vi "ADC_CHP_TEST.vi"() -> ()   [LabVIEW 2016]
uses:
  D:/share/SBND/SBND_SW/SBND_WIB_DLL/WIB_DLL/bin/Debug/WIB_DLL.dll
  SBND/SBND_SW/SBND_WIB_DLL/WIB_DLL/bin/Debug/WIB_DLL.dll
  WIB_Global.vi
  <vilib>/express/express analysis/Spectral/Block/exnSpectralBlock spectral measurements peak poly.vi
  <vilib>/express/express analysis/Spectral/Block/exnSpectralBlock spectral measurements peak DDT.vi
  <vilib>/Waveform/DTblOps.llb/DTbl Boolean Array to Digital.vi
  <vilib>/Waveform/DTblOps.llb/DTbl Append Digital Samples.vi
  <vilib>/express/express analysis/Spectral/XNode/ExpressSpectralMeasurementsBlockNode.xnode
  <vilib>/Analysis/NI_AAL_SigProc.lvlib
panel:
  out "PWR_CNTRL_\nREG 1":u32=15
  out "HCP_CHN_SEL_REG3":u32=2147484929
  out "TP_FR_DLY_REG5":u32=7996092
  out "D SHIFT_REG8":u32=33686018
  out "TP_CNTL_REG6":u32=18
  out "CLK_PHS_REG7":u32=13
  out "FE SPI":u32[](array[numeric])=[3435973836, 3435973836, 3435973836, 3435973836, 35344]
  out "ADC SPI 4":u32[](array[numeric])=[1751672936, 1751672936, 1751672936, 1751672936, 40960]
  out "ADC SPI 3":u32[](array[numeric])=[1751672936, 1751672936, 1751672936, 1751672936, 40960]
  out "ADC SPI 2":u32[](array[numeric])=[1751672936, 1751672936, 1751672936, 1751672936, 40960]
  out "ADC SPI 1":u32[](array[numeric])=[1751672936, 1751672936, 1751672936, 1751672936, 40960]
  out "receive_byte_array":u8[](array[numeric])=[1, 179, 4, 188, 0, 0, 0, 0, 0, 0, 0, 0, 240, 0, 1, 0, 250, 206, 195, 197, 161, 60, 60, 163, 51, 170, 192, 60, 61, 131, 195, 192, 200, 60, 57, 227, 83, 192, 203, 61, 60, 35, 250, 206, 163, 197, 159, 60, 60, 131, 51, 172, 187, 60, 61, 115, 195, 192, 200, 60, 57, 227, 83, 188, 203, 61, 60, 19, 250, 206, 179, 198, 162, 60, 60, 3, 51, 172, 188, 60, 61, 147, 179, 192, 200, 60, 57, 243, 83, 192, 203, 61, 60, 3, 250, 206, 163, 197, 164, 60, 60, 163, 99, 173, 192, 60, 61, 163, 179, 192, 201, 60, 57, 227, 99, 191, 203, 61, 60, 19, 250, 206, 179, 195, 164, 60, 60, 147, 51, 168, 192, 60, 61, 99, 131, 192, 200, 60, 57, 227, 51, 192, 205, 61, 60, 3, 250, 206, 163, 194, 161, 60, 60, 99, 35, 169, 189, 60, 61, 99, 147, 189, 200, 60, 57, 227, 99, 187, 203, 61, 60, 3, 250, 206, 147, 192, 159, 60, 60, 51, 51, 167, 187, 60, 61, 99, 147, 192, 200, 60, 57, 227, 83, 187, 204, 61, 60, 19, 250, 206, 147, 192, 159, 60, 60, 51, 19, 170, 190, 60, 61, 99, 179, 192, 198, 60, 57, 211, 83, 186, 203, 61, 60, 3, 250, 206, 115, 193, 158, 60, 60, 67, 19, 170, 186, 60, 61, 115, 163, 187, 200, 60, 57, 227, 83, 185, 203, 61, 60, 3, 250, 206, 131, 192, 158, 60, 60, 51, 3, 170, 186, 60, 61, 99, 163, 188, 200, 60, 58, 19, 83, 186, 203, 61, 60, 3, 250, 206, 163, 193, 159, 60, 60, 115, 3, 169, 187, 60, 61, 99, 163, 187, 200, 60, 57, 243, 51, 187, 200, 61, 60, 3, 250, 206, 179, 192, 159, 60, 60, 115, 3, 167, 188, 60, 61, 67, 179, 187, 200, 60, 57, 227, 51, 187, 200, 61, 60, 3, 250, 206, 195, 193, 162, 60, 60, 115, 19, 167, 192, 60, 61, 99, 131, 187, 199, 60, 58, 3, 115, 185, 202, 61, 60, 3, 250, 206, 163, 192, 191, 60, 60, 115, 19, 167, 192, 60, 61, 83, 147, 187, 199, 60, 57, 243, 51, 187, 203, 61, 60, 3, 250, 206, 179, 193, 159, 60, 60, 115, 19, 170, 192, 60, 61, 115, 131, 187, 197, 60, 57, 227, 51, 185, 202, 61, 59, 195, 250, 206, 179, 194, 160, 60, 60, 99, 3, 171, 192, 60, 61, 99, 131, 185, 200, 60, 57, 243, 51, 188, 200, 61, 60, 3, 250, 206, 179, 196, 160, 60, 60, 99, 3, 171, 192, 60, 61, 115, 163, 184, 198, 60, 57, 211, 83, 185, 200, 61, 60, 3, 250, 206, 163, 196, 159, 60, 60, 99, 3, 167, 192, 60, 61, 99, 131, 187, 198, 60, 57, 211, 51, 187, 200, 61, 60, 3, 250, 206, 163, 196, 161, 60, 60, 99, 3, 170, 187, 60, 61, 99, 147, 185, 198, 60, 57, 195, 35, 188, 200, 61, 60, 3, 250, 206, 131, 196, 160, 60, 60, 115, 3, 168, 192, 60, 61, 99, 131, 186, 197, 60, 57, 227, 35, 188, 200, 61, 59, 227, 250, 206, 163, 195, 160, 60, 60, 115, 3, 170, 189, 60, 61, 67, 147, 186, 197, 60, 57, 243, 35, 191, 200, 61, 59, 195, 250, 206, 131, 194, 161, 60, 60, 131, 3, 168, 192, 60, 61, 99, 131, 184, 198, 60, 57, 243, 19, 188, 201, 61, 60, 3, 250, 206, 131, 193, 159, 60, 60, 163, 3, 167, 192, 60, 61, 67, 115, 185, 198, 60, 57, 227, 19, 188, 200, 61, 59, 195, 250, 206, 67, 188, 154, 60, 60, 51, 3, 163, 185, 60, 61, 51, 83, 179, 194, 60, 57, 163, 211, 185, 198, 60, 59, 131, 250, 206, 179, 97, 64, 54, 54, 163, 83, 72, 98, 54, 55, 163, 195, 76, 104, 54, 52, 3, 35, 92, 106, 55, 53, 243, 250, 206, 242, 53, 23, 35, 35, 226, 2, 29, 54, 36, 36, 226, 162, 16, 52, 36, 33, 82, 242, 40, 61, 35, 35, 66, 250, 206, 49, 0, 213, 15, 15, 48, 160, 212, 241, 14, 16, 16, 48, 206, 247, 15, 13, 128, 0, 222, 0, 16, 14, 225, 250, 206, 32, 220, 64, 9, 5, 96, 32, 64, 123, 4, 5, 240, 64, 66, 200, 5, 5, 240, 144, 64, 158, 8, 8, 96, 250, 206, 160, 218, 40, 8, 3, 240, 208, 13, 117, 2, 3, 240, 112, 54, 201, 4, 5, 144, 32, 35, 155, 8, 8, 0, 250, 206, 192, 218, 43, 8, 3, 240, 240, 10, 119, 2, 3, 240, 128, 54, 200, 4, 5, 144, 16, 35, 155, 8, 8, 0, 250, 206, 0, 218, 60, 9, 3, 240, 96, 22, 120, 4, 3, 240, 48, 85, 201, 5, 5, 240, 128, 56, 155, 8, 8, 32, 250, 206, 192, 230, 171, 12, 12, 224, 240, 167, 203, 11, 14, 32, 96, 231, 230, 12, 12, 0, 16, 191, 216, 14, 12, 208, 250, 206, 225, 156, 123, 25, 25, 209, 113, 124, 152, 25, 27, 65, 161, 193, 176, 25, 24, 33, 65, 157, 161, 27, 25, 129, 250, 206, 98, 115, 75, 39, 39, 18, 210, 81, 106, 38, 40, 162, 34, 145, 127, 39, 37, 34, 194, 113, 118, 40, 38, 178, 250, 206, 131, 23, 236, 49, 49, 98, 2, 244, 11, 49, 50, 83, 83, 40, 32, 49, 47, 3, 131, 16, 26, 50, 48, 179, 250, 206, 3, 121, 81, 56, 55, 179, 67, 90, 110, 55, 56, 131, 179, 128, 129, 55, 53, 51, 211, 113, 128, 56, 54, 243, 250, 206, 227, 172, 132, 58, 58, 227, 67, 144, 162, 58, 59, 163, 211, 165, 174, 58, 56, 99, 3, 162, 176, 60, 58, 83, 250, 206, 67, 191, 154, 60, 60, 83, 227, 163, 182, 59, 61, 3, 67, 182, 195, 60, 57, 147, 3, 183, 196, 61, 59, 147, 250, 206, 147, 195, 159, 60, 60, 131, 19, 170, 187, 60, 61, 99, 131, 184, 201, 60, 57, 243, 83, 188, 200, 61, 60, 19] format="%x"
  out "ADC_hist":u32[][](array[numeric])
  in  "stop":bool
  in  "Tab Control":T1(tab)
  in  "RESET 6":bool
  in  "samples 3":i32
  in  "CHANNEL":u8(slide)=5
  in  "number_of_samples":u32=5000
  in  "CHIP":u8(slide)=1 scale=1.0..4.0
  in  "STOP_DATA":bool
  in  "AUTO SCALE":bool=TRUE
  in  "x":u32=72
  out "ADC_RMS":dbl=174.66413482178115
  out "ADC_MEAN":dbl=933.1157768446311
  out "ADC_CNT":u32=5001
  out "ADC_PEAK":u32=936
  out "Waveform Graph 4":u32[](graph)
  out "ADC HIST":u32[](graph)=[22577709, 0, 0, 0, 0, 0, 0, 21, 20418, 52548, 15639, 26748, 664, 1, 0, 1, 0, 0, 0, 0, 0, 0, 0, 0, 0, 0, 0, 0, 0, 0, 0, 0, 2, 0, 0, 0, 1, 7, 281, 204, 1416, 4249, 8417, 5754, 234, 46, 11, 23, 1, 0, 0, 1, 16, 23, 186, 61, 3216, 3846, 273, 944, 1470, 230, 5, 52, 23468, 0, 0, 0, 0, 0, 0, 2, 26, 205, 1131, 2487, 13823, 43022, 52991, 115617, 146273, 179719, 290128, 262476, 337032, 260069, 167100, 269246, 193925, 64886, 36955, 23917, 16001, 9314, 5817, 3963, 4270, 8627, 9126, 11227, 16105, 15657, 10840, 8925, 8975, 10027, 6845, 7402, 7674, 7135, 5371, 4730, 3238, 2959, 2574, 3198, 3582, 4566, 5614, 6190, 5902, 5590, 4229, 3018, 2633, 2873, 3587, 558800, 539267, 12817, 2, 0, 1, 0, 1, 78, 70, 55, 3, 0, 0, 0, 0, 0, 0, 0, 0, 0, 0, 0, 0, 0, 0, 28247, 761, 0, 0, 0, 0, 0, 3, 0, 0, 0, 0, 0, 1, 1, 61, 181, 563, 3580, 2716, 1620, 768, 580, 227, 15, 5, 3, 0, 7, 11, 25, 31, 40, 79, 98, 174, 226, 331, 157971, 146461, 0, 0, 0, 0, 0, 0, 0, 0, 0, 0, 0, 0, 0, 0, 0, 20, 1, 6, 75, 297, 1597, 1813, 2654, 2380, 744, 706, 26, 2, 0, 1, 1, 0, 0, 0, 0, 0, 0, 0, 0, 0, 17, 7, 0, 0, 0, 0, 0, 0, 0, 0, 0, 0, 0, 0, 0, 0, 0, 0, 0, 0, 0, 0, 268190, 65267, 235, 280, 239, 116, 42, 12, 1, 0, 1, 0, 0, 0, 0, 0, 0, 0, 0, 0, 0, 0, 0, 0, 0, 3, 0, 27989, 1018, 0, 0, 0, 0, 0, 0, 0, 0, 0, 0, 0, 0, 0, 0, 0, 0, 0, 0, 0, 0, 0, 0, 0, 0, 0, 0, 0, 0, 0, 0, 0, 0, 0, 0, 0, 348357, 468088, 0, 0, 0, 0, 0, 0, 0, 0, 0, 0, 0, 0, 0, 0, 0, 0, 0, 0, 0, 0, 0, 0, 0, 0, 0, 0, 0, 0, 0, 0, 0, 0, 0, 0, 0, 0, 0, 0, 0, 0, 0, 0, 0, 0, 0, 0, 0, 1, 0, 0, 10, 44, 151, 270, 186, 1592, 3714, 1087, 1445, 1789, 402, 33, 114418, 100521, 0, 0, 0, 0, 0, 0, 0, 0, 0, 0, 0, 0, 0, 0, 0, 0, 0, 0, 0, 0, 0, 0, 0, 0, 0, 0, 0, 0, 0, 0, 0, 0, 0, 0, 0, 0, 0, 0, 0, 0, 0, 0, 0, 0, 0, 0, 0, 0, 0, 0, 0, 0, 0, 0, 0, 0, 0, 0, 0, 0, 0, 0, 103225, 65211, 0, 0, 0, 0, 0, 0, 0, 0, 0, 0, 0, 0, 0, 0, 0, 0, 0, 0, 0, 1, 0, 0, 0, 0, 2, 474, 23148, 5367, 21546, 7315, 162, 0, 0, 0, 0, 0, 0, 0, 0, 0, 0, 0, 0, 0, 0, 0, 0, 0, 0, 0, 0, 0, 0, 0, 0, 0, 0, 0, 0, 0, 0, 0, 543916, 110849, 0, 0, 0, 0, 0, 0, 0, 0, 0, 0, 0, 0, 0, 0, 0, 64, 0, 8, 41, 168, 805, 1642, 2596, 1966, 752, 2266, 66, 39, 4270076, 0, 1, 0, 0, 0, 0, 0, 0, 0, 0, 0, 0, 0, 0, 0, 0, 0, 0, 0, 0, 0, 0, 0, 0, 0, 0, 0, 0, 0, 0, 0, 0, 0, 37524, 27901, 0, 0, 0, 0, 6, 10, 48, 66, 332, 550, 1805, 2923, 1144, 2250, 391, 902, 209, 44, 11, 0, 0, 0, 0, 3, 4281, 672, 89, 36472, 1510, 7, 15, 0, 9, 17, 33, 68, 41, 14, 5, 2, 0, 0, 0, 0, 0, 0, 0, 0, 0, 0, 0, 0, 0, 1, 12, 29, 38, 40, 16, 8, 6, 1, 186208, 374158, 15, 0, 0, 0, 0, 0, 5, 16, 34, 29, 14, 23, 14, 16, 33, 31, 18, 12, 3, 0, 0, 0, 0, 3, 0, 8, 21677, 7388, 152, 229, 257, 251, 134, 170, 204, 245, 307, 103, 52, 23, 7, 0, 0, 0, 3, 8, 35, 36, 38, 20, 10, 1, 0, 1, 11, 34, 72, 83, 40, 34, 5, 3, 539938, 221066, 133, 2, 14, 18, 29, 37, 423, 8, 8, 12, 12, 46, 46, 22, 34, 52, 30, 18, 14, 46, 103, 142, 86, 533, 8, 31, 5, 0, 3, 11, 26, 232, 42, 67, 84, 167, 169, 70, 42, 31, 60, 226, 1856, 2214, 1932, 1347, 1913, 1419, 101, 57, 23, 125, 289, 692, 1227, 1912, 3009, 2950, 2155, 1898, 1846, 1019, 145654, 187109, 2619, 1, 0, 0, 2, 14, 128, 655, 1324, 2969, 2323, 3140, 1932, 2127, 3093, 2220, 2096, 1242, 311, 28, 6, 1, 44, 296, 1396, 3357, 4125, 6543, 56916, 809, 267, 188, 282, 691, 795, 1008, 1064, 756, 423, 402, 999, 2289, 5714, 9364, 10422, 7930, 5699, 4275, 4216, 2880, 2729, 2320, 1875, 1848, 3156, 6640, 11295, 8971, 4828, 2794, 2521, 2254, 539153, 9526140, 23984, 3645, 2296, 775, 296, 85, 173, 34, 44, 41, 22, 36, 221, 423, 747, 1207, 1662, 3476, 3632, 1875, 1500, 574, 17287, 29029, 11205, 22887, 23819, 18510, 125772, 15570944, 5084400, 131401, 71234, 13143, 113780, 41764, 10472, 11394, 9741, 18907, 12744, 10109, 16912, 14081, 9050, 15252, 18972, 18097, 30210, 34499, 22914, 15704, 16962, 14793, 11397, 17017, 22006, 17454, 8162, 9019, 17249, 16759, 607898, 530261, 36183, 18775, 19842, 12497, 14104, 10165, 14844, 7410, 9392, 20172, 24755, 28710, 25853, 22888, 21117, 21210, 12128, 13154, 15918, 17977, 10914, 13293, 24423, 46723, 56516, 168221, 201926, 1224748, 932608, 1703093, 2418436, 1290130, 1081875, 1220564, 2115041, 48563549, 66978175, 81096802, 128293940, 174345980, 56717555, 6687204, 3207911, 517765, 97306, 77854, 30160, 42469, 70408, 98814, 71477, 70253, 36559, 44538, 101818, 310050, 1809711, 2451921, 347958, 395428, 108140, 6891, 210217, 1611534, 1259156, 46666, 29264, 41833, 8071, 10703, 17330, 16157, 8644, 4255, 3099, 4459, 7721, 9566, 11907, 11073, 10813, 12608, 21489, 38723, 51966, 68269, 84538, 69440, 17462, 11299, 5029, 3258, 215986, 99753, 66565, 117594, 123569, 9000, 112656, 4859, 1648, 1607, 1064, 1125, 1192, 7668, 9736, 8534, 6905, 5548, 1375, 649, 667, 846, 1826, 3073, 4290, 5127, 5994, 11408, 3783, 2185, 3925, 1156, 831, 490, 544570, 271572, 72151, 10036, 10374, 13581, 11554, 10053, 10605, 4507, 5529, 11858, 3179, 973, 475, 1232, 3805, 5899, 5322, 7517, 5860, 5148, 4434, 7330, 6653, 8150, 5089, 7730, 24174, 22294, 211500, 148381, 98471, 182664, 91351, 656, 229017, 70281, 53148, 950, 33846, 945, 620, 460, 1469, 2995, 3740, 2697, 3829, 3305, 452, 736, 58, 44, 4, 6, 10, 27, 13, 35, 67, 72, 186, 234, 54221, 83063, 2258, 2331, 5555, 548, 1421, 80, 198, 22, 8, 4, 16, 357, 1586, 1901, 1928, 914, 1246, 1207, 1834, 2347, 1744, 651, 118, 37, 0, 0, 0, 4, 9031, 141640, 280332, 295916, 115759, 6648, 4525, 4918, 925, 453, 296, 902, 1039, 2591, 3442, 2825, 182, 66, 197, 281, 274, 115, 57, 15, 0, 0, 0, 2, 0, 2, 0, 6, 23, 43, 97065, 560497, 177, 34, 47, 25, 4, 1, 33, 0, 0, 2, 6, 37, 30, 23, 35, 4, 45, 53, 61, 60, 73, 54, 15, 8, 1, 0, 0, 0, 0, 1, 1, 23, 370649, 132, 153619, 135316, 143, 131, 45, 87, 436, 178, 183, 99, 24, 1, 0, 0, 3, 25, 55, 93, 58, 310, 121, 43, 160, 16, 0, 0, 2, 17, 60446, 169610, 333, 0, 0, 0, 0, 0, 0, 0, 1, 2, 2, 10, 24, 24, 38, 9, 32, 9, 2, 13, 30, 42, 34, 36, 17, 0, 0, 0, 0, 2, 29007, 16, 9, 34, 65, 47, 21, 6, 4, 3, 33, 51, 60, 71, 216, 407, 1423, 2777, 1256, 2544, 319, 1291, 27, 10, 9, 4, 0, 0, 0, 0, 2, 5, 44882, 27803, 185, 0, 0, 0, 0, 0, 0, 0, 0, 0, 0, 0, 0, 0, 0, 0, 0, 0, 0, 0, 0, 0, 0, 0, 0, 0, 0, 0, 0, 0, 0, 0, 0, 0, 0, 0, 0, 0, 0, 0, 0, 0, 0, 0, 0, 0, 0, 0, 0, 0, 0, 0, 0, 0, 0, 0, 0, 0, 0, 0, 0, 0, 50022, 355826, 0, 0, 0, 0, 0, 0, 0, 0, 0, 0, 0, 0, 0, 0, 0, 0, 0, 0, 0, 0, 0, 0, 0, 0, 0, 0, 0, 0, 0, 0, 0, 0, 0, 0, 0, 0, 0, 0, 0, 0, 0, 0, 0, 0, 0, 0, 0, 0, 0, 0, 0, 0, 0, 0, 0, 0, 0, 0, 0, 0, 0, 0, 148638, 196913, 0, 0, 0, 0, 0, 0, 0, 0, 0, 0, 0, 0, 0, 0, 0, 0, 0, 0, 0, 0, 0, 0, 0, 0, 0, 0, 0, 0, 0, 0, 0, 0, 0, 0, 0, 0, 0, 0, 0, 0, 0, 0, 0, 0, 0, 0, 0, 0, 0, 0, 0, 0, 0, 0, 0, 0, 0, 0, 0, 0, 0, 0, 304803, 63193, 0, 0, 0, 0, 0, 0, 0, 0, 0, 0, 0, 0, 0, 0, 0, 0, 0, 0, 0, 0, 0, 0, 0, 0, 0, 0, 0, 0, 0, 0, 0, 0, 0, 0, 0, 0, 0, 0, 0, 0, 0, 0, 0, 0, 0, 0, 0, 0, 0, 0, 0, 0, 0, 0, 0, 2872, 0, 0, 0, 0, 0, 0, 24503, 122552, 0, 0, 0, 0, 0, 0, 0, 0, 0, 0, 0, 0, 0, 0, 0, 0, 0, 0, 0, 0, 0, 0, 0, 0, 0, 0, 0, 0, 0, 0, 1, 29005, 0, 0, 0, 0, 0, 0, 0, 0, 0, 0, 0, 0, 0, 0, 0, 5, 0, 0, 2, 94, 134, 367, 118, 4775, 3317, 208, 556, 662, 66, 4, 12854, 29829, 1, 0, 0, 0, 0, 0, 86, 3, 19, 87, 189, 240, 250, 32, 15, 2, 1, 0, 1, 0, 0, 0, 0, 0, 0, 0, 0, 0, 0, 0, 0, 0, 0, 0, 0, 0, 0, 0, 0, 0, 0, 0, 0, 0, 0, 0, 0, 0, 0, 0, 0, 0, 0, 0, 0, 0, 0, 0, 0, 0, 0, 0, 9597, 26948, 0, 0, 0, 0, 0, 0, 0, 0, 0, 0, 0, 0, 0, 0, 0, 0, 0, 0, 0, 0, 0, 0, 0, 0, 0, 0, 0, 0, 0, 0, 0, 29004, 2, 0, 0, 0, 0, 0, 0, 0, 1, 0, 0, 0, 0, 0, 0, 0, 0, 0, 0, 0, 0, 0, 0, 0, 0, 0, 0, 0, 0, 0, 9296, 232533, 0, 0, 0, 0, 0, 0, 0, 0, 0, 0, 0, 0, 0, 0, 0, 0, 0, 0, 0, 0, 0, 0, 0, 0, 0, 0, 0, 0, 0, 0, 0, 0, 0, 0, 0, 0, 0, 0, 0, 0, 0, 0, 0, 0, 0, 0, 0, 0, 0, 0, 0, 0, 0, 0, 2, 15, 175, 203, 494, 2344, 3342, 938, 12604, 116970, 25, 5, 0, 0, 0, 0, 0, 0, 0, 0, 0, 0, 0, 0, 0, 0, 0, 0, 0, 0, 0, 0, 0, 0, 0, 0, 0, 0, 0, 0, 0, 0, 0, 0, 0, 0, 0, 0, 0, 0, 0, 0, 0, 0, 0, 0, 0, 0, 0, 0, 0, 0, 0, 0, 0, 0, 0, 0, 0, 0, 0, 0, 92278, 206268, 0, 0, 0, 0, 0, 0, 0, 0, 0, 0, 0, 0, 0, 0, 0, 0, 0, 0, 0, 0, 0, 0, 0, 0, 0, 0, 0, 0, 0, 0, 0, 0, 0, 0, 0, 0, 0, 0, 0, 0, 0, 0, 0, 0, 0, 0, 0, 0, 0, 0, 0, 0, 0, 0, 0, 0, 0, 0, 0, 0, 0, 0, 44518, 51696, 0, 0, 0, 0, 0, 0, 0, 0, 0, 0, 0, 0, 0, 0, 0, 0, 0, 0, 0, 0, 0, 0, 0, 0, 0, 0, 0, 0, 0, 0, 0, 0, 0, 0, 0, 0, 0, 0, 0, 0, 0, 0, 0, 0, 0, 0, 0, 0, 0, 0, 0, 0, 0, 0, 0, 50, 1, 0, 0, 0, 0, 0, 15879, 62858, 0, 0, 0, 0, 0, 0, 0, 0, 0, 0, 0, 0, 0, 0, 0, 0, 0, 0, 0, 0, 0, 0, 0, 0, 0, 0, 0, 0, 0, 0, 0, 0, 23, 307, 28543, 133, 0, 0, 0, 0, 0, 0, 0, 0, 0, 0, 0, 0, 0, 0, 0, 0, 0, 0, 0, 0, 0, 0, 0, 0, 0, 0, 48629, 97378, 0, 2, 12, 1, 13, 124, 363, 1882, 2761, 2632, 1683, 452, 145, 27, 153, 0, 0, 0, 0, 0, 0, 0, 0, 0, 0, 0, 0, 0, 0, 0, 0, 0, 0, 0, 0, 0, 0, 0, 0, 0, 0, 0, 0, 0, 0, 0, 0, 0, 0, 0, 0, 0, 0, 0, 0, 0, 0, 0, 0, 0, 0, 0, 182370, 13611, 0, 0, 0, 0, 0, 0, 0, 0, 0, 0, 0, 0, 0, 0, 0, 0, 0, 0, 0, 0, 0, 0, 0, 0, 0, 0, 0, 0, 0, 0, 0, 0, 0, 0, 0, 0, 0, 0, 0, 0, 0, 0, 0, 0, 0, 0, 0, 0, 0, 0, 0, 0, 0, 0, 0, 0, 0, 0, 0, 0, 0, 0, 15545, 11648, 0, 0, 0, 0, 0, 0, 0, 0, 0, 0, 0, 0, 0, 0, 0, 0, 0, 0, 0, 0, 0, 0, 0, 0, 0, 0, 0, 0, 0, 0, 0, 0, 0, 0, 0, 0, 0, 0, 0, 0, 0, 0, 0, 0, 0, 0, 0, 0, 0, 0, 0, 0, 0, 0, 0, 0, 0, 0, 0, 0, 0, 0, 46428, 23927, 0, 0, 0, 0, 0, 0, 0, 0, 0, 0, 0, 0, 0, 0, 0, 0, 0, 0, 0, 0, 0, 0, 0, 0, 0, 0, 0, 0, 0, 0, 0, 0, 0, 0, 0, 0, 0, 0, 0, 0, 14, 5, 0, 0, 0, 0, 0, 0, 0, 0, 0, 0, 0, 0, 0, 0, 0, 0, 0, 0, 0, 0, 282874, 312757, 6, 0, 0, 0, 0, 0, 0, 0, 0, 0, 0, 0, 0, 0, 0, 1, 0, 0, 0, 0, 0, 0, 0, 0, 0, 0, 0, 0, 0, 0, 0, 0, 0, 0, 0, 0, 0, 0, 0, 0, 0, 0, 0, 0, 0, 0, 0, 0, 0, 0, 0, 0, 0, 0, 0, 0, 0, 0, 0, 0, 0, 0, 10038, 189855, 0, 0, 0, 0, 0, 0, 0, 0, 0, 0, 0, 0, 0, 0, 0, 0, 0, 0, 0, 0, 0, 0, 0, 0, 0, 0, 0, 0, 0, 0, 0, 0, 0, 0, 0, 0, 0, 0, 0, 0, 0, 0, 0, 0, 0, 0, 0, 0, 0, 0, 0, 0, 0, 0, 0, 0, 0, 0, 0, 0, 0, 0, 5636, 51609, 0, 0, 0, 0, 0, 0, 0, 0, 0, 0, 0, 0, 0, 0, 0, 0, 0, 0, 0, 0, 0, 0, 0, 0, 0, 0, 0, 0, 0, 4, 11, 19, 12, 13, 27, 49, 41, 59, 4298, 19373, 0, 0, 0, 0, 0, 0, 0, 1, 0, 0, 1, 6, 4, 3991, 10, 3156, 0, 2, 10, 0, 0, 0, 9926, 64268, 0, 0, 0, 0, 0, 0, 0, 0, 0, 0, 0, 0, 0, 0, 0, 0, 0, 0, 0, 0, 0, 0, 0, 0, 0, 0, 0, 0, 0, 1293, 3795, 12, 0, 0, 0, 13395, 10568, 290, 4753, 0, 0, 0, 0, 0, 0, 0, 0, 0, 0, 0, 0, 0, 0, 0, 0, 0, 0, 0, 0, 0, 0, 0, 11479, 95493, 0, 0, 0, 0, 0, 0, 0, 0, 0, 0, 0, 0, 0, 0, 0, 6, 0, 0, 0, 0, 0, 2, 15, 192, 828, 2618, 1718, 1754, 1878, 726, 563, 45, 16, 129, 326, 1885, 1524, 2929, 1018, 1280, 509, 455, 217, 4, 0, 0, 0, 0, 0, 0, 0, 0, 0, 0, 0, 6, 0, 0, 0, 0, 0, 2, 92982, 29939, 0, 0, 0, 0, 0, 0, 0, 0, 0, 0, 0, 0, 0, 0, 0, 0, 0, 0, 0, 0, 0, 0, 0, 0, 0, 0, 0, 0, 0, 0, 0, 0, 0, 0, 0, 0, 0, 0, 0, 0, 0, 0, 0, 0, 0, 0, 0, 0, 0, 0, 0, 0, 0, 0, 0, 0, 0, 0, 0, 0, 0, 0, 46979, 14255, 0, 0, 0, 0, 0, 0, 0, 0, 0, 0, 0, 0, 0, 0, 0, 0, 0, 0, 0, 0, 0, 0, 0, 0, 0, 0, 0, 2, 4, 32, 100, 8260, 19163, 205899, 332365, 335911, 57084, 188161, 39724, 1994, 118, 4764, 1068, 392, 400, 1032, 239, 365, 405, 509, 181, 585, 270, 245, 171, 418, 163, 182, 305, 497, 440, 267, 47466, 94800, 47, 0, 0, 0, 0, 0, 0, 0, 0, 0, 0, 0, 0, 0, 0, 0, 0, 0, 0, 0, 0, 0, 0, 0, 0, 0, 0, 0, 0, 0, 0, 0, 0, 0, 0, 0, 0, 0, 0, 0, 0, 0, 0, 0, 0, 0, 0, 0, 0, 0, 0, 0, 0, 0, 0, 0, 0, 0, 0, 0, 0, 0, 184863, 255979, 0, 0, 0, 0, 0, 0, 0, 0, 0, 0, 0, 0, 0, 0, 0, 0, 0, 0, 0, 0, 0, 0, 0, 0, 0, 0, 0, 0, 0, 0, 0, 0, 0, 0, 0, 0, 0, 0, 0, 0, 0, 0, 0, 0, 0, 0, 0, 0, 0, 0, 0, 0, 0, 0, 0, 3156, 0, 0, 0, 0, 0, 0, 16079, 233706, 0, 0, 0, 0, 0, 0, 0, 0, 0, 0, 0, 0, 0, 0, 0, 0, 0, 0, 0, 0, 0, 0, 0, 0, 0, 0, 0, 0, 0, 0, 0, 0, 6, 4, 5, 5, 4, 3, 11, 28931, 0, 0, 0, 0, 0, 0, 0, 0, 0, 0, 0, 0, 0, 0, 0, 665, 0, 0, 0, 0, 0, 0, 328595, 89292, 36, 0, 0, 0, 0, 0, 0, 0, 0, 0, 0, 0, 0, 0, 0, 0, 0, 0, 0, 0, 0, 0, 0, 0, 0, 0, 0, 0, 0, 0, 0, 1, 34, 2, 27751, 1255, 0, 0, 0, 0, 0, 0, 0, 0, 0, 0, 0, 0, 0, 0, 0, 0, 0, 0, 0, 5, 27, 7, 23, 17, 3, 2, 20923, 113008, 101, 10, 3, 0, 0, 0, 0, 0, 0, 0, 0, 0, 0, 0, 0, 0, 0, 0, 0, 0, 0, 0, 0, 0, 0, 0, 0, 0, 0, 0, 0, 0, 0, 0, 0, 0, 0, 0, 0, 0, 0, 1, 31, 102, 226, 348, 1710, 1959, 877, 3349, 609, 968, 29, 27, 23, 17, 0, 0, 0, 0, 0, 6, 149571, 516166, 46546, 4192, 2157, 2291, 2062, 1763, 860, 369, 173, 134, 67, 16, 5, 0, 0, 0, 0, 0, 0, 0, 0, 0, 0, 0, 0, 0, 0, 0, 0, 0, 0, 0, 0, 0, 0, 0, 0, 0, 0, 0, 0, 0, 0, 0, 0, 0, 0, 0, 0, 0, 0, 0, 0, 0, 0, 0, 0, 0, 0, 0, 0, 0, 330, 94, 0, 0, 0, 0, 0, 0, 0, 0, 0, 0, 0, 0, 0, 0, 0, 0, 0, 0, 0, 0, 0, 0, 0, 0, 0, 0, 0, 0, 0, 0, 0, 0, 0, 0, 0, 0, 0, 0, 0, 0, 0, 0, 0, 0, 0, 0, 0, 0, 0, 0, 0, 0, 0, 0, 0, 0, 0, 0, 0, 0, 0, 0, 342, 578, 0, 0, 0, 0, 0, 0, 0, 0, 0, 0, 0, 0, 0, 0, 0, 0, 0, 0, 0, 0, 0, 0, 0, 0, 0, 0, 0, 0, 0, 0, 0, 0, 0, 0, 0, 0, 0, 0, 0, 0, 0, 0, 0, 0, 0, 0, 0, 0, 0, 0, 0, 0, 0, 0, 0, 0, 0, 0, 0, 0, 0, 0, 1159, 1, 0, 0, 0, 0, 0, 0, 0, 0, 0, 0, 0, 0, 0, 0, 0, 0, 0, 0, 0, 0, 0, 0, 0, 0, 0, 0, 0, 0, 0, 0, 0, 0, 0, 0, 0, 0, 0, 0, 0, 0, 19, 9, 0, 0, 0, 0, 0, 0, 0, 0, 0, 0, 0, 0, 0, 0, 0, 0, 0, 0, 0, 0, 1486, 1, 0, 0, 0, 0, 0, 0, 0, 0, 0, 0, 0, 0, 0, 0, 0, 0, 1, 0, 0, 0, 0, 0, 0, 0, 0, 0, 0, 0, 0, 0, 0, 0, 0, 0, 0, 0, 0, 0, 0, 0, 0, 0, 0, 0, 0, 0, 0, 0, 0, 0, 0, 0, 0, 0, 0, 0, 0, 0, 0, 0, 0, 0, 1939, 3175, 0, 0, 0, 0, 0, 0, 0, 0, 0, 0, 0, 0, 0, 0, 0, 0, 0, 0, 0, 0, 0, 0, 0, 0, 0, 0, 0, 0, 0, 0, 0, 0, 0, 0, 0, 0, 0, 0, 0, 0, 0, 0, 0, 0, 0, 0, 0, 0, 0, 0, 0, 0, 0, 0, 0, 0, 0, 0, 0, 0, 0, 0, 1379, 1262, 0, 0, 0, 0, 0, 0, 0, 0, 0, 0, 0, 0, 0, 0, 0, 0, 0, 0, 0, 0, 0, 0, 0, 0, 0, 0, 0, 0, 0, 0, 0, 0, 0, 0, 0, 0, 0, 0, 0, 0, 0, 0, 0, 0, 0, 0, 0, 0, 0, 0, 0, 0, 0, 0, 0, 0, 0, 0, 0, 0, 0, 0, 1052, 854, 0, 0, 0, 0, 0, 0, 0, 0, 0, 0, 0, 0, 0, 0, 0, 0, 0, 0, 0, 0, 0, 0, 0, 0, 0, 0, 0, 0, 0, 0, 0, 0, 0, 0, 0, 0, 0, 0, 0, 0, 0, 0, 0, 0, 0, 0, 0, 0, 0, 0, 0, 0, 0, 0, 0, 0, 0, 0, 0, 0, 0, 0, 12072, 3568, 0, 0, 0, 0, 0, 0, 0, 0, 0, 0, 0, 0, 0, 0, 0, 0, 0, 0, 0, 0, 0, 0, 0, 0, 0, 0, 0, 0, 0, 0, 0, 0, 0, 0, 0, 0, 0, 0, 0, 0, 0, 0, 0, 0, 0, 0, 0, 0, 0, 0, 0, 0, 0, 0, 0, 0, 0, 0, 0, 0, 0, 0, 5930, 5084, 0, 0, 0, 0, 0, 0, 0, 0, 0, 0, 0, 0, 0, 0, 0, 0, 0, 0, 0, 0, 0, 0, 0, 0, 0, 0, 0, 0, 0, 0, 0, 0, 0, 0, 0, 0, 0, 0, 0, 0, 0, 0, 0, 0, 0, 0, 0, 0, 0, 0, 0, 0, 0, 0, 0, 0, 0, 0, 0, 0, 0, 0, 1087, 11747, 0, 0, 0, 0, 0, 0, 0, 0, 0, 0, 0, 0, 0, 0, 0, 1, 0, 0, 0, 7, 0, 0, 0, 8, 0, 0, 0, 11, 0, 0, 0, 19, 0, 0, 0, 4, 0, 0, 0, 1, 0, 0, 0, 0, 0, 0, 0, 0, 0, 0, 0, 0, 0, 0, 0, 0, 0, 0, 0, 0, 0, 0, 899, 3837, 0, 0, 0, 0, 0, 0, 0, 0, 0, 0, 0, 0, 0, 0, 0, 0, 0, 0, 0, 0, 0, 0, 0, 0, 0, 0, 0, 0, 0, 0, 0, 0, 0, 0, 0, 0, 0, 0, 0, 0, 0, 0, 0, 0, 0, 0, 0, 0, 0, 0, 0, 0, 0, 0, 0, 0, 0, 0, 0, 0, 0, 0, 1305, 1659, 0, 0, 0, 0, 0, 0, 0, 0, 0, 0, 0, 0, 0, 0, 0, 0, 0, 0, 0, 0, 0, 0, 0, 0, 0, 0, 0, 0, 0, 0, 0, 0, 0, 0, 0, 0, 0, 0, 0, 0, 0, 0, 0, 0, 0, 0, 0, 0, 0, 0, 0, 0, 0, 0, 0, 0, 0, 0, 0, 0, 0, 0, 860, 1, 0, 0, 0, 0, 0, 0, 0, 0, 0, 0, 0, 0, 0, 0, 0, 0, 0, 0, 0, 0, 0, 0, 0, 0, 0, 0, 0, 0, 0, 0, 0, 0, 0, 0, 0, 0, 0, 0, 0, 0, 0, 0, 0, 0, 0, 0, 0, 0, 0, 0, 0, 0, 0, 0, 0, 0, 0, 0, 0, 0, 0, 0, 1, 0, 0, 0, 0, 0, 0, 0, 0, 0, 0, 0, 0, 0, 0, 0, 0, 0, 0, 0, 0, 0, 0, 0, 0, 0, 0, 0, 0, 0, 0, 0, 0, 0, 0, 0, 0, 0, 0, 0, 0, 0, 0, 0, 0, 0, 0, 0, 0, 0, 0, 0, 0, 0, 0, 0, 0, 0, 0, 0, 0, 0, 0, 0, 0, 674, 1, 0, 0, 0, 0, 0, 0, 0, 0, 0, 0, 0, 0, 0, 0, 0, 0, 0, 0, 0, 0, 0, 0, 0, 0, 0, 0, 0, 0, 0, 0, 0, 0, 0, 0, 0, 0, 0, 0, 0, 0, 0, 0, 0, 0, 0, 0, 0, 0, 0, 0, 0, 0, 0, 0, 0, 0, 0, 0, 0, 0, 0, 77598]
  out "samples 4":u32=671013472
  in  "FILE PATH":path=path "C:/Users/jfried/Desktop/New folder (11)"
  in  "FILE NAME 2":string="1459002fff"
  in  "SAVE TO \nFILE":bool
  out "Store_Data":bool
  out "x = y? 5":bool=TRUE
  out "HEX":u32=928 format="%x"
  in  "Tab Control 3":T2(tab)
  in  "length":i32=29 min=10 max=65 step=1
  in  "Tab Control 5":enum32{"ADC SYNC", "UDP CONTROL"}(tab)=enum."UDP CONTROL"
  out "100MHZ":bool
  out "200MHZ  ON":bool=TRUE
  in  "ADC  CLK \nPHASE 2":bool[](array[boolean])=[FALSE, FALSE, FALSE, TRUE, FALSE, FALSE, FALSE, FALSE]
  in  "DATA SHIFT 2":u8[](array[numeric])=[0, 0, 0, 0, 0, 0, 0, 1] format="%x"
  in  "ADC  CLK \nPHASE":bool[](array[boolean])=[TRUE, FALSE, TRUE, TRUE, FALSE, FALSE, FALSE, FALSE]
  in  "TEST PAT EN":bool
  in  "TEST PAT":u16=18 format="%x"
  in  "DATA SHIFT":u8[](array[numeric])=[2, 2, 2, 2, 0, 0, 0, 1] format="%x"
  in  "100MHz/\n200MHz":bool
  out "SYNC 2":u8=240 format="%08b"
  in  "DATA 9":u32=15 format="%x"
  in  "ADDRESS 6":u16=1
  in  "UDP WRITE 2":bool
  in  "ADDRESS 5":u16=1
  out "DATA 8":u32 format="%x"
  in  "UDP READ 2":bool
  in  "WIB MODE":bool=TRUE
  in  "ASIC/CHN READOUT":bool=TRUE
  out "Waveform Graph 6":u32[](graph)=[927, 927, 927, 926, 927, 926, 927, 926, 926, 927, 930, 1124, 1789, 2599, 3058, 3008, 2591, 2059, 1592, 1266, 1074, 978, 940, 930, 929, 930, 931, 930, 930]
  in  "FPGA DAC":bool
  in  "ASIC DAC":bool
  in  "AMPL":u16=24576 format="%x"
  in  "DLY":u16=122
  in  "FREQ":u16=700
  in  "MODE":u16(slide)=4 scale format="%.6p"
  out "Waveform Graph 5":u32[](graph)=[927, 927, 927, 926, 927, 926, 927, 926, 926, 927, 930, 1124, 1789, 2599, 3058, 3008, 2591, 2059, 1592, 1266, 1074, 978, 940, 930, 929, 930, 931, 930, 930]
  in  "MULT":dbl=1.0 min=1.0
  out "CLOCK 2":dbl=5e-09
  in  "CLOCK":dbl=5e-09
  in  "IDL_OFF2":dbl=4.500000000000002e-07 caption="OFFSET" min=0.0 max=0.000655 step=1e-08 format="%#_6p"
  in  "IDL_WID2":dbl=5e-08 caption="WIDTH" min=0.0 max=0.000655 step=1e-08 format="%#_6p"
  in  "I_IDL":bool caption="INVERT"
  in  "IDL_WID1":dbl=1.5999999999999995e-07 caption="WIDTH" min=0.0 max=0.000655 step=1e-08 format="%#_6p"
  in  "IDL_OFF1":dbl=5e-08 caption="OFFSET" min=0.0 max=0.000655 step=1e-08 format="%#_6p"
  out "INV_REG":u32=50529027
  in  "OK Button 4":bool
  in  "I_IDXL":bool caption="invert"
  in  "I_IDXM":bool caption="invert"
  in  "I_READ":bool=TRUE caption="invert"
  in  "I_RST":bool=TRUE caption="invert"
  in  "IDXL_WID":dbl=4.999999999999999e-08 caption="WIDTH" min=0.0 max=0.000655 step=5e-09 format="%#_6p"
  in  "IDXL_OFF":dbl=4.4999999999999993e-07 caption="OFFSET" min=0.0 max=0.000655 step=5e-09 format="%#_6p"
  in  "IDXM_WID":dbl=3e-07 caption="WIDTH" min=0.0 max=0.000655 step=5e-09 format="%#_6p"
  in  "IDXM_OFF":dbl=2e-07 caption="OFFSET" min=0.0 max=0.000655 step=5e-09 format="%#_6p"
  in  "READ_WID":dbl=3.000000000000002e-08 caption="WIDTH" min=0.0 max=0.000655 step=5e-09 format="%#_6p"
  in  "READ_OFF":dbl=4.600000000000003e-07 caption="OFFSET" min=0.0 max=0.000655 step=5e-09 format="%#_6p"
  in  "RST_WID":dbl=5e-08 caption="WIDTH" min=0.0 max=0.000655 step=5e-09 format="%#_6p"
  in  "RST_OFF":dbl caption="OFFSET" min=0.0 max=0.000655 step=5e-09 format="%#_6p"
  in  "PERIOD":dbl=5e-07 min=1e-08 max=0.000655 step=1e-08 format="%#_6p"
  out "Mixed Signal Graph":digitaldata(graph)
  in  "CLOCK DISABLE":bool
  out "PLL1 in = out":bool=TRUE
  in  "C0":u16
  in  "C1":u16
  out "PLL1_in":u32 format="%x"
  out "PLL1_out":u32 format="%x"
  in  "C3":u16=2
  in  "C2":u16=1
  out "PLL1_in 2":u32=131073 format="%x"
  out "PLL1 in = out 2":bool=TRUE
  out "PLL1_out 2":u32=131073 format="%x"
  out "PLL1_in 3":u32 format="%x"
  in  "C0 2":bool
  in  "C4":bool
  in  "C3 2":bool
  in  "C2 2":bool
  in  "C1 2":bool
  in  "C4 2":u16 caption="C4"
  out "PLL1 in = out 3":bool=TRUE
  out "PLL1_out 3":u32 format="%x"
  out "set_ind":bool
  in  "Set Phase ADC 1":bool
  in  "C0 3":u16 caption="C0"
  in  "C1 3":u16 caption="C1"
  out "PLL1_in 4":u32 format="%x"
  out "PLL1_out 4":u32 format="%x"
  out "PLL1 in = out 4":bool=TRUE
  in  "C3 3":u16=2 caption="C3"
  in  "C2 3":u16=1 caption="C2"
  out "PLL1_in 5":u32=131073 format="%x"
  out "PLL1 in = out 5":bool=TRUE
  out "PLL1_out 5":u32=131073 format="%x"
  out "PLL1_in 6":u32 format="%x"
  in  "C0 4":bool
  in  "C4 3":bool
  in  "C3 4":bool
  in  "C2 4":bool
  in  "C1 4":bool
  in  "C4 4":u16 caption="C4"
  out "PLL1 in = out 6":bool=TRUE
  out "PLL1_out 6":u32 format="%x"
  out "set_ind 2":bool
  in  "Set Phase ADC 2":bool
  in  "C0 5":u16 caption="C0"
  in  "C1 5":u16 caption="C1"
  out "PLL1_in 7":u32 format="%x"
  out "PLL1_out 7":u32 format="%x"
  out "PLL1 in = out 7":bool=TRUE
  in  "C3 5":u16=2 caption="C3"
  in  "C2 5":u16=1 caption="C2"
  out "PLL1_in 8":u32=131073 format="%x"
  out "PLL1 in = out 8":bool=TRUE
  out "PLL1_out 8":u32=131073 format="%x"
  out "PLL1_in 9":u32 format="%x"
  in  "C0 6":bool
  in  "C4 5":bool
  in  "C3 6":bool
  in  "C2 6":bool
  in  "C1 6":bool
  in  "C4 6":u16 caption="C4"
  out "PLL1 in = out 9":bool=TRUE
  out "PLL1_out 9":u32 format="%x"
  out "set_ind 3":bool
  in  "Set Phase ADC 3":bool
  out "Waveform Graph":dynamicdata(graph)=[{"t0"=timestamp(0 s since 1904-01-01), "dt"=399.9200159968007, "Y"=array[2501 elements], "attributes"=variant("NI_ChannelName"=variant(string "FFT - (Peak)"))}]
  in  "ENABLE FFT":bool=TRUE
  in  "RESET FFT":bool
  out "BUS VOL":dbl[](array[numeric])=[1.78875, 1.7862500000000001, 1.7925, 1.7825, 1.7875, 1.7925] format="%#_4p"
  out "SHUNT VOL":dbl[](array[numeric])=[0.0031125000000000002, 0.0023125000000000003, 0.00237, 0.0053750000000000004, 0.005580000000000001, 0.0031025000000000002] format="%#_4p"
  in  "Boolean":bool
  out "BUS VOL 2":dbl[](array[numeric])=[1.7962500000000001, 1.78875, 1.7875, 1.7862500000000001, 1.78875, 1.7875] format="%#_4p"
  out "SHUNT VOL 2":dbl[](array[numeric])=[0.0032575000000000004, 0.0021750000000000003, 0.0020475000000000003, 0.0055325, 0.005602500000000001, 0.0032050000000000004] format="%#_4p"
  in  "PWR SCK 1":bool=TRUE
  in  "channel":T3={"sts"=TRUE, "snc"=TRUE, "SG"=0, "ST"=3, "SDC"=FALSE, "SDF"=FALSE} {"ST" items=["0.5us"=1, "1us"=0, "2us"=3, "3us"=2]; "SG" items=["4.7 mV/fC", "7.8 mV/fC", "14 mV/fC", "25 mV/fC"]}
  in  "s 11":bool=TRUE
  in  "write_string":bool
  in  "OK Button 2":bool
  in  "Slide":u8(slide) scale=0.0..3.0
  in  "CHANNEL 4":T4={"D_offset"=6, "PDSR"=FALSE, "PCSR"=TRUE, "slp"=FALSE, "tst"=FALSE} {"D_offset" items=["0", "1", "2", "3", "4", "5", "6", "7", "8", "9", "10", "11", "12", "13", "14", "15"]}
  in  "QUICK SET":bool
  in  "s 10":bool=TRUE
  in  "s 9":bool=TRUE
  in  "s 8":bool=TRUE
  in  "s 7":bool=TRUE
  in  "s 6":bool=TRUE
  in  "s 5":bool=TRUE
  in  "s 4":bool=TRUE
  in  "s 3":bool=TRUE
  in  "s 2":bool=TRUE
  in  "s":bool=TRUE
  in  "CHANNEL 3":T5(array[cluster])=[[{"D_offset"=6, "PDSR"=FALSE, "PCSR"=TRUE, "slp"=FALSE, "tst"=FALSE}, {"D_offset"=6, "PDSR"=FALSE, "PCSR"=TRUE, "slp"=FALSE, "tst"=FALSE}, {"D_offset"=6, "PDSR"=FALSE, "PCSR"=TRUE, "slp"=FALSE, "tst"=FALSE}, {"D_offset"=6, "PDSR"=FALSE, "PCSR"=TRUE, "slp"=FALSE, "tst"=FALSE}, {"D_offset"=0, "PDSR"=TRUE, "PCSR"=TRUE, "slp"=FALSE, "tst"=FALSE}, {"D_offset"=0, "PDSR"=TRUE, "PCSR"=TRUE, "slp"=FALSE, "tst"=FALSE}, {"D_offset"=0, "PDSR"=TRUE, "PCSR"=TRUE, "slp"=FALSE, "tst"=FALSE}, {"D_offset"=0, "PDSR"=TRUE, "PCSR"=TRUE, "slp"=FALSE, "tst"=FALSE}], [{"D_offset"=6, "PDSR"=FALSE, "PCSR"=TRUE, "slp"=FALSE, "tst"=FALSE}, {"D_offset"=6, "PDSR"=FALSE, "PCSR"=TRUE, "slp"=FALSE, "tst"=FALSE}, {"D_offset"=6, "PDSR"=FALSE, "PCSR"=TRUE, "slp"=FALSE, "tst"=FALSE}, {"D_offset"=6, "PDSR"=FALSE, "PCSR"=TRUE, "slp"=FALSE, "tst"=FALSE}, {"D_offset"=0, "PDSR"=TRUE, "PCSR"=TRUE, "slp"=FALSE, "tst"=FALSE}, {"D_offset"=0, "PDSR"=TRUE, "PCSR"=TRUE, "slp"=FALSE, "tst"=FALSE}, {"D_offset"=0, "PDSR"=TRUE, "PCSR"=TRUE, "slp"=FALSE, "tst"=FALSE}, {"D_offset"=0, "PDSR"=TRUE, "PCSR"=TRUE, "slp"=FALSE, "tst"=FALSE}], [{"D_offset"=6, "PDSR"=FALSE, "PCSR"=TRUE, "slp"=FALSE, "tst"=FALSE}, {"D_offset"=6, "PDSR"=FALSE, "PCSR"=TRUE, "slp"=FALSE, "tst"=FALSE}, {"D_offset"=6, "PDSR"=FALSE, "PCSR"=TRUE, "slp"=FALSE, "tst"=FALSE}, {"D_offset"=6, "PDSR"=FALSE, "PCSR"=TRUE, "slp"=FALSE, "tst"=FALSE}, {"D_offset"=0, "PDSR"=TRUE, "PCSR"=TRUE, "slp"=FALSE, "tst"=FALSE}, {"D_offset"=0, "PDSR"=TRUE, "PCSR"=TRUE, "slp"=FALSE, "tst"=FALSE}, {"D_offset"=0, "PDSR"=TRUE, "PCSR"=TRUE, "slp"=FALSE, "tst"=FALSE}, {"D_offset"=0, "PDSR"=TRUE, "PCSR"=TRUE, "slp"=FALSE, "tst"=FALSE}], [{"D_offset"=6, "PDSR"=FALSE, "PCSR"=TRUE, "slp"=FALSE, "tst"=FALSE}, {"D_offset"=6, "PDSR"=FALSE, "PCSR"=TRUE, "slp"=FALSE, "tst"=FALSE}, {"D_offset"=6, "PDSR"=FALSE, "PCSR"=TRUE, "slp"=FALSE, "tst"=FALSE}, {"D_offset"=6, "PDSR"=FALSE, "PCSR"=TRUE, "slp"=FALSE, "tst"=FALSE}, {"D_offset"=0, "PDSR"=TRUE, "PCSR"=TRUE, "slp"=FALSE, "tst"=FALSE}, {"D_offset"=0, "PDSR"=TRUE, "PCSR"=TRUE, "slp"=FALSE, "tst"=FALSE}, {"D_offset"=0, "PDSR"=TRUE, "PCSR"=TRUE, "slp"=FALSE, "tst"=FALSE}, {"D_offset"=0, "PDSR"=TRUE, "PCSR"=TRUE, "slp"=FALSE, "tst"=FALSE}], [{"D_offset"=6, "PDSR"=FALSE, "PCSR"=TRUE, "slp"=FALSE, "tst"=FALSE}, {"D_offset"=6, "PDSR"=FALSE, "PCSR"=TRUE, "slp"=FALSE, "tst"=FALSE}, {"D_offset"=6, "PDSR"=FALSE, "PCSR"=TRUE, "slp"=FALSE, "tst"=FALSE}, {"D_offset"=6, "PDSR"=FALSE, "PCSR"=TRUE, "slp"=FALSE, "tst"=FALSE}, {"D_offset"=0, "PDSR"=TRUE, "PCSR"=TRUE, "slp"=FALSE, "tst"=FALSE}, {"D_offset"=0, "PDSR"=TRUE, "PCSR"=TRUE, "slp"=FALSE, "tst"=FALSE}, {"D_offset"=0, "PDSR"=TRUE, "PCSR"=TRUE, "slp"=FALSE, "tst"=FALSE}, {"D_offset"=0, "PDSR"=TRUE, "PCSR"=TRUE, "slp"=FALSE, "tst"=FALSE}], [{"D_offset"=6, "PDSR"=FALSE, "PCSR"=TRUE, "slp"=FALSE, "tst"=FALSE}, {"D_offset"=6, "PDSR"=FALSE, "PCSR"=TRUE, "slp"=FALSE, "tst"=FALSE}, {"D_offset"=6, "PDSR"=FALSE, "PCSR"=TRUE, "slp"=FALSE, "tst"=FALSE}, {"D_offset"=6, "PDSR"=FALSE, "PCSR"=TRUE, "slp"=FALSE, "tst"=FALSE}, {"D_offset"=0, "PDSR"=TRUE, "PCSR"=TRUE, "slp"=FALSE, "tst"=FALSE}, {"D_offset"=0, "PDSR"=TRUE, "PCSR"=TRUE, "slp"=FALSE, "tst"=FALSE}, {"D_offset"=0, "PDSR"=TRUE, "PCSR"=TRUE, "slp"=FALSE, "tst"=FALSE}, {"D_offset"=0, "PDSR"=TRUE, "PCSR"=TRUE, "slp"=FALSE, "tst"=FALSE}], [{"D_offset"=6, "PDSR"=FALSE, "PCSR"=TRUE, "slp"=FALSE, "tst"=FALSE}, {"D_offset"=6, "PDSR"=FALSE, "PCSR"=TRUE, "slp"=FALSE, "tst"=FALSE}, {"D_offset"=6, "PDSR"=FALSE, "PCSR"=TRUE, "slp"=FALSE, "tst"=FALSE}, {"D_offset"=6, "PDSR"=FALSE, "PCSR"=TRUE, "slp"=FALSE, "tst"=FALSE}, {"D_offset"=0, "PDSR"=TRUE, "PCSR"=TRUE, "slp"=FALSE, "tst"=FALSE}, {"D_offset"=0, "PDSR"=TRUE, "PCSR"=TRUE, "slp"=FALSE, "tst"=FALSE}, {"D_offset"=0, "PDSR"=TRUE, "PCSR"=TRUE, "slp"=FALSE, "tst"=FALSE}, {"D_offset"=0, "PDSR"=TRUE, "PCSR"=TRUE, "slp"=FALSE, "tst"=FALSE}], [{"D_offset"=6, "PDSR"=FALSE, "PCSR"=TRUE, "slp"=FALSE, "tst"=FALSE}, {"D_offset"=6, "PDSR"=FALSE, "PCSR"=TRUE, "slp"=FALSE, "tst"=FALSE}, {"D_offset"=6, "PDSR"=FALSE, "PCSR"=TRUE, "slp"=FALSE, "tst"=FALSE}, {"D_offset"=6, "PDSR"=FALSE, "PCSR"=TRUE, "slp"=FALSE, "tst"=FALSE}, {"D_offset"=0, "PDSR"=TRUE, "PCSR"=TRUE, "slp"=FALSE, "tst"=FALSE}, {"D_offset"=0, "PDSR"=TRUE, "PCSR"=TRUE, "slp"=FALSE, "tst"=FALSE}, {"D_offset"=0, "PDSR"=TRUE, "PCSR"=TRUE, "slp"=FALSE, "tst"=FALSE}, {"D_offset"=0, "PDSR"=TRUE, "PCSR"=TRUE, "slp"=FALSE, "tst"=FALSE}], [{"D_offset"=6, "PDSR"=FALSE, "PCSR"=TRUE, "slp"=FALSE, "tst"=FALSE}, {"D_offset"=6, "PDSR"=FALSE, "PCSR"=TRUE, "slp"=FALSE, "tst"=FALSE}, {"D_offset"=6, "PDSR"=FALSE, "PCSR"=TRUE, "slp"=FALSE, "tst"=FALSE}, {"D_offset"=6, "PDSR"=FALSE, "PCSR"=TRUE, "slp"=FALSE, "tst"=FALSE}, {"D_offset"=0, "PDSR"=TRUE, "PCSR"=TRUE, "slp"=FALSE, "tst"=FALSE}, {"D_offset"=0, "PDSR"=TRUE, "PCSR"=TRUE, "slp"=FALSE, "tst"=FALSE}, {"D_offset"=0, "PDSR"=TRUE, "PCSR"=TRUE, "slp"=FALSE, "tst"=FALSE}, {"D_offset"=0, "PDSR"=TRUE, "PCSR"=TRUE, "slp"=FALSE, "tst"=FALSE}], [{"D_offset"=6, "PDSR"=FALSE, "PCSR"=TRUE, "slp"=FALSE, "tst"=FALSE}, {"D_offset"=6, "PDSR"=FALSE, "PCSR"=TRUE, "slp"=FALSE, "tst"=FALSE}, {"D_offset"=6, "PDSR"=FALSE, "PCSR"=TRUE, "slp"=FALSE, "tst"=FALSE}, {"D_offset"=6, "PDSR"=FALSE, "PCSR"=TRUE, "slp"=FALSE, "tst"=FALSE}, {"D_offset"=0, "PDSR"=TRUE, "PCSR"=TRUE, "slp"=FALSE, "tst"=FALSE}, {"D_offset"=0, "PDSR"=TRUE, "PCSR"=TRUE, "slp"=FALSE, "tst"=FALSE}, {"D_offset"=0, "PDSR"=TRUE, "PCSR"=TRUE, "slp"=FALSE, "tst"=FALSE}, {"D_offset"=0, "PDSR"=TRUE, "PCSR"=TRUE, "slp"=FALSE, "tst"=FALSE}], [{"D_offset"=6, "PDSR"=FALSE, "PCSR"=TRUE, "slp"=FALSE, "tst"=FALSE}, {"D_offset"=6, "PDSR"=FALSE, "PCSR"=TRUE, "slp"=FALSE, "tst"=FALSE}, {"D_offset"=6, "PDSR"=FALSE, "PCSR"=TRUE, "slp"=FALSE, "tst"=FALSE}, {"D_offset"=6, "PDSR"=FALSE, "PCSR"=TRUE, "slp"=FALSE, "tst"=FALSE}, {"D_offset"=0, "PDSR"=TRUE, "PCSR"=TRUE, "slp"=FALSE, "tst"=FALSE}, {"D_offset"=0, "PDSR"=TRUE, "PCSR"=TRUE, "slp"=FALSE, "tst"=FALSE}, {"D_offset"=0, "PDSR"=TRUE, "PCSR"=TRUE, "slp"=FALSE, "tst"=FALSE}, {"D_offset"=0, "PDSR"=TRUE, "PCSR"=TRUE, "slp"=FALSE, "tst"=FALSE}], [{"D_offset"=6, "PDSR"=FALSE, "PCSR"=TRUE, "slp"=FALSE, "tst"=FALSE}, {"D_offset"=6, "PDSR"=FALSE, "PCSR"=TRUE, "slp"=FALSE, "tst"=FALSE}, {"D_offset"=6, "PDSR"=FALSE, "PCSR"=TRUE, "slp"=FALSE, "tst"=FALSE}, {"D_offset"=6, "PDSR"=FALSE, "PCSR"=TRUE, "slp"=FALSE, "tst"=FALSE}, {"D_offset"=0, "PDSR"=TRUE, "PCSR"=TRUE, "slp"=FALSE, "tst"=FALSE}, {"D_offset"=0, "PDSR"=TRUE, "PCSR"=TRUE, "slp"=FALSE, "tst"=FALSE}, {"D_offset"=0, "PDSR"=TRUE, "PCSR"=TRUE, "slp"=FALSE, "tst"=FALSE}, {"D_offset"=0, "PDSR"=TRUE, "PCSR"=TRUE, "slp"=FALSE, "tst"=FALSE}], [{"D_offset"=6, "PDSR"=FALSE, "PCSR"=TRUE, "slp"=FALSE, "tst"=FALSE}, {"D_offset"=6, "PDSR"=FALSE, "PCSR"=TRUE, "slp"=FALSE, "tst"=FALSE}, {"D_offset"=6, "PDSR"=FALSE, "PCSR"=TRUE, "slp"=FALSE, "tst"=FALSE}, {"D_offset"=6, "PDSR"=FALSE, "PCSR"=TRUE, "slp"=FALSE, "tst"=FALSE}, {"D_offset"=0, "PDSR"=TRUE, "PCSR"=TRUE, "slp"=FALSE, "tst"=FALSE}, {"D_offset"=0, "PDSR"=TRUE, "PCSR"=TRUE, "slp"=FALSE, "tst"=FALSE}, {"D_offset"=0, "PDSR"=TRUE, "PCSR"=TRUE, "slp"=FALSE, "tst"=FALSE}, {"D_offset"=0, "PDSR"=TRUE, "PCSR"=TRUE, "slp"=FALSE, "tst"=FALSE}], [{"D_offset"=6, "PDSR"=FALSE, "PCSR"=TRUE, "slp"=FALSE, "tst"=FALSE}, {"D_offset"=6, "PDSR"=FALSE, "PCSR"=TRUE, "slp"=FALSE, "tst"=FALSE}, {"D_offset"=6, "PDSR"=FALSE, "PCSR"=TRUE, "slp"=FALSE, "tst"=FALSE}, {"D_offset"=6, "PDSR"=FALSE, "PCSR"=TRUE, "slp"=FALSE, "tst"=FALSE}, {"D_offset"=0, "PDSR"=TRUE, "PCSR"=TRUE, "slp"=FALSE, "tst"=FALSE}, {"D_offset"=0, "PDSR"=TRUE, "PCSR"=TRUE, "slp"=FALSE, "tst"=FALSE}, {"D_offset"=0, "PDSR"=TRUE, "PCSR"=TRUE, "slp"=FALSE, "tst"=FALSE}, {"D_offset"=0, "PDSR"=TRUE, "PCSR"=TRUE, "slp"=FALSE, "tst"=FALSE}], [{"D_offset"=6, "PDSR"=FALSE, "PCSR"=TRUE, "slp"=FALSE, "tst"=FALSE}, {"D_offset"=6, "PDSR"=FALSE, "PCSR"=TRUE, "slp"=FALSE, "tst"=FALSE}, {"D_offset"=6, "PDSR"=FALSE, "PCSR"=TRUE, "slp"=FALSE, "tst"=FALSE}, {"D_offset"=6, "PDSR"=FALSE, "PCSR"=TRUE, "slp"=FALSE, "tst"=FALSE}, {"D_offset"=0, "PDSR"=TRUE, "PCSR"=TRUE, "slp"=FALSE, "tst"=FALSE}, {"D_offset"=0, "PDSR"=TRUE, "PCSR"=TRUE, "slp"=FALSE, "tst"=FALSE}, {"D_offset"=0, "PDSR"=TRUE, "PCSR"=TRUE, "slp"=FALSE, "tst"=FALSE}, {"D_offset"=0, "PDSR"=TRUE, "PCSR"=TRUE, "slp"=FALSE, "tst"=FALSE}], [{"D_offset"=6, "PDSR"=FALSE, "PCSR"=TRUE, "slp"=FALSE, "tst"=FALSE}, {"D_offset"=6, "PDSR"=FALSE, "PCSR"=TRUE, "slp"=FALSE, "tst"=FALSE}, {"D_offset"=6, "PDSR"=FALSE, "PCSR"=TRUE, "slp"=FALSE, "tst"=FALSE}, {"D_offset"=6, "PDSR"=FALSE, "PCSR"=TRUE, "slp"=FALSE, "tst"=FALSE}, {"D_offset"=0, "PDSR"=TRUE, "PCSR"=TRUE, "slp"=FALSE, "tst"=FALSE}, {"D_offset"=0, "PDSR"=TRUE, "PCSR"=TRUE, "slp"=FALSE, "tst"=FALSE}, {"D_offset"=0, "PDSR"=TRUE, "PCSR"=TRUE, "slp"=FALSE, "tst"=FALSE}, {"D_offset"=0, "PDSR"=TRUE, "PCSR"=TRUE, "slp"=FALSE, "tst"=FALSE}]] {"D_offset" items=["0", "1", "2", "3", "4", "5", "6", "7", "8", "9", "10", "11", "12", "13", "14", "15"]}
  out "ADC ARRAY":bool[](array[boolean])=[FALSE, FALSE, FALSE, TRUE, FALSE, TRUE, TRUE, FALSE, FALSE, FALSE, FALSE, TRUE, FALSE, TRUE, TRUE, FALSE, FALSE, FALSE, FALSE, TRUE, FALSE, TRUE, TRUE, FALSE, FALSE, FALSE, FALSE, TRUE, FALSE, TRUE, TRUE, FALSE, FALSE, FALSE, FALSE, TRUE, FALSE, TRUE, TRUE, FALSE, FALSE, FALSE, FALSE, TRUE, FALSE, TRUE, TRUE, FALSE, FALSE, FALSE, FALSE, TRUE, FALSE, TRUE, TRUE, FALSE, FALSE, FALSE, FALSE, TRUE, FALSE, TRUE, TRUE, FALSE, FALSE, FALSE, FALSE, TRUE, FALSE, TRUE, TRUE, FALSE, FALSE, FALSE, FALSE, TRUE, FALSE, TRUE, TRUE, FALSE, FALSE, FALSE, FALSE, TRUE, FALSE, TRUE, TRUE, FALSE, FALSE, FALSE, FALSE, TRUE, FALSE, TRUE, TRUE, FALSE, FALSE, FALSE, FALSE, TRUE, FALSE, TRUE, TRUE, FALSE, FALSE, FALSE, FALSE, TRUE, FALSE, TRUE, TRUE, FALSE, FALSE, FALSE, FALSE, TRUE, FALSE, TRUE, TRUE, FALSE, FALSE, FALSE, FALSE, TRUE, FALSE, TRUE, TRUE, FALSE, FALSE, FALSE, FALSE, FALSE, FALSE, FALSE, FALSE, FALSE, FALSE, FALSE, FALSE, FALSE, FALSE, TRUE, FALSE, TRUE, FALSE, FALSE, FALSE, TRUE, FALSE, TRUE, TRUE, FALSE, FALSE, FALSE, FALSE, TRUE, FALSE, TRUE, TRUE, FALSE, FALSE, FALSE, FALSE, TRUE, FALSE, TRUE, TRUE, FALSE, FALSE, FALSE, FALSE, TRUE, FALSE, TRUE, TRUE, FALSE, FALSE, FALSE, FALSE, TRUE, FALSE, TRUE, TRUE, FALSE, FALSE, FALSE, FALSE, TRUE, FALSE, TRUE, TRUE, FALSE, FALSE, FALSE, FALSE, TRUE, FALSE, TRUE, TRUE, FALSE, FALSE, FALSE, FALSE, TRUE, FALSE, TRUE, TRUE, FALSE, FALSE, FALSE, FALSE, TRUE, FALSE, TRUE, TRUE, FALSE, FALSE, FALSE, FALSE, TRUE, FALSE, TRUE, TRUE, FALSE, FALSE, FALSE, FALSE, TRUE, FALSE, TRUE, TRUE, FALSE, FALSE, FALSE, FALSE, TRUE, FALSE, TRUE, TRUE, FALSE, FALSE, FALSE, FALSE, TRUE, FALSE, TRUE, TRUE, FALSE, FALSE, FALSE, FALSE, TRUE, FALSE, TRUE, TRUE, FALSE, FALSE, FALSE, FALSE, TRUE, FALSE, TRUE, TRUE, FALSE, FALSE, FALSE, FALSE, TRUE, FALSE, TRUE, TRUE, FALSE, FALSE, FALSE, FALSE, FALSE, FALSE, FALSE, FALSE, FALSE, FALSE, FALSE, FALSE, FALSE, FALSE, TRUE, FALSE, TRUE, FALSE, FALSE, FALSE, TRUE, FALSE, TRUE, TRUE, FALSE, FALSE, FALSE, FALSE, TRUE, FALSE, TRUE, TRUE, FALSE, FALSE, FALSE, FALSE, TRUE, FALSE, TRUE, TRUE, FALSE, FALSE, FALSE, FALSE, TRUE, FALSE, TRUE, TRUE, FALSE, FALSE, FALSE, FALSE, TRUE, FALSE, TRUE, TRUE, FALSE, FALSE, FALSE, FALSE, TRUE, FALSE, TRUE, TRUE, FALSE, FALSE, FALSE, FALSE, TRUE, FALSE, TRUE, TRUE, FALSE, FALSE, FALSE, FALSE, TRUE, FALSE, TRUE, TRUE, FALSE, FALSE, FALSE, FALSE, TRUE, FALSE, TRUE, TRUE, FALSE, FALSE, FALSE, FALSE, TRUE, FALSE, TRUE, TRUE, FALSE, FALSE, FALSE, FALSE, TRUE, FALSE, TRUE, TRUE, FALSE, FALSE, FALSE, FALSE, TRUE, FALSE, TRUE, TRUE, FALSE, FALSE, FALSE, FALSE, TRUE, FALSE, TRUE, TRUE, FALSE, FALSE, FALSE, FALSE, TRUE, FALSE, TRUE, TRUE, FALSE, FALSE, FALSE, FALSE, TRUE, FALSE, TRUE, TRUE, FALSE, FALSE, FALSE, FALSE, TRUE, FALSE, TRUE, TRUE, FALSE, FALSE, FALSE, FALSE, FALSE, FALSE, FALSE, FALSE, FALSE, FALSE, FALSE, FALSE, FALSE, FALSE, TRUE, FALSE, TRUE, FALSE, FALSE, FALSE, TRUE, FALSE, TRUE, TRUE, FALSE, FALSE, FALSE, FALSE, TRUE, FALSE, TRUE, TRUE, FALSE, FALSE, FALSE, FALSE, TRUE, FALSE, TRUE, TRUE, FALSE, FALSE, FALSE, FALSE, TRUE, FALSE, TRUE, TRUE, FALSE, FALSE, FALSE, FALSE, TRUE, FALSE, TRUE, TRUE, FALSE, FALSE, FALSE, FALSE, TRUE, FALSE, TRUE, TRUE, FALSE, FALSE, FALSE, FALSE, TRUE, FALSE, TRUE, TRUE, FALSE, FALSE, FALSE, FALSE, TRUE, FALSE, TRUE, TRUE, FALSE, FALSE, FALSE, FALSE, TRUE, FALSE, TRUE, TRUE, FALSE, FALSE, FALSE, FALSE, TRUE, FALSE, TRUE, TRUE, FALSE, FALSE, FALSE, FALSE, TRUE, FALSE, TRUE, TRUE, FALSE, FALSE, FALSE, FALSE, TRUE, FALSE, TRUE, TRUE, FALSE, FALSE, FALSE, FALSE, TRUE, FALSE, TRUE, TRUE, FALSE, FALSE, FALSE, FALSE, TRUE, FALSE, TRUE, TRUE, FALSE, FALSE, FALSE, FALSE, TRUE, FALSE, TRUE, TRUE, FALSE, FALSE, FALSE, FALSE, TRUE, FALSE, TRUE, TRUE, FALSE, FALSE, FALSE, FALSE, FALSE, FALSE, FALSE, FALSE, FALSE, FALSE, FALSE, FALSE, FALSE, FALSE, TRUE, FALSE, TRUE]
  out "FE ARRAY":bool[](array[boolean])=[FALSE, FALSE, TRUE, TRUE, FALSE, FALSE, TRUE, TRUE, FALSE, FALSE, TRUE, TRUE, FALSE, FALSE, TRUE, TRUE, FALSE, FALSE, TRUE, TRUE, FALSE, FALSE, TRUE, TRUE, FALSE, FALSE, TRUE, TRUE, FALSE, FALSE, TRUE, TRUE, FALSE, FALSE, TRUE, TRUE, FALSE, FALSE, TRUE, TRUE, FALSE, FALSE, TRUE, TRUE, FALSE, FALSE, TRUE, TRUE, FALSE, FALSE, TRUE, TRUE, FALSE, FALSE, TRUE, TRUE, FALSE, FALSE, TRUE, TRUE, FALSE, FALSE, TRUE, TRUE, FALSE, FALSE, TRUE, TRUE, FALSE, FALSE, TRUE, TRUE, FALSE, FALSE, TRUE, TRUE, FALSE, FALSE, TRUE, TRUE, FALSE, FALSE, TRUE, TRUE, FALSE, FALSE, TRUE, TRUE, FALSE, FALSE, TRUE, TRUE, FALSE, FALSE, TRUE, TRUE, FALSE, FALSE, TRUE, TRUE, FALSE, FALSE, TRUE, TRUE, FALSE, FALSE, TRUE, TRUE, FALSE, FALSE, TRUE, TRUE, FALSE, FALSE, TRUE, TRUE, FALSE, FALSE, TRUE, TRUE, FALSE, FALSE, TRUE, TRUE, FALSE, FALSE, TRUE, TRUE, FALSE, FALSE, FALSE, FALSE, TRUE, FALSE, FALSE, FALSE, FALSE, TRUE, FALSE, TRUE, FALSE, FALSE, FALSE, TRUE]
  out "size(s)":i32=576
  in  "DAC  0x00-0x3f":u16=17 format="%x"
  in  "DAC":u16(ring)=2 items=["DISABLE TEST PULSE", "INTERNAL DAC", "EXTERNAL DAC", "DAC OUTPUT"]
  in  "STB":u16(ring) items=["Monitor Analog"=0, "Monitor Temp"=1, "Monitor Bandgap"=3]
  in  "Array 4":T6(array[cluster])=[{"EN_GR"=0, "CLKG"=1, "FRQC"=1, "F2"=0, "F1"=0, "F0"=0, "F3"=0, "F4 pipeline select"=0, "F5  TEST DATA"=0, "sLSB"=0}, {"EN_GR"=0, "CLKG"=0, "FRQC"=1, "F2"=0, "F1"=0, "F0"=0, "F3"=0, "F4 pipeline select"=0, "F5  TEST DATA"=0, "sLSB"=0}, {"EN_GR"=0, "CLKG"=0, "FRQC"=1, "F2"=0, "F1"=0, "F0"=0, "F3"=0, "F4 pipeline select"=0, "F5  TEST DATA"=0, "sLSB"=0}, {"EN_GR"=0, "CLKG"=0, "FRQC"=1, "F2"=0, "F1"=0, "F0"=0, "F3"=0, "F4 pipeline select"=0, "F5  TEST DATA"=1, "sLSB"=0}, {"EN_GR"=0, "CLKG"=2, "FRQC"=1, "F2"=0, "F1"=0, "F0"=0, "F3"=0, "F4 pipeline select"=0, "F5  TEST DATA"=0, "sLSB"=0}, {"EN_GR"=0, "CLKG"=2, "FRQC"=1, "F2"=0, "F1"=0, "F0"=0, "F3"=0, "F4 pipeline select"=0, "F5  TEST DATA"=0, "sLSB"=0}, {"EN_GR"=0, "CLKG"=2, "FRQC"=1, "F2"=0, "F1"=0, "F0"=0, "F3"=0, "F4 pipeline select"=0, "F5  TEST DATA"=0, "sLSB"=0}, {"EN_GR"=0, "CLKG"=2, "FRQC"=1, "F2"=0, "F1"=0, "F0"=0, "F3"=0, "F4 pipeline select"=0, "F5  TEST DATA"=0, "sLSB"=0}] {"sLSB" items=["FIFO write clock is the ADC write clock", "FIFO write clock is on pin IdxMp/n.  "]; "F5  TEST DATA" items=["ADC data is selected and pipelined.", "test data is selected and pipelined"]; "F4 pipeline select" items=["bit F5 controls the pipeline.", "CMOS pins CS and SCK controls the pipeline"]; "F3" items=["IDL falling edge is delayed of 5-10ns after IDXM rising edge.", "delay of 1 clock cycle on LVDS pin CLK"]; "F0" items=["the ADC write clock is generated internally.", "the ADC write clock is on LVDS pin IDXM"]; "F1" items=["a rising edge on LVDS pin ADC_CONV starts the sampling and readout.", "the readout is compatible to V* version"]; "F2" items=["FIFO clock generator on", "FIFO clock generator  off"]; "FRQC" items=["1 MHz", "2 MHz "]; "CLKG" items=["ADC clocks from internal FIFO controller,", "External clocks", "ADC clocks from internal monostable", "ADC clocks from internal FIFO controller,"]; "EN_GR" items=["Disables offset current absorption", "Enables the offset current absorption"]}
  in  "GLOBAL \nALL SAME":bool=TRUE
  in  "Array 3":T7(array[cluster])=[[{"sts"=TRUE, "snc"=TRUE, "SG"=0, "ST"=3, "SDC"=FALSE, "SDF"=FALSE}, {"sts"=TRUE, "snc"=TRUE, "SG"=1, "ST"=0, "SDC"=FALSE, "SDF"=FALSE}, {"sts"=TRUE, "snc"=TRUE, "SG"=1, "ST"=0, "SDC"=FALSE, "SDF"=FALSE}, {"sts"=TRUE, "snc"=TRUE, "SG"=1, "ST"=0, "SDC"=FALSE, "SDF"=FALSE}, {"sts"=TRUE, "snc"=TRUE, "SG"=1, "ST"=0, "SDC"=FALSE, "SDF"=FALSE}, {"sts"=TRUE, "snc"=TRUE, "SG"=1, "ST"=0, "SDC"=FALSE, "SDF"=FALSE}, {"sts"=TRUE, "snc"=TRUE, "SG"=1, "ST"=0, "SDC"=FALSE, "SDF"=FALSE}, {"sts"=TRUE, "snc"=TRUE, "SG"=1, "ST"=2, "SDC"=FALSE, "SDF"=FALSE}], [{"sts"=TRUE, "snc"=TRUE, "SG"=0, "ST"=3, "SDC"=FALSE, "SDF"=FALSE}, {"sts"=TRUE, "snc"=TRUE, "SG"=1, "ST"=0, "SDC"=FALSE, "SDF"=FALSE}, {"sts"=TRUE, "snc"=TRUE, "SG"=1, "ST"=0, "SDC"=FALSE, "SDF"=FALSE}, {"sts"=TRUE, "snc"=TRUE, "SG"=1, "ST"=0, "SDC"=FALSE, "SDF"=FALSE}, {"sts"=TRUE, "snc"=TRUE, "SG"=1, "ST"=0, "SDC"=FALSE, "SDF"=FALSE}, {"sts"=TRUE, "snc"=TRUE, "SG"=1, "ST"=0, "SDC"=FALSE, "SDF"=FALSE}, {"sts"=TRUE, "snc"=TRUE, "SG"=1, "ST"=0, "SDC"=FALSE, "SDF"=FALSE}, {"sts"=TRUE, "snc"=TRUE, "SG"=1, "ST"=2, "SDC"=FALSE, "SDF"=FALSE}], [{"sts"=TRUE, "snc"=TRUE, "SG"=0, "ST"=3, "SDC"=FALSE, "SDF"=FALSE}, {"sts"=TRUE, "snc"=TRUE, "SG"=1, "ST"=0, "SDC"=FALSE, "SDF"=FALSE}, {"sts"=TRUE, "snc"=TRUE, "SG"=1, "ST"=0, "SDC"=FALSE, "SDF"=FALSE}, {"sts"=TRUE, "snc"=TRUE, "SG"=1, "ST"=0, "SDC"=FALSE, "SDF"=FALSE}, {"sts"=TRUE, "snc"=TRUE, "SG"=1, "ST"=0, "SDC"=FALSE, "SDF"=FALSE}, {"sts"=TRUE, "snc"=TRUE, "SG"=1, "ST"=0, "SDC"=FALSE, "SDF"=FALSE}, {"sts"=TRUE, "snc"=TRUE, "SG"=1, "ST"=0, "SDC"=FALSE, "SDF"=FALSE}, {"sts"=TRUE, "snc"=TRUE, "SG"=1, "ST"=2, "SDC"=FALSE, "SDF"=FALSE}], [{"sts"=TRUE, "snc"=TRUE, "SG"=0, "ST"=3, "SDC"=FALSE, "SDF"=FALSE}, {"sts"=TRUE, "snc"=TRUE, "SG"=1, "ST"=0, "SDC"=FALSE, "SDF"=FALSE}, {"sts"=TRUE, "snc"=TRUE, "SG"=1, "ST"=0, "SDC"=FALSE, "SDF"=FALSE}, {"sts"=TRUE, "snc"=TRUE, "SG"=1, "ST"=0, "SDC"=FALSE, "SDF"=FALSE}, {"sts"=TRUE, "snc"=TRUE, "SG"=1, "ST"=0, "SDC"=FALSE, "SDF"=FALSE}, {"sts"=TRUE, "snc"=TRUE, "SG"=1, "ST"=0, "SDC"=FALSE, "SDF"=FALSE}, {"sts"=TRUE, "snc"=TRUE, "SG"=1, "ST"=0, "SDC"=FALSE, "SDF"=FALSE}, {"sts"=TRUE, "snc"=TRUE, "SG"=1, "ST"=2, "SDC"=FALSE, "SDF"=FALSE}], [{"sts"=TRUE, "snc"=TRUE, "SG"=0, "ST"=3, "SDC"=FALSE, "SDF"=FALSE}, {"sts"=TRUE, "snc"=TRUE, "SG"=1, "ST"=0, "SDC"=FALSE, "SDF"=FALSE}, {"sts"=TRUE, "snc"=TRUE, "SG"=1, "ST"=0, "SDC"=FALSE, "SDF"=FALSE}, {"sts"=TRUE, "snc"=TRUE, "SG"=1, "ST"=0, "SDC"=FALSE, "SDF"=FALSE}, {"sts"=TRUE, "snc"=TRUE, "SG"=1, "ST"=0, "SDC"=FALSE, "SDF"=FALSE}, {"sts"=TRUE, "snc"=TRUE, "SG"=1, "ST"=0, "SDC"=FALSE, "SDF"=FALSE}, {"sts"=TRUE, "snc"=TRUE, "SG"=1, "ST"=0, "SDC"=FALSE, "SDF"=FALSE}, {"sts"=TRUE, "snc"=TRUE, "SG"=1, "ST"=2, "SDC"=FALSE, "SDF"=FALSE}], [{"sts"=TRUE, "snc"=TRUE, "SG"=0, "ST"=3, "SDC"=FALSE, "SDF"=FALSE}, {"sts"=TRUE, "snc"=TRUE, "SG"=1, "ST"=0, "SDC"=FALSE, "SDF"=FALSE}, {"sts"=TRUE, "snc"=TRUE, "SG"=1, "ST"=0, "SDC"=FALSE, "SDF"=FALSE}, {"sts"=TRUE, "snc"=TRUE, "SG"=1, "ST"=0, "SDC"=FALSE, "SDF"=FALSE}, {"sts"=TRUE, "snc"=TRUE, "SG"=1, "ST"=0, "SDC"=FALSE, "SDF"=FALSE}, {"sts"=TRUE, "snc"=TRUE, "SG"=1, "ST"=0, "SDC"=FALSE, "SDF"=FALSE}, {"sts"=TRUE, "snc"=TRUE, "SG"=1, "ST"=0, "SDC"=FALSE, "SDF"=FALSE}, {"sts"=TRUE, "snc"=TRUE, "SG"=1, "ST"=2, "SDC"=FALSE, "SDF"=FALSE}], [{"sts"=TRUE, "snc"=TRUE, "SG"=0, "ST"=3, "SDC"=FALSE, "SDF"=FALSE}, {"sts"=TRUE, "snc"=TRUE, "SG"=1, "ST"=0, "SDC"=FALSE, "SDF"=FALSE}, {"sts"=TRUE, "snc"=TRUE, "SG"=1, "ST"=0, "SDC"=FALSE, "SDF"=FALSE}, {"sts"=TRUE, "snc"=TRUE, "SG"=1, "ST"=0, "SDC"=FALSE, "SDF"=FALSE}, {"sts"=TRUE, "snc"=TRUE, "SG"=1, "ST"=0, "SDC"=FALSE, "SDF"=FALSE}, {"sts"=TRUE, "snc"=TRUE, "SG"=1, "ST"=0, "SDC"=FALSE, "SDF"=FALSE}, {"sts"=TRUE, "snc"=TRUE, "SG"=1, "ST"=0, "SDC"=FALSE, "SDF"=FALSE}, {"sts"=TRUE, "snc"=TRUE, "SG"=1, "ST"=2, "SDC"=FALSE, "SDF"=FALSE}], [{"sts"=TRUE, "snc"=TRUE, "SG"=0, "ST"=3, "SDC"=FALSE, "SDF"=FALSE}, {"sts"=TRUE, "snc"=TRUE, "SG"=1, "ST"=0, "SDC"=FALSE, "SDF"=FALSE}, {"sts"=TRUE, "snc"=TRUE, "SG"=1, "ST"=0, "SDC"=FALSE, "SDF"=FALSE}, {"sts"=TRUE, "snc"=TRUE, "SG"=1, "ST"=0, "SDC"=FALSE, "SDF"=FALSE}, {"sts"=TRUE, "snc"=TRUE, "SG"=1, "ST"=0, "SDC"=FALSE, "SDF"=FALSE}, {"sts"=TRUE, "snc"=TRUE, "SG"=1, "ST"=0, "SDC"=FALSE, "SDF"=FALSE}, {"sts"=TRUE, "snc"=TRUE, "SG"=1, "ST"=0, "SDC"=FALSE, "SDF"=FALSE}, {"sts"=TRUE, "snc"=TRUE, "SG"=1, "ST"=2, "SDC"=FALSE, "SDF"=FALSE}], [{"sts"=TRUE, "snc"=TRUE, "SG"=0, "ST"=3, "SDC"=FALSE, "SDF"=FALSE}, {"sts"=TRUE, "snc"=TRUE, "SG"=1, "ST"=0, "SDC"=FALSE, "SDF"=FALSE}, {"sts"=TRUE, "snc"=TRUE, "SG"=1, "ST"=0, "SDC"=FALSE, "SDF"=FALSE}, {"sts"=TRUE, "snc"=TRUE, "SG"=1, "ST"=0, "SDC"=FALSE, "SDF"=FALSE}, {"sts"=TRUE, "snc"=TRUE, "SG"=1, "ST"=0, "SDC"=FALSE, "SDF"=FALSE}, {"sts"=TRUE, "snc"=TRUE, "SG"=1, "ST"=0, "SDC"=FALSE, "SDF"=FALSE}, {"sts"=TRUE, "snc"=TRUE, "SG"=1, "ST"=0, "SDC"=FALSE, "SDF"=FALSE}, {"sts"=TRUE, "snc"=TRUE, "SG"=1, "ST"=2, "SDC"=FALSE, "SDF"=FALSE}], [{"sts"=TRUE, "snc"=TRUE, "SG"=0, "ST"=3, "SDC"=FALSE, "SDF"=FALSE}, {"sts"=TRUE, "snc"=TRUE, "SG"=1, "ST"=0, "SDC"=FALSE, "SDF"=FALSE}, {"sts"=TRUE, "snc"=TRUE, "SG"=1, "ST"=0, "SDC"=FALSE, "SDF"=FALSE}, {"sts"=TRUE, "snc"=TRUE, "SG"=1, "ST"=0, "SDC"=FALSE, "SDF"=FALSE}, {"sts"=TRUE, "snc"=TRUE, "SG"=1, "ST"=0, "SDC"=FALSE, "SDF"=FALSE}, {"sts"=TRUE, "snc"=TRUE, "SG"=1, "ST"=0, "SDC"=FALSE, "SDF"=FALSE}, {"sts"=TRUE, "snc"=TRUE, "SG"=1, "ST"=0, "SDC"=FALSE, "SDF"=FALSE}, {"sts"=TRUE, "snc"=TRUE, "SG"=1, "ST"=2, "SDC"=FALSE, "SDF"=FALSE}], [{"sts"=TRUE, "snc"=TRUE, "SG"=0, "ST"=3, "SDC"=FALSE, "SDF"=FALSE}, {"sts"=TRUE, "snc"=TRUE, "SG"=1, "ST"=0, "SDC"=FALSE, "SDF"=FALSE}, {"sts"=TRUE, "snc"=TRUE, "SG"=1, "ST"=0, "SDC"=FALSE, "SDF"=FALSE}, {"sts"=TRUE, "snc"=TRUE, "SG"=1, "ST"=0, "SDC"=FALSE, "SDF"=FALSE}, {"sts"=TRUE, "snc"=TRUE, "SG"=1, "ST"=0, "SDC"=FALSE, "SDF"=FALSE}, {"sts"=TRUE, "snc"=TRUE, "SG"=1, "ST"=0, "SDC"=FALSE, "SDF"=FALSE}, {"sts"=TRUE, "snc"=TRUE, "SG"=1, "ST"=0, "SDC"=FALSE, "SDF"=FALSE}, {"sts"=TRUE, "snc"=TRUE, "SG"=1, "ST"=2, "SDC"=FALSE, "SDF"=FALSE}], [{"sts"=TRUE, "snc"=TRUE, "SG"=0, "ST"=3, "SDC"=FALSE, "SDF"=FALSE}, {"sts"=TRUE, "snc"=TRUE, "SG"=1, "ST"=0, "SDC"=FALSE, "SDF"=FALSE}, {"sts"=TRUE, "snc"=TRUE, "SG"=1, "ST"=0, "SDC"=FALSE, "SDF"=FALSE}, {"sts"=TRUE, "snc"=TRUE, "SG"=1, "ST"=0, "SDC"=FALSE, "SDF"=FALSE}, {"sts"=TRUE, "snc"=TRUE, "SG"=1, "ST"=0, "SDC"=FALSE, "SDF"=FALSE}, {"sts"=TRUE, "snc"=TRUE, "SG"=1, "ST"=0, "SDC"=FALSE, "SDF"=FALSE}, {"sts"=TRUE, "snc"=TRUE, "SG"=1, "ST"=0, "SDC"=FALSE, "SDF"=FALSE}, {"sts"=TRUE, "snc"=TRUE, "SG"=1, "ST"=2, "SDC"=FALSE, "SDF"=FALSE}], [{"sts"=TRUE, "snc"=TRUE, "SG"=0, "ST"=3, "SDC"=FALSE, "SDF"=FALSE}, {"sts"=TRUE, "snc"=TRUE, "SG"=1, "ST"=0, "SDC"=FALSE, "SDF"=FALSE}, {"sts"=TRUE, "snc"=TRUE, "SG"=1, "ST"=0, "SDC"=FALSE, "SDF"=FALSE}, {"sts"=TRUE, "snc"=TRUE, "SG"=1, "ST"=0, "SDC"=FALSE, "SDF"=FALSE}, {"sts"=TRUE, "snc"=TRUE, "SG"=1, "ST"=0, "SDC"=FALSE, "SDF"=FALSE}, {"sts"=TRUE, "snc"=TRUE, "SG"=1, "ST"=0, "SDC"=FALSE, "SDF"=FALSE}, {"sts"=TRUE, "snc"=TRUE, "SG"=1, "ST"=0, "SDC"=FALSE, "SDF"=FALSE}, {"sts"=TRUE, "snc"=TRUE, "SG"=1, "ST"=2, "SDC"=FALSE, "SDF"=FALSE}], [{"sts"=TRUE, "snc"=TRUE, "SG"=0, "ST"=3, "SDC"=FALSE, "SDF"=FALSE}, {"sts"=TRUE, "snc"=TRUE, "SG"=1, "ST"=0, "SDC"=FALSE, "SDF"=FALSE}, {"sts"=TRUE, "snc"=TRUE, "SG"=1, "ST"=0, "SDC"=FALSE, "SDF"=FALSE}, {"sts"=TRUE, "snc"=TRUE, "SG"=1, "ST"=0, "SDC"=FALSE, "SDF"=FALSE}, {"sts"=TRUE, "snc"=TRUE, "SG"=1, "ST"=0, "SDC"=FALSE, "SDF"=FALSE}, {"sts"=TRUE, "snc"=TRUE, "SG"=1, "ST"=0, "SDC"=FALSE, "SDF"=FALSE}, {"sts"=TRUE, "snc"=TRUE, "SG"=1, "ST"=0, "SDC"=FALSE, "SDF"=FALSE}, {"sts"=TRUE, "snc"=TRUE, "SG"=1, "ST"=2, "SDC"=FALSE, "SDF"=FALSE}], [{"sts"=TRUE, "snc"=TRUE, "SG"=0, "ST"=3, "SDC"=FALSE, "SDF"=FALSE}, {"sts"=TRUE, "snc"=TRUE, "SG"=1, "ST"=0, "SDC"=FALSE, "SDF"=FALSE}, {"sts"=TRUE, "snc"=TRUE, "SG"=1, "ST"=0, "SDC"=FALSE, "SDF"=FALSE}, {"sts"=TRUE, "snc"=TRUE, "SG"=1, "ST"=0, "SDC"=FALSE, "SDF"=FALSE}, {"sts"=TRUE, "snc"=TRUE, "SG"=1, "ST"=0, "SDC"=FALSE, "SDF"=FALSE}, {"sts"=TRUE, "snc"=TRUE, "SG"=1, "ST"=0, "SDC"=FALSE, "SDF"=FALSE}, {"sts"=TRUE, "snc"=TRUE, "SG"=1, "ST"=0, "SDC"=FALSE, "SDF"=FALSE}, {"sts"=TRUE, "snc"=TRUE, "SG"=1, "ST"=2, "SDC"=FALSE, "SDF"=FALSE}], [{"sts"=TRUE, "snc"=TRUE, "SG"=0, "ST"=3, "SDC"=FALSE, "SDF"=FALSE}, {"sts"=TRUE, "snc"=TRUE, "SG"=1, "ST"=0, "SDC"=FALSE, "SDF"=FALSE}, {"sts"=TRUE, "snc"=TRUE, "SG"=1, "ST"=0, "SDC"=FALSE, "SDF"=FALSE}, {"sts"=TRUE, "snc"=TRUE, "SG"=1, "ST"=0, "SDC"=FALSE, "SDF"=FALSE}, {"sts"=TRUE, "snc"=TRUE, "SG"=1, "ST"=0, "SDC"=FALSE, "SDF"=FALSE}, {"sts"=TRUE, "snc"=TRUE, "SG"=1, "ST"=0, "SDC"=FALSE, "SDF"=FALSE}, {"sts"=TRUE, "snc"=TRUE, "SG"=1, "ST"=0, "SDC"=FALSE, "SDF"=FALSE}, {"sts"=TRUE, "snc"=TRUE, "SG"=1, "ST"=2, "SDC"=FALSE, "SDF"=FALSE}]] {"ST" items=["0.5us"=1, "1us"=0, "2us"=3, "3us"=2]; "SG" items=["4.7 mV/fC", "7.8 mV/fC", "14 mV/fC", "25 mV/fC"]}
  in  "SLK":bool
  in  "SLK 2":bool=TRUE
  out "size(s) 2":i32=144
  out "ADC 1":bool=TRUE
  out "ADC 4":bool=TRUE
  out "ADC 3":bool=TRUE
  out "ADC 2":bool=TRUE
  in  "ALL SAME":bool=TRUE
  in  "OK Button 5":bool
  out "FE 1":bool=TRUE
  out "FE 4":bool=TRUE
  out "FE 3":bool=TRUE
  out "FE 2":bool=TRUE
  in  "PWR SCK 2":bool=TRUE
  in  "PWR SCK 3":bool=TRUE
  in  "PWR SCK 4":bool=TRUE
  out "SYNC":u8 format="%08b"
  in  "UDP READ":bool
  in  "UDP WRITE":bool
  out "DATA 3":u32=3835 format="%x"
  in  "ADDRESS 3":u16=63 format="%x"
  in  "DATA":u32=15 format="%x"
  in  "ADDRESS":u16=1 format="%x"
  in  "Remote Host":string="192.168.121.1"
  out "start_udp_IO":string="OK"
  out "UDP_CLEANUP":string="ok"
  in  "UDP/I2C":bool
  out "SBND_WIB_DLL_VERSION":u32=109
  out "FIMWARE VERSION":u32=259 format="%x"
  in  "THRD_SEL":i32
  in  "RING_BUF_SIZE":i32=500
  out "BUF_LEN":i32
  # "RAW \nBIN FILE"
  # "SYNC"
  # "200MHz"
  # "100MHz"
  # "1"
  # "1"
  # "1"
  # "1"
  # "1"
  # "1"
  # "2"
  # "2"
  # "2"
  # "2"
  # "2"
  # "2"
  # "3"
  # "3"
  # "3"
  # "3"
  # "3"
  # "3"
  # "4"
  # "4"
  # "4"
  # "4"
  # "4"
  # "4"
  # "UDP \nREADOUT MODE SELECT"
  # "SOCKET 2"
  # "SOCKET 1"
  # "SOCKET 3"
  # "SKT 1 VDDF"
  # "SKT 1 VDDD"
  # "SKT 2 VDDD"
  # "SKT 2 VDDA"
  # "SKT 1 VDDA"
  # "SKT 2 VDDF"
  # "SKT 3 VDDF"
  # "SKT 3 VDDD"
  # "SKT 4 VDDD"
  # "SKT 4 VDDA"
  # "SKT 3 VDDA"
  # "SKT 4 VDDF"
  # "SYNC STATUS"
  # "0"
  # "SPI STATUS"
  # "1"
  # "2"
  # "3"
  # "4"
  # "5"
  # "6"
  # "7"
  # "8"
  # "9"
  # "10"
  # "11"
  # "12"
  # "13"
  # "14"
  # "15"
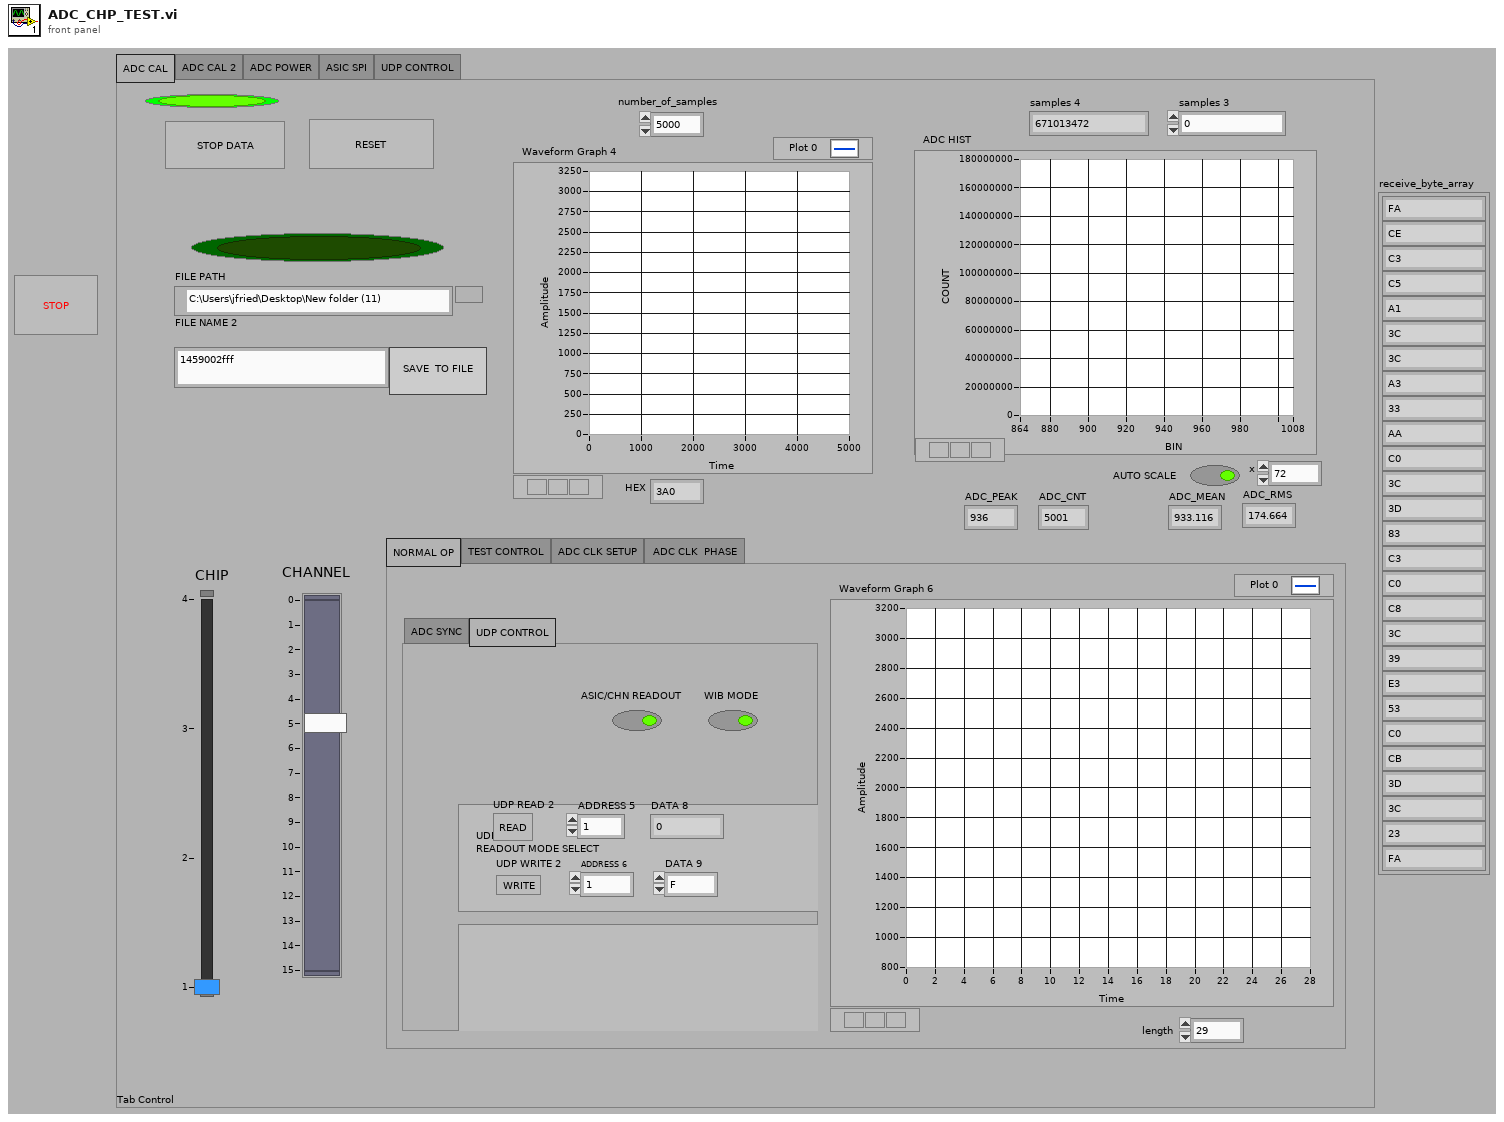
[diagram p1: front panel]
types:
  T1 = enum32{"ADC CAL", "ADC CAL 2", "ADC POWER", "ASIC SPI", "UDP CONTROL"}
  T2 = enum32{"NORMAL OP", "TEST CONTROL", "ADC CLK SETUP", "ADC CLK  PHASE "}
  T3 = cluster{"sts":bool, "snc":bool, "SG":u16, "ST":u16, "SDC":bool, "SDF":bool}
  T4 = cluster{"D_offset":u16, "PDSR":bool, "PCSR":bool, "slp":bool, "tst":bool}
  T5 = cluster{"D_offset":u16, "PDSR":bool, "PCSR":bool, "slp":bool, "tst":bool}[][]
  T6 = cluster{"EN_GR":u16, "CLKG":u16, "FRQC":u16, "F2":u16, "F1":u16, "F0":u16, "F3":u16, "F4 pipeline select":u16, "F5  TEST DATA":u16, "sLSB":u16}[]
  T7 = cluster{"sts":bool, "snc":bool, "SG":u16, "ST":u16, "SDC":bool, "SDF":bool}[][]
  T8 = cluster{"averaging mode":u16, "weighting mode":u16, "number of averages":u32}
  T9 = cluster{"dB On (F)":bool, "unwrap phase (F)":bool, "convert to degree (F)":bool}
  T10 = enum8{"Enabled", "Disabled", "Disabled and Grayed Out"}
  T11 = cluster{"D_offset":u16, "PDSR":bool, "PCSR":bool, "slp":bool, "tst":bool}[]
  T12 = cluster{"EN_GR":u16, "CLKG":u16, "FRQC":u16, "F2":u16, "F1":u16, "F0":u16, "F3":u16, "F4 pipeline select":u16, "F5  TEST DATA":u16, "sLSB":u16}
  T13 = cluster{"sts":bool, "snc":bool, "SG":u16, "ST":u16, "SDC":bool, "SDF":bool}[]
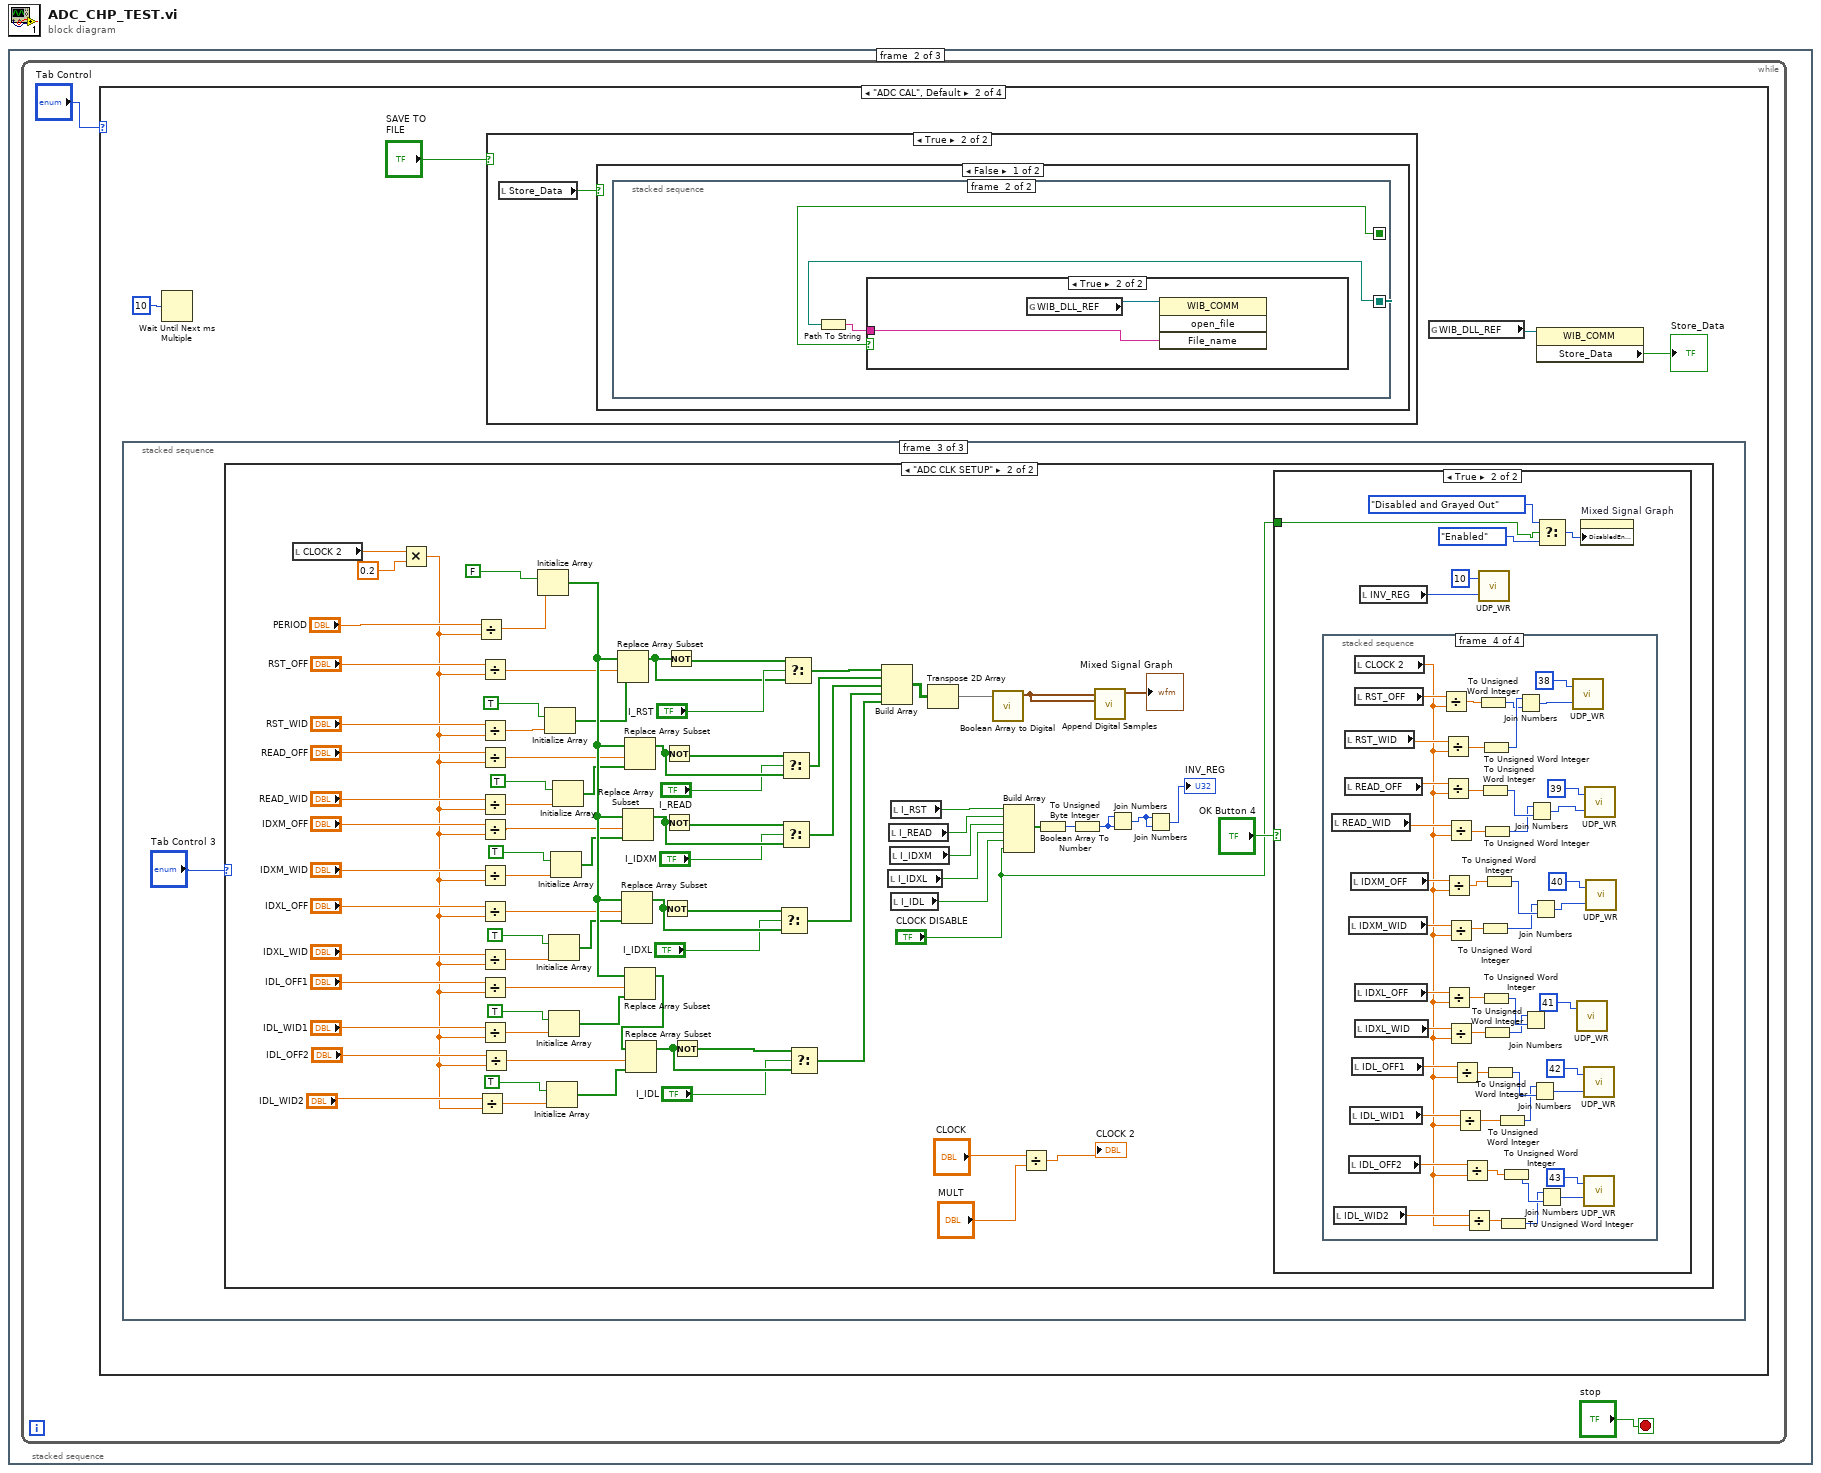
[diagram p0: block diagram]
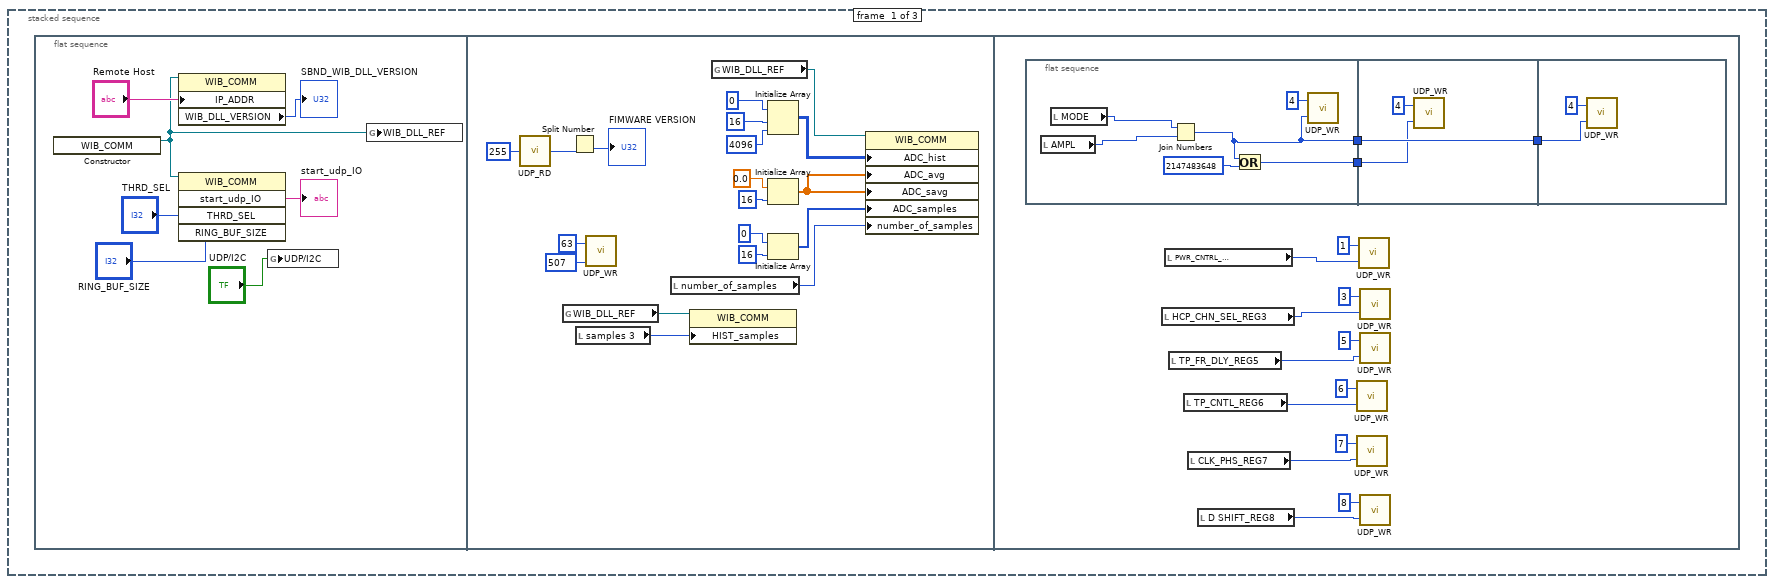
[diagram p2: hidden frame]
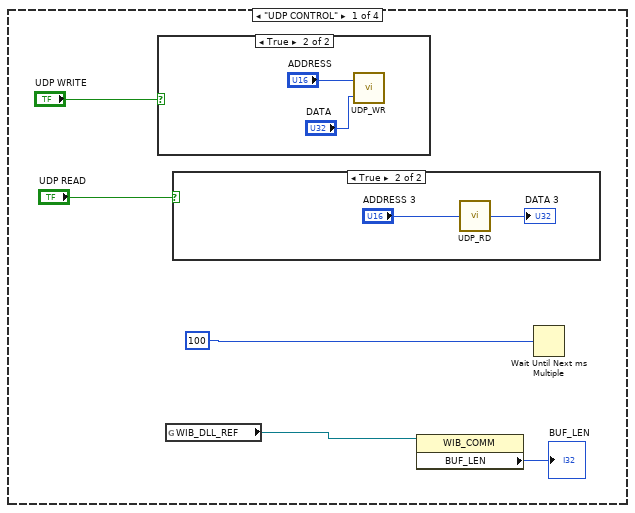
[diagram p3: hidden frame]
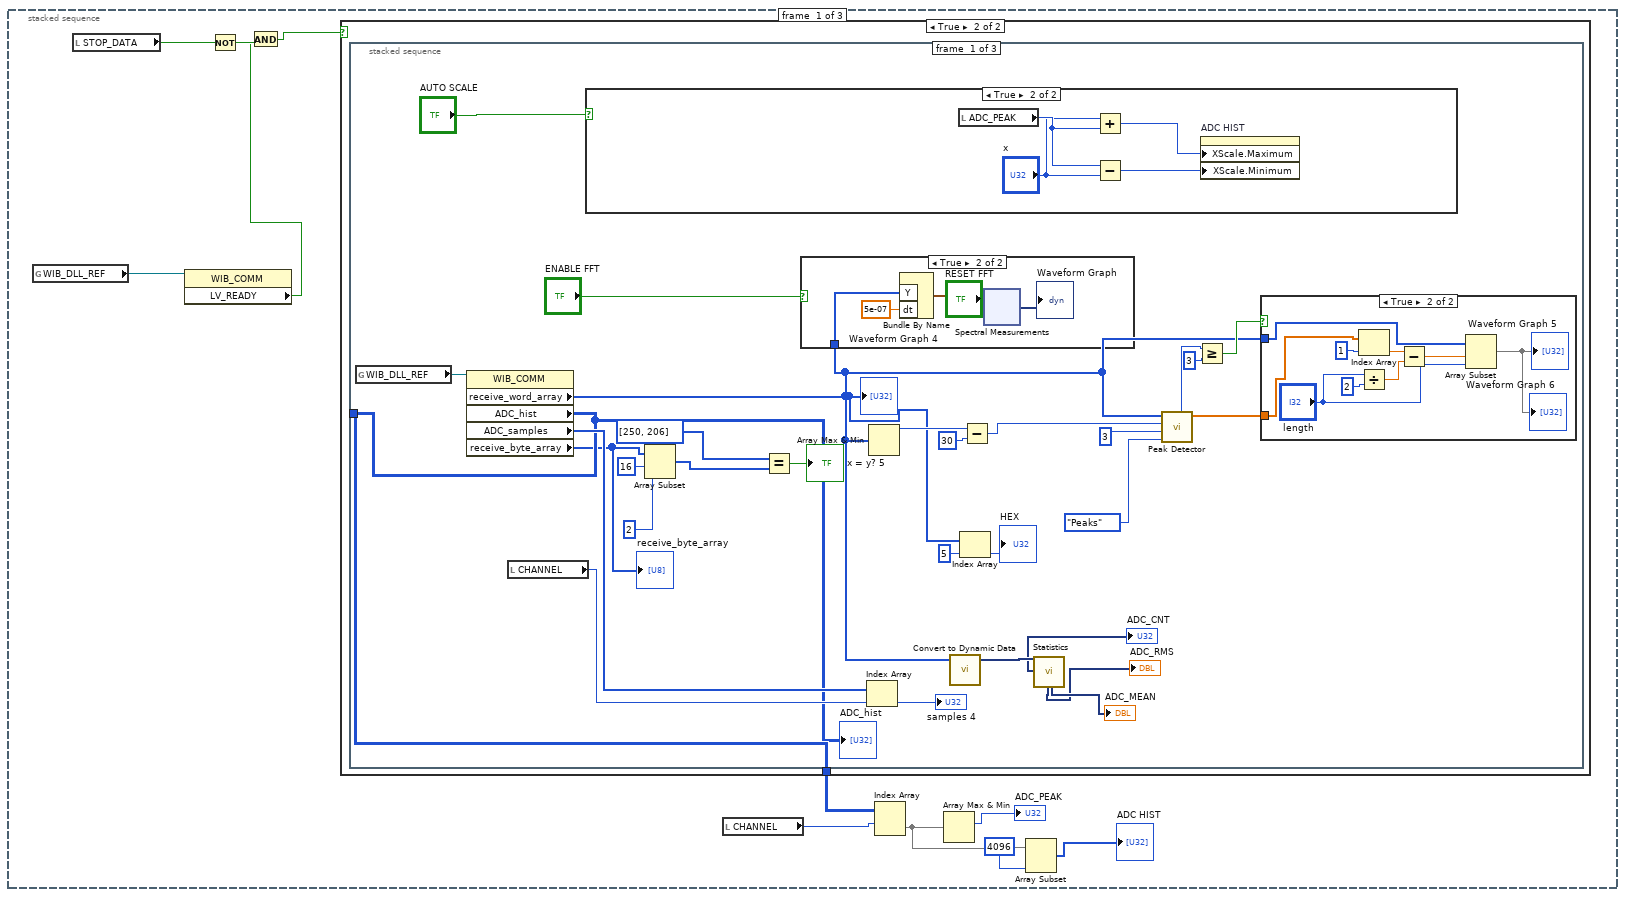
[diagram p6: hidden frame]
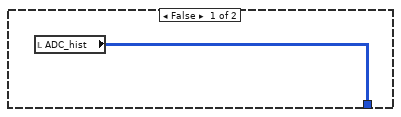
[diagram p7: hidden frame]
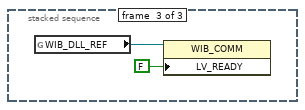
[diagram p12: hidden frame]
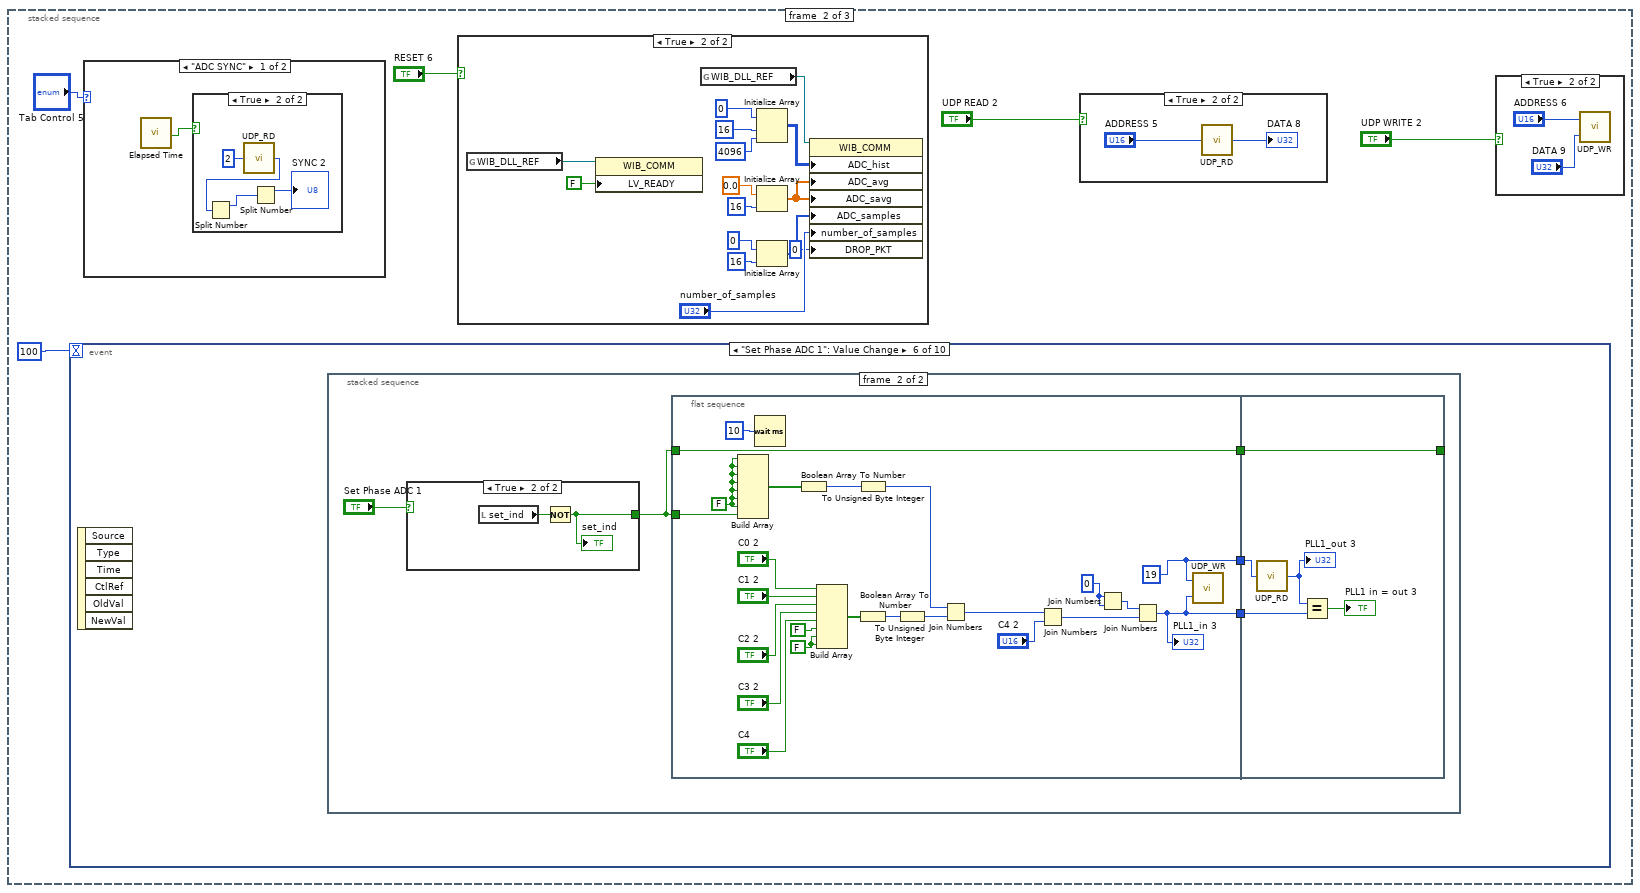
[diagram p13: hidden frame]
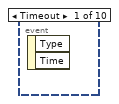
[diagram p16: hidden frame]
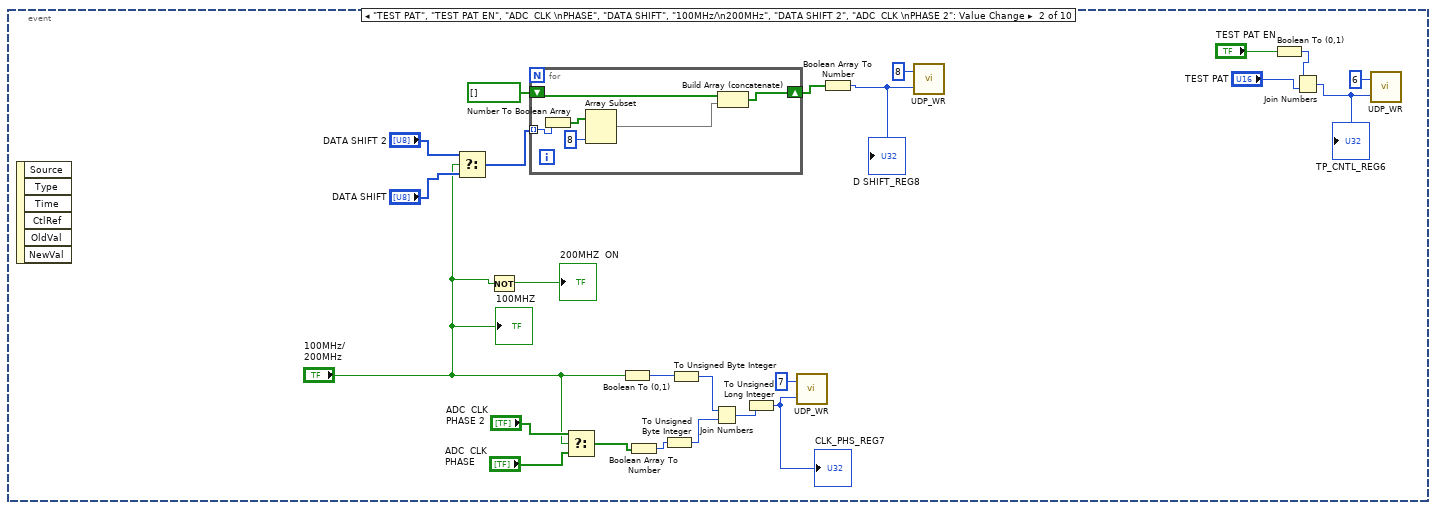
[diagram p17: hidden frame]
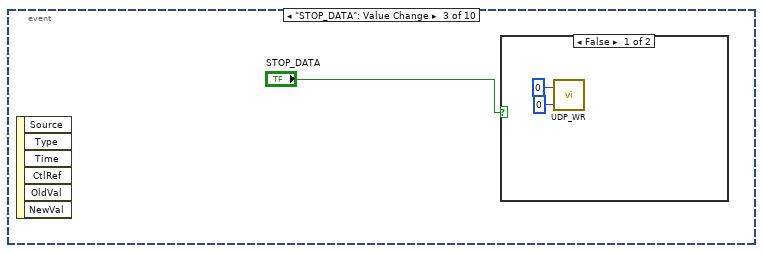
[diagram p18: hidden frame]
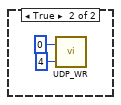
[diagram p19: hidden frame]
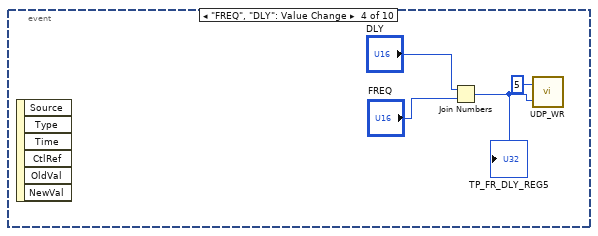
[diagram p20: hidden frame]
diagram:
  n1 = stacked-sequence {
    frame #0 {
      n2 = flat-sequence {
        frame #0 {
          n3 = constructor class="WIB_COMM"() -> (reference out=w3:refnum<k24>)  [unwired: 3 in, 2 out]
          n4 = property class="WIB_COMM"(reference=w3, "IP_ADDR"="Remote Host") -> ("WIB_DLL_VERSION"=→"SBND_WIB_DLL_VERSION":u32)  [unwired: 1 in, 2 out]
          n5 = invoke class="WIB_COMM" method="start_udp_IO"(reference=w3, "THRD_SEL"="THRD_SEL", "RING_BUF_SIZE"="RING_BUF_SIZE") -> ("start_udp_IO"=→"start_udp_IO":string)  [unwired: 2 in, 4 out]
          n6 = global write "WIB_Global.vi" "UDP/I2C"("UDP/I2C") -> ()
          n7 = global write "WIB_Global.vi" "WIB_DLL_REF"(w3) -> ()
        }
        frame #1 {
          n8 = call "UDP_RD.vi"("ADDRESS 2"=i16 255) -> ("DATA 2"=w10:u32)
          n9 = global read "WIB_Global.vi" "WIB_DLL_REF"() -> (w25:refnum<k24>)
          n10 = Split Number(x=w10) -> (lo(x)=→"FIMWARE VERSION":u16)  [unwired: 1 out]
          n11 = local read "samples 3"() -> (w26:i32)
          n12 = call "UDP_WR.vi"("DATA"=u32 507, "ADDRESS"=u16 63) -> ()  [unwired: 1 out]
          n13 = local read "number_of_samples"() -> (w24:u32)
          n14 = property class="WIB_COMM"(reference=w25, "HIST_samples"=w26) -> ()  [unwired: 1 in, 2 out]
          n15 = global read "WIB_Global.vi" "WIB_DLL_REF"() -> (w13:refnum<k24>)
          n16 = Initialize Array(u32 0 ("element"), 16 ("dimension size"), 4096 ("dimension size")) -> (w17:u32[][])
          n17 = Initialize Array(0.0 ("element"), 16 ("dimension size")) -> (w20:dbl[])
          n18 = Initialize Array(u32 0 ("element"), 16 ("dimension size")) -> (w22:u32[])
          n19 = property class="WIB_COMM"(reference=w13, "ADC_hist"=w17, "ADC_avg"=w20, "ADC_savg"=w20, "ADC_samples"=w22, "number_of_samples"=w24) -> ()  [unwired: 1 in, 2 out]
        }
        frame #2 {
          n20 = flat-sequence {
            tunnel: [w45] -> w41
            tunnel: [w44] -> w40
            tunnel: w41 -> [w48]
            tunnel: w40 -> [w50]
            tunnel: [w50] -> w39
            tunnel: w39 -> [w51]
            frame #0 {
              n21 = local read "AMPL"() -> (w42:u16)
              n22 = local read "MODE"() -> (w43:u16)
              n23 = Join Numbers(hi=w43, lo=w42) -> ((hi.lo)=w44:u32)
              n24 = Or(x=w44, y=u32 2147483648) -> (x .or. y?=w45:u32)
              n25 = call "UDP_WR.vi"("DATA"=w44, "ADDRESS"=u16 4) -> ()  [unwired: 1 out]
            }
            frame #1 {
              n26 = call "UDP_WR.vi"("DATA"=w48, "ADDRESS"=u16 4) -> ()  [unwired: 1 out]
            }
            frame #2 {
              n27 = call "UDP_WR.vi"("DATA"=w51, "ADDRESS"=u16 4) -> ()  [unwired: 1 out]
            }
          }
          n28 = local read "HCP_CHN_SEL_REG3"() -> (w38:u32)
          n29 = local read "PWR_CNTRL_\nREG 1"() -> (w27:u32)
          n30 = local read "TP_FR_DLY_REG5"() -> (w37:u32)
          n31 = local read "TP_CNTL_REG6"() -> (w36:u32)
          n32 = local read "CLK_PHS_REG7"() -> (w35:u32)
          n33 = local read "D SHIFT_REG8"() -> (w34:u32)
          n34 = call "UDP_WR.vi"("DATA"=w36, "ADDRESS"=u16 6) -> ()  [unwired: 1 out]
          n35 = call "UDP_WR.vi"("DATA"=w35, "ADDRESS"=u16 7) -> ()  [unwired: 1 out]
          n36 = call "UDP_WR.vi"("DATA"=w27, "ADDRESS"=u16 1) -> ()  [unwired: 1 out]
          n37 = call "UDP_WR.vi"("DATA"=w38, "ADDRESS"=u16 3) -> ()  [unwired: 1 out]
          n38 = call "UDP_WR.vi"("DATA"=w37, "ADDRESS"=u16 5) -> ()  [unwired: 1 out]
          n39 = call "UDP_WR.vi"("DATA"=w34, "ADDRESS"=u16 8) -> ()  [unwired: 1 out]
        }
      }
    }
    frame #1 {
      n40 = while {
        stop <- "stop" stop-if-true
        n41 = case shown="\"ADC CAL\", Default" "Tab Control" {
          frame "UDP CONTROL" {
            n42 = case shown="True" "UDP WRITE" {
              frame False {
              }
              frame True {
                n43 = call "UDP_WR.vi"("DATA"="DATA", "ADDRESS"="ADDRESS") -> ()  [unwired: 1 out]
              }
            }
            n44 = global read "WIB_Global.vi" "WIB_DLL_REF"() -> (w56:refnum<k24>)
            n45 = case shown="True" "UDP READ" {
              frame False {
              }
              frame True {
                n46 = call "UDP_RD.vi"("ADDRESS 2"="ADDRESS 3") -> ("DATA 2"=→"DATA 3":u32)
              }
            }
            n47 = property class="WIB_COMM"(reference=w56) -> ("BUF_LEN"=→"BUF_LEN":i32)  [unwired: 1 in, 2 out]
            n48 = Wait Until Next ms Multiple(millisecond multiple=u32 100) -> ()  [unwired: 1 out]
          }
          frame "ADC CAL", Default {
            n49 = stacked-sequence {
              frame #0 {
                n50 = global read "WIB_Global.vi" "WIB_DLL_REF"() -> (w71:refnum<k24>)
                n51 = local read "STOP_DATA"() -> (w78:bool)
                n52 = property class="WIB_COMM"(reference=w71) -> ("LV_READY"=w69:bool)  [unwired: 1 in, 2 out]
                n53 = Not(x=w78) -> (.not. x?=w70:bool)
                n54 = And(x=w70, y=w69) -> (x .and. y?=w68:bool)
                n55 = case shown="True" w68 {
                  tunnel: [w79 w80] -> w72
                  frame False {
                    n56 = local read "ADC_hist"() -> (w79:u32[][])
                  }
                  frame True {
                    n57 = stacked-sequence {
                      tunnel: [w92 _ _] -> w80
                      frame #0 {
                        n58 = global read "WIB_Global.vi" "WIB_DLL_REF"() -> (w105:refnum<k24>)
                        n59 = property class="WIB_COMM"(reference=w105) -> ("receive_word_array"=w83:u32[], "ADC_hist"=w92:u32[][], "ADC_samples"=w100:u32[], "receive_byte_array"=w89:u8[])  [unwired: 1 in, 2 out]
                        "Waveform Graph 4" <- w83
                        "ADC_hist" <- w92
                        "receive_byte_array" <- w89
                        n60 = local read "CHANNEL"() -> (w99:u8)
                        n61 = case shown="True" "AUTO SCALE" {
                          frame False {
                          }
                          frame True {
                            n62 = local read "ADC_PEAK"() -> (w138:u32)
                            n63 = Add(x="x", y=w138) -> (x+y=w137:u32)
                            n64 = Subtract(x=w138, y="x") -> (x-y=w136:u32)
                            n65 = property on="ADC HIST" class="WFGraph (strict)"("XScale.Maximum"=w137, "XScale.Minimum"=w136) -> ()  [unwired: 2 in, 2 out]
                          }
                        }
                        n66 = Array Subset(array=w89, index=16, length=2) -> (w85:u8[])
                        n67 = Equal?(x=u8[] [250, 206] ("subarray"), y=w85) -> (x = y?=→"x = y? 5":bool)
                        n68 = case shown="True" "ENABLE FFT" {
                          tunnel: w83 -> [_ w113]
                          frame False {
                          }
                          frame True {
                            n69 = Bundle By Name("Y"=w113, "dt"=5e-07) -> (w112:waveform(u32))  [unwired: 1 in]
                            n70 = xnode "Spectral Measurements"("Signals"=w112, "Restart Averaging"="RESET FFT") -> ("FFT - (Peak)"=→"Waveform Graph":dynamicdata)  [unwired: 1 in, 3 out]
                          }
                        }
                        n71 = Index Array(array=w100, index=w99) -> (element=→"samples 4":u32)
                        n72 = Array Max & Min(array=w83) -> (max value=w106:u32)  [unwired: 3 out]
                        n73 = call "Convert to Dynamic Data"("Array"=w83) -> ("Dynamic Data Type"=w103:dynamicdata)  [unwired: 3 in]
                        n74 = Index Array(array=w83, index=5) -> (element=→"HEX":u32)
                        n75 = Subtract(x=w106, y=30) -> (x-y=w107:u32)
                        n76 = call "Statistics"("Signals"=w103) -> ("Total Samples"=→"ADC_CNT":dynamicdata, "Standard Dev"=→"ADC_RMS":dynamicdata, "Arithmetic Mean"=→"ADC_MEAN":dynamicdata)  [unwired: 23 in, 1 out]
                        n77 = call <vilib>:"Peak Detector.vi"("peaks/valleys"=enum32{"Peaks", "Valleys"}."Peaks", "width"=3, "threshold"=w107, "X"=w83) -> ("Locations"=w97:dbl[], "# found"=w95:i32)  [unwired: 3 in, 3 out]
                        n78 = Greater Or Equal?(x=w95, y=3 ("x")) -> (x >= y?=w98:bool)
                        n79 = case shown="True" w98 {
                          tunnel: w97 -> [_ w134]
                          tunnel: w83 -> [_ w131]
                          frame False {
                          }
                          frame True {
                            n80 = Index Array(array=w134, index=1) -> (element=w132:dbl)
                            n81 = Divide(x="length", y=2) -> (x/y=w129:dbl)
                            n82 = Subtract(x=w132, y=w129) -> (x-y=w130:dbl)
                            n83 = Array Subset(array=w131, index=w130, length="length") -> (→"Waveform Graph 5" →"Waveform Graph 6":u32[])
                          }
                        }
                      }
                      frame #1 {
                      }
                      frame #2 {
                        n84 = global read "WIB_Global.vi" "WIB_DLL_REF"() -> (w139:refnum<k24>)
                        n85 = property class="WIB_COMM"(reference=w139, "LV_READY"=FALSE) -> ()  [unwired: 1 in, 2 out]
                      }
                    }
                  }
                }
                n86 = local read "CHANNEL"() -> (w76:u8)
                n87 = Index Array(array=w72, index (row)=w76) -> (element=w77:u32[])  [unwired: 1 in]
                n88 = Array Max & Min(array=w77) -> (max index (indices)=→"ADC_PEAK":i32)  [unwired: 3 out]
                n89 = Array Subset(array=w77, length=4096) -> (→"ADC HIST":u32[])  [unwired: 1 in]
              }
              frame #1 {
                n90 = event shown="[5] \"Set Phase ADC 1\": Value Change" {
                  selector: _ -> [_ _ _ _ _ _ _ _ _ _]
                  dyn-events: _ -> [_ _ _ _ _ _ _ _ _ _]
                  timeout: 100 -> [_ _ _ _ _ _ _ _ _ _]
                  event Timeout {
                    n91 = event-data() -> ()  [unwired: 1 in, 2 out]
                  }
                  event "TEST PAT", "TEST PAT EN", "ADC  CLK \nPHASE", "DATA SHIFT", "100MHz/\n200MHz", "DATA SHIFT 2", "ADC  CLK \nPHASE 2": Value Change {
                    n92 = event-data() -> ()  [unwired: 1 in, 6 out]
                    n93 = Select(t="DATA SHIFT 2", s="100MHz/\n200MHz", f="DATA SHIFT") -> (s? t:f=w153:u8[])
                    n94 = Not(x="100MHz/\n200MHz") -> (.not. x?=→"200MHZ  ON":bool)
                    n95 = for {
                      tunnel: w153 -> [w179] mode=indexing
                      shift-right: [w176] -> w165
                      shift-left: bool[] [] -> [w175]
                      n96 = Number To Boolean Array(number=w179) -> (Boolean array=w178:bool[])
                      n97 = Array Subset(array=w178, length=8) -> (w177:bool[])  [unwired: 1 in]
                      n98 = Build Array (concatenate)(w175, w177) -> (w176:bool[])
                    }
                    n99 = Select(t="ADC  CLK \nPHASE 2", s="100MHz/\n200MHz", f="ADC  CLK \nPHASE") -> (s? t:f=w156:bool[])
                    n100 = Boolean To (0,1)(Boolean="100MHz/\n200MHz") -> (0, 1=w163:i16)
                    n101 = Boolean Array To Number(Boolean array=w156) -> (number=w164:u32)
                    n102 = To Unsigned Byte Integer(number=w164) -> (unsigned 8bit integer=w161:u8)
                    n103 = To Unsigned Byte Integer(number=w163) -> (unsigned 8bit integer=w162:u8)
                    n104 = Join Numbers(hi=w162, lo=w161) -> ((hi.lo)=w160:u16)
                    n105 = To Unsigned Long Integer(number=w160) -> (unsigned 32bit integer=w159:u32)
                    "CLK_PHS_REG7" <- w159
                    n106 = call "UDP_WR.vi"("DATA"=w159, "ADDRESS"=u16 7) -> ()  [unwired: 1 out]
                    n107 = Boolean Array To Number(Boolean array=w165) -> (number=w167:u32)
                    "D SHIFT_REG8" <- w167
                    n108 = call "UDP_WR.vi"("DATA"=w167, "ADDRESS"=u16 8) -> ()  [unwired: 1 out]
                    n109 = Boolean To (0,1)(Boolean="TEST PAT EN") -> (0, 1=w172:i16)
                    n110 = Join Numbers(hi=w172, lo="TEST PAT") -> ((hi.lo)=w170:u32)
                    "TP_CNTL_REG6" <- w170
                    n111 = call "UDP_WR.vi"("DATA"=w170, "ADDRESS"=u16 6) -> ()  [unwired: 1 out]
                    "100MHZ" <- "100MHz/\n200MHz"
                  }
                  event "STOP_DATA": Value Change {
                    n112 = event-data() -> ()  [unwired: 1 in, 6 out]
                    n113 = case shown="False" "STOP_DATA" {
                      frame False {
                        n114 = call "UDP_WR.vi"("DATA"=u32 0, "ADDRESS"=u16 0) -> ()  [unwired: 1 out]
                      }
                      frame True {
                        n115 = call "UDP_WR.vi"("DATA"=u32 4, "ADDRESS"=u16 0) -> ()  [unwired: 1 out]
                      }
                    }
                  }
                  event "FREQ", "DLY": Value Change {
                    n116 = event-data() -> ()  [unwired: 1 in, 6 out]
                    n117 = Join Numbers(hi="DLY", lo="FREQ") -> ((hi.lo)=w187:u32)
                    "TP_FR_DLY_REG5" <- w187
                    n118 = call "UDP_WR.vi"("DATA"=w187, "ADDRESS"=u16 5) -> ()  [unwired: 1 out]
                  }
                  event "AMPL", "MODE": Value Change {
                    n119 = event-data() -> ()  [unwired: 1 in, 6 out]
                    n120 = flat-sequence {
                      tunnel: [w196] -> w192
                      tunnel: [w195] -> w191
                      tunnel: w192 -> [w199]
                      tunnel: w191 -> [w201]
                      tunnel: [w201] -> w190
                      tunnel: w190 -> [w202]
                      frame #0 {
                        n121 = Join Numbers(hi="MODE", lo="AMPL") -> ((hi.lo)=w195:u32)
                        n122 = Or(x=w195, y=u32 2147483648) -> (x .or. y?=w196:u32)
                        n123 = call "UDP_WR.vi"("DATA"=w195, "ADDRESS"=u16 4) -> ()  [unwired: 1 out]
                      }
                      frame #1 {
                        n124 = call "UDP_WR.vi"("DATA"=w199, "ADDRESS"=u16 4) -> ()  [unwired: 1 out]
                      }
                      frame #2 {
                        n125 = call "UDP_WR.vi"("DATA"=w202, "ADDRESS"=u16 4) -> ()  [unwired: 1 out]
                      }
                    }
                  }
                  event "Set Phase ADC 1": Value Change {
                    n126 = event-data() -> ()  [unwired: 1 in, 6 out]
                    n127 = stacked-sequence {
                      frame #0 {
                        n128 = flat-sequence {
                          tunnel: [w208] -> w207
                          tunnel: [w209] -> w206
                          tunnel: w206 -> [w216]
                          tunnel: w207 -> [w214]
                          tunnel: [w217] -> w205
                          tunnel: [w218] -> w204
                          tunnel: w205 -> [w223]
                          tunnel: w204 -> [w225]
                          frame #0 {
                            w208 = u16 17 ("ADDRESS 2")
                            n129 = Wait (ms)(milliseconds to wait=u32 10) -> ()  [unwired: 1 out]
                            n130 = Join Numbers(hi="C1", lo="C0") -> ((hi.lo)=w209:u32)
                            "PLL1_in" <- w209
                            n131 = call "UDP_WR.vi"("DATA"=w209, "ADDRESS"=w208) -> ()  [unwired: 1 out]
                          }
                          frame #1 {
                            n132 = call "UDP_RD.vi"("ADDRESS 2"=w214) -> ("DATA 2"=w213:u32)
                            "PLL1_out" <- w213
                            n133 = Equal?(x=w213, y=w216) -> (x = y?=→"PLL1 in = out":bool)
                          }
                          frame #2 {
                            w217 = u16 18 ("ADDRESS 2")
                            n134 = Wait (ms)(milliseconds to wait=u32 10) -> ()  [unwired: 1 out]
                            n135 = Join Numbers(hi="C3", lo="C2") -> ((hi.lo)=w218:u32)
                            "PLL1_in 2" <- w218
                            n136 = call "UDP_WR.vi"("DATA"=w218, "ADDRESS"=w217) -> ()  [unwired: 1 out]
                          }
                          frame #3 {
                            n137 = call "UDP_RD.vi"("ADDRESS 2"=w223) -> ("DATA 2"=w222:u32)
                            "PLL1_out 2" <- w222
                            n138 = Equal?(x=w222, y=w225) -> (x = y?=→"PLL1 in = out 2":bool)
                          }
                        }
                      }
                      frame #1 {
                        n139 = case shown="True" "Set Phase ADC 1" {
                          tunnel: [_ w260] -> w229
                          frame False {
                          }
                          frame True {
                            n140 = local read "set_ind"() -> (w261:bool)
                            n141 = Not(x=w261) -> (.not. x?=w260:bool)
                            "set_ind" <- w260
                          }
                        }
                        n142 = flat-sequence {
                          tunnel: w229 -> [w239]
                          tunnel: w229 -> [w233]
                          tunnel: [w233] -> w228
                          tunnel: [w232] -> w227
                          tunnel: [w231] -> w226
                          tunnel: w228 -> [w257]
                          tunnel: w227 -> [w256]
                          tunnel: w226 -> [w259]
                          tunnel: [w257] -> _
                          frame #0 {
                            w240 = FALSE ("element")
                            w243 = u8 0 ("hi")
                            w232 = u16 19 ("ADDRESS 2")
                            w241 = FALSE ("element")
                            n143 = Build Array(w240, w240, w240, w240, w240, w240, w240, w239) -> (w238:bool[])
                            n144 = Wait (ms)(milliseconds to wait=u32 10) -> ()  [unwired: 1 out]
                            n145 = Boolean Array To Number(Boolean array=w238) -> (number=w237:u32)
                            n146 = Build Array("C0 2", "C1 2", "C2 2", "C3 2", "C4", FALSE ("element"), w241, w241) -> (w249:bool[])
                            n147 = To Unsigned Byte Integer(number=w237) -> (unsigned 8bit integer=w236:u8)
                            n148 = Boolean Array To Number(Boolean array=w249) -> (number=w250:u32)
                            n149 = To Unsigned Byte Integer(number=w250) -> (unsigned 8bit integer=w235:u8)
                            n150 = Join Numbers(hi=w236, lo=w235) -> ((hi.lo)=w234:u16)
                            n151 = Join Numbers(hi=w234, lo="C4 2") -> ((hi.lo)=w253:u32)
                            n152 = Join Numbers(hi=w243, lo=w243) -> ((hi.lo)=w254:u16)
                            n153 = Join Numbers(hi=w254, lo=w253) -> ((hi.lo)=w231:u64)
                            "PLL1_in 3" <- w231
                            n154 = call "UDP_WR.vi"("DATA"=w231, "ADDRESS"=w232) -> ()  [unwired: 1 out]
                          }
                          frame #1 {
                            n155 = call "UDP_RD.vi"("ADDRESS 2"=w256) -> ("DATA 2"=w255:u32)
                            "PLL1_out 3" <- w255
                            n156 = Equal?(x=w255, y=w259) -> (x = y?=→"PLL1 in = out 3":bool)
                          }
                        }
                      }
                    }
                  }
                  event "Set Phase ADC 2": Value Change {
                    n157 = event-data() -> ()  [unwired: 1 in, 6 out]
                    n158 = stacked-sequence {
                      frame #0 {
                        n159 = flat-sequence {
                          tunnel: [w266] -> w265
                          tunnel: [w267] -> w264
                          tunnel: w264 -> [w274]
                          tunnel: w265 -> [w272]
                          tunnel: [w276] -> w263
                          tunnel: [w275] -> w262
                          tunnel: w263 -> [w280]
                          tunnel: w262 -> [w283]
                          frame #0 {
                            w266 = u16 26 ("ADDRESS 2")
                            n160 = Wait (ms)(milliseconds to wait=u32 10) -> ()  [unwired: 1 out]
                            n161 = Join Numbers(hi="C1 3", lo="C0 3") -> ((hi.lo)=w267:u32)
                            "PLL1_in 4" <- w267
                            n162 = call "UDP_WR.vi"("DATA"=w267, "ADDRESS"=w266) -> ()  [unwired: 1 out]
                          }
                          frame #1 {
                            n163 = call "UDP_RD.vi"("ADDRESS 2"=w272) -> ("DATA 2"=w271:u32)
                            "PLL1_out 4" <- w271
                            n164 = Equal?(x=w271, y=w274) -> (x = y?=→"PLL1 in = out 4":bool)
                          }
                          frame #2 {
                            w276 = u16 27 ("ADDRESS 2")
                            n165 = Wait (ms)(milliseconds to wait=u32 10) -> ()  [unwired: 1 out]
                            n166 = Join Numbers(hi="C3 3", lo="C2 3") -> ((hi.lo)=w275:u32)
                            "PLL1_in 5" <- w275
                            n167 = call "UDP_WR.vi"("DATA"=w275, "ADDRESS"=w276) -> ()  [unwired: 1 out]
                          }
                          frame #3 {
                            n168 = call "UDP_RD.vi"("ADDRESS 2"=w280) -> ("DATA 2"=w281:u32)
                            "PLL1_out 5" <- w281
                            n169 = Equal?(x=w281, y=w283) -> (x = y?=→"PLL1 in = out 5":bool)
                          }
                        }
                      }
                      frame #1 {
                        n170 = case shown="True" "Set Phase ADC 2" {
                          tunnel: [_ w318] -> w287
                          frame False {
                          }
                          frame True {
                            n171 = local read "set_ind 2"() -> (w319:bool)
                            n172 = Not(x=w319) -> (.not. x?=w318:bool)
                            "set_ind 2" <- w318
                          }
                        }
                        n173 = flat-sequence {
                          tunnel: w287 -> [w297]
                          tunnel: w287 -> [w291]
                          tunnel: [w291] -> w286
                          tunnel: [w290] -> w285
                          tunnel: [w289] -> w284
                          tunnel: w286 -> [w315]
                          tunnel: w285 -> [w313]
                          tunnel: w284 -> [w317]
                          tunnel: [w315] -> _
                          frame #0 {
                            w298 = FALSE ("element")
                            w301 = u8 0 ("hi")
                            w290 = u16 28 ("ADDRESS 2")
                            w299 = FALSE ("element")
                            n174 = Build Array(w298, w298, w298, w298, w298, w298, w298, w297) -> (w296:bool[])
                            n175 = Wait (ms)(milliseconds to wait=u32 10) -> ()  [unwired: 1 out]
                            n176 = Boolean Array To Number(Boolean array=w296) -> (number=w295:u32)
                            n177 = Build Array("C0 4", "C1 4", "C2 4", "C3 4", "C4 3", FALSE ("element"), w299, w299) -> (w307:bool[])
                            n178 = To Unsigned Byte Integer(number=w295) -> (unsigned 8bit integer=w294:u8)
                            n179 = Boolean Array To Number(Boolean array=w307) -> (number=w308:u32)
                            n180 = To Unsigned Byte Integer(number=w308) -> (unsigned 8bit integer=w293:u8)
                            n181 = Join Numbers(hi=w294, lo=w293) -> ((hi.lo)=w292:u16)
                            n182 = Join Numbers(hi=w292, lo="C4 4") -> ((hi.lo)=w311:u32)
                            n183 = Join Numbers(hi=w301, lo=w301) -> ((hi.lo)=w312:u16)
                            n184 = Join Numbers(hi=w312, lo=w311) -> ((hi.lo)=w289:u64)
                            "PLL1_in 6" <- w289
                            n185 = call "UDP_WR.vi"("DATA"=w289, "ADDRESS"=w290) -> ()  [unwired: 1 out]
                          }
                          frame #1 {
                            n186 = call "UDP_RD.vi"("ADDRESS 2"=w313) -> ("DATA 2"=w314:u32)
                            "PLL1_out 6" <- w314
                            n187 = Equal?(x=w314, y=w317) -> (x = y?=→"PLL1 in = out 6":bool)
                          }
                        }
                      }
                    }
                  }
                  event "Set Phase ADC 3": Value Change {
                    n188 = event-data() -> ()  [unwired: 1 in, 6 out]
                    n189 = stacked-sequence {
                      frame #0 {
                        n190 = flat-sequence {
                          tunnel: [w324] -> w323
                          tunnel: [w325] -> w322
                          tunnel: w322 -> [w332]
                          tunnel: w323 -> [w329]
                          tunnel: [w333] -> w321
                          tunnel: [w334] -> w320
                          tunnel: w321 -> [w338]
                          tunnel: w320 -> [w341]
                          frame #0 {
                            w324 = u16 44 ("ADDRESS 2")
                            n191 = Wait (ms)(milliseconds to wait=u32 10) -> ()  [unwired: 1 out]
                            n192 = Join Numbers(hi="C1 5", lo="C0 5") -> ((hi.lo)=w325:u32)
                            "PLL1_in 7" <- w325
                            n193 = call "UDP_WR.vi"("DATA"=w325, "ADDRESS"=w324) -> ()  [unwired: 1 out]
                          }
                          frame #1 {
                            n194 = call "UDP_RD.vi"("ADDRESS 2"=w329) -> ("DATA 2"=w330:u32)
                            "PLL1_out 7" <- w330
                            n195 = Equal?(x=w330, y=w332) -> (x = y?=→"PLL1 in = out 7":bool)
                          }
                          frame #2 {
                            w333 = u16 45 ("ADDRESS 2")
                            n196 = Wait (ms)(milliseconds to wait=u32 10) -> ()  [unwired: 1 out]
                            n197 = Join Numbers(hi="C3 5", lo="C2 5") -> ((hi.lo)=w334:u32)
                            "PLL1_in 8" <- w334
                            n198 = call "UDP_WR.vi"("DATA"=w334, "ADDRESS"=w333) -> ()  [unwired: 1 out]
                          }
                          frame #3 {
                            n199 = call "UDP_RD.vi"("ADDRESS 2"=w338) -> ("DATA 2"=w339:u32)
                            "PLL1_out 8" <- w339
                            n200 = Equal?(x=w339, y=w341) -> (x = y?=→"PLL1 in = out 8":bool)
                          }
                        }
                      }
                      frame #1 {
                        n201 = case shown="True" "Set Phase ADC 3" {
                          tunnel: [_ w376] -> w345
                          frame False {
                          }
                          frame True {
                            n202 = local read "set_ind 3"() -> (w377:bool)
                            n203 = Not(x=w377) -> (.not. x?=w376:bool)
                            "set_ind 3" <- w376
                          }
                        }
                        n204 = flat-sequence {
                          tunnel: w345 -> [w355]
                          tunnel: w345 -> [w349]
                          tunnel: [w349] -> w344
                          tunnel: [w347] -> w343
                          tunnel: [w348] -> w342
                          tunnel: w344 -> [w373]
                          tunnel: w343 -> [w371]
                          tunnel: w342 -> [w375]
                          tunnel: [w373] -> _
                          frame #0 {
                            w356 = FALSE ("element")
                            w359 = u8 0 ("hi")
                            w347 = u16 46 ("ADDRESS 2")
                            w357 = FALSE ("element")
                            n205 = Build Array(w356, w356, w356, w356, w356, w356, w356, w355) -> (w354:bool[])
                            n206 = Wait (ms)(milliseconds to wait=u32 10) -> ()  [unwired: 1 out]
                            n207 = Boolean Array To Number(Boolean array=w354) -> (number=w353:u32)
                            n208 = Build Array("C0 6", "C1 6", "C2 6", "C3 6", "C4 5", FALSE ("element"), w357, w357) -> (w365:bool[])
                            n209 = To Unsigned Byte Integer(number=w353) -> (unsigned 8bit integer=w352:u8)
                            n210 = Boolean Array To Number(Boolean array=w365) -> (number=w366:u32)
                            n211 = To Unsigned Byte Integer(number=w366) -> (unsigned 8bit integer=w351:u8)
                            n212 = Join Numbers(hi=w352, lo=w351) -> ((hi.lo)=w350:u16)
                            n213 = Join Numbers(hi=w350, lo="C4 6") -> ((hi.lo)=w369:u32)
                            n214 = Join Numbers(hi=w359, lo=w359) -> ((hi.lo)=w370:u16)
                            n215 = Join Numbers(hi=w370, lo=w369) -> ((hi.lo)=w348:u64)
                            "PLL1_in 9" <- w348
                            n216 = call "UDP_WR.vi"("DATA"=w348, "ADDRESS"=w347) -> ()  [unwired: 1 out]
                          }
                          frame #1 {
                            n217 = call "UDP_RD.vi"("ADDRESS 2"=w371) -> ("DATA 2"=w372:u32)
                            "PLL1_out 9" <- w372
                            n218 = Equal?(x=w372, y=w375) -> (x = y?=→"PLL1 in = out 9":bool)
                          }
                        }
                      }
                    }
                  }
                  event "samples 3": Value Change {
                    n219 = event-data() -> ()  [unwired: 1 in, 6 out]
                    n220 = global read "WIB_Global.vi" "WIB_DLL_REF"() -> (w379:refnum<k24>)
                    n221 = property class="WIB_COMM"(reference=w379, "HIST_samples"="samples 3") -> ()  [unwired: 1 in, 2 out]
                  }
                  event "CHANNEL", "CHIP", "ASIC/CHN READOUT": Value Change {
                    n222 = event-data() -> ()  [unwired: 1 in, 6 out]
                    n223 = flat-sequence {
                      frame #0 {
                        n224 = call "UDP_WR.vi"("DATA"=u32 1, "ADDRESS"=u16 9) -> ()  [unwired: 1 out]
                      }
                      frame #1 {
                        n225 = Wait Until Next ms Multiple(millisecond multiple=u32 1) -> ()  [unwired: 1 out]
                      }
                      frame #2 {
                        n226 = global read "WIB_Global.vi" "WIB_DLL_REF"() -> (w397:refnum<k24>)
                        n227 = Select(t=u32 0 ("address"), s="ASIC/CHN READOUT", f=u32 4096 ("address")) -> (s? t:f=w383:u32)
                        n228 = Select(t=u32 2147483648 ("address"), s="WIB MODE", f=u32 0 ("address")) -> (s? t:f=w387:u32)
                        n229 = property class="WIB_COMM"(reference=w397, "CHN_SEL"="CHANNEL") -> ()  [unwired: 1 in, 2 out]
                        n230 = Join Numbers(hi="CHANNEL", lo="CHIP") -> ((hi.lo)=w391:u16)
                        n231 = To Unsigned Long Integer(number=w391) -> (unsigned 32bit integer=w388:u32)
                        n232 = Compound Arithmetic op=OR(w388, w387, w383) -> (w389:u32)
                        "HCP_CHN_SEL_REG3" <- w389
                        n233 = call "UDP_WR.vi"("DATA"=w389, "ADDRESS"=u16 3 ("address")) -> ()  [unwired: 1 out]
                      }
                      frame #3 {
                        n234 = Wait Until Next ms Multiple(millisecond multiple=u32 1) -> ()  [unwired: 1 out]
                      }
                      frame #4 {
                        n235 = call "UDP_WR.vi"("DATA"=u32 0, "ADDRESS"=u16 9) -> ()  [unwired: 1 out]
                      }
                    }
                  }
                }
                n236 = case shown="\"ADC SYNC\"" "Tab Control 5" {
                  frame "ADC SYNC" {
                    n237 = call "Elapsed Time"() -> ("Time has Elapsed"=w146:bool)  [unwired: 12 in, 7 out]
                    n238 = case shown="True" w146 {
                      frame False {
                      }
                      frame True {
                        n239 = call "UDP_RD.vi"("ADDRESS 2"=i16 2) -> ("DATA 2"=w147:u32)
                        n240 = Split Number(x=w147) -> (hi(x)=w149:u16)  [unwired: 1 out]
                        n241 = Split Number(x=w149) -> (hi(x)=→"SYNC 2":u8)  [unwired: 1 out]
                      }
                    }
                  }
                  frame "UDP CONTROL", Default {
                  }
                }
                n242 = case shown="True" "RESET 6" {
                  frame False {
                  }
                  frame True {
                    n243 = global read "WIB_Global.vi" "WIB_DLL_REF"() -> (w406:refnum<k24>)
                    n244 = property class="WIB_COMM"(reference=w406, "LV_READY"=FALSE) -> ()  [unwired: 1 in, 2 out]
                    n245 = global read "WIB_Global.vi" "WIB_DLL_REF"() -> (w409:refnum<k24>)
                    n246 = Initialize Array(u32 0 ("element"), 16 ("dimension size"), 4096 ("dimension size")) -> (w413:u32[][])
                    n247 = Initialize Array(0.0 ("element"), 16 ("dimension size")) -> (w416:dbl[])
                    n248 = Initialize Array(u32 0 ("element"), 16 ("dimension size")) -> (w418:u32[])
                    n249 = property class="WIB_COMM"(reference=w409, "ADC_hist"=w413, "ADC_avg"=w416, "ADC_savg"=w416, "ADC_samples"=w418, "number_of_samples"="number_of_samples", "DROP_PKT"=0) -> ()  [unwired: 1 in, 2 out]
                  }
                }
                n250 = case shown="True" "UDP READ 2" {
                  frame False {
                  }
                  frame True {
                    n251 = call "UDP_RD.vi"("ADDRESS 2"="ADDRESS 5") -> ("DATA 2"=→"DATA 8":u32)
                  }
                }
                n252 = case shown="True" "UDP WRITE 2" {
                  frame False {
                  }
                  frame True {
                    n253 = call "UDP_WR.vi"("DATA"="DATA 9", "ADDRESS"="ADDRESS 6") -> ()  [unwired: 1 out]
                  }
                }
              }
              frame #2 {
                n254 = case shown="\"ADC CLK SETUP\"" "Tab Control 3" {
                  frame "NORMAL OP", Default {
                  }
                  frame "ADC CLK SETUP" {
                    n255 = local read "CLOCK 2"() -> (w429:dbl)
                    n256 = Multiply(x=w429, y=0.2) -> (x*y=w428:dbl)
                    n257 = Divide(x="PERIOD", y=w428) -> (x/y=w431:dbl)
                    n258 = Divide(x="IDL_WID2", y=w428) -> (x/y=w492:dbl)
                    n259 = Divide(x="RST_OFF", y=w428) -> (x/y=w441:dbl)
                    n260 = Divide(x="RST_WID", y=w428) -> (x/y=w442:dbl)
                    n261 = Divide(x="READ_OFF", y=w428) -> (x/y=w448:dbl)
                    n262 = Divide(x="READ_WID", y=w428) -> (x/y=w451:dbl)
                    n263 = Divide(x="IDXM_OFF", y=w428) -> (x/y=w449:dbl)
                    n264 = Divide(x="IDXM_WID", y=w428) -> (x/y=w450:dbl)
                    n265 = Divide(x="IDXL_OFF", y=w428) -> (x/y=w456:dbl)
                    n266 = Divide(x="IDXL_WID", y=w428) -> (x/y=w455:dbl)
                    n267 = Divide(x="IDL_OFF1", y=w428) -> (x/y=w487:dbl)
                    n268 = Divide(x="IDL_WID1", y=w428) -> (x/y=w483:dbl)
                    n269 = Divide(x="IDL_OFF2", y=w428) -> (x/y=w490:dbl)
                    n270 = Initialize Array(FALSE, w431) -> (w503:bool[])
                    n271 = Initialize Array(TRUE, w442) -> (w444:bool[])
                    n272 = Initialize Array(TRUE, w492) -> (w489:bool[])
                    n273 = Initialize Array(TRUE, w455) -> (w447:bool[])
                    n274 = Initialize Array(TRUE, w483) -> (w488:bool[])
                    n275 = Initialize Array(TRUE, w450) -> (w446:bool[])
                    n276 = Initialize Array(TRUE, w451) -> (w445:bool[])
                    n277 = Replace Array Subset(array=w503, new element=w444, index=w441) -> (w458:bool[])
                    n278 = Replace Array Subset(array=w503, new element=w447, index=w456) -> (w466:bool[])
                    n279 = Replace Array Subset(array=w503, new element=w446, index=w449) -> (w467:bool[])
                    n280 = Replace Array Subset(array=w503, new element=w445, index=w448) -> (w468:bool[])
                    n281 = Replace Array Subset(array=w503, new element=w488, index=w487) -> (w495:bool[])
                    n282 = Replace Array Subset(array=w495, new element=w489, index=w490) -> (w496:bool[])
                    n283 = Not(x=w466) -> (.not. x?=w465:bool[])
                    n284 = Not(x=w468) -> (.not. x?=w461:bool[])
                    n285 = Not(x=w467) -> (.not. x?=w462:bool[])
                    n286 = Not(x=w458) -> (.not. x?=w457:bool[])
                    n287 = Not(x=w496) -> (.not. x?=w481:bool[])
                    n288 = Select(t=w465, s="I_IDXL", f=w466) -> (s? t:f=w473:bool[])
                    n289 = Select(t=w461, s="I_READ", f=w468) -> (s? t:f=w469:bool[])
                    n290 = Select(t=w462, s="I_IDXM", f=w467) -> (s? t:f=w472:bool[])
                    n291 = Select(t=w457, s="I_RST", f=w458) -> (s? t:f=w480:bool[])
                    n292 = Select(t=w481, s="I_IDL", f=w496) -> (s? t:f=w497:bool[])
                    n293 = Build Array(w480, w469, w472, w473, w497) -> (w470:bool[][])
                    n294 = local read "I_IDXL"() -> (w479:bool)
                    n295 = local read "I_READ"() -> (w477:bool)
                    n296 = local read "I_IDXM"() -> (w478:bool)
                    n297 = local read "I_RST"() -> (w476:bool)
                    n298 = local read "I_IDL"() -> (w498:bool)
                    n299 = Transpose 2D Array(2D array=w470) -> (transposed array=w471:bool[][])
                    n300 = call-poly <vilib>:"Boolean Array to Digital.vi"("boolean array"=w471) -> ("digital data"=w430:digitaldata)  [unwired: 9 in, 1 out]
                    n301 = Build Array(w476, w477, w478, w479, w498, "CLOCK DISABLE") -> (w425:bool[])
                    n302 = Divide(x="CLOCK", y="MULT") -> (x/y=→"CLOCK 2":dbl)
                    n303 = Boolean Array To Number(Boolean array=w425) -> (number=w424:u32)
                    n304 = To Unsigned Byte Integer(number=w424) -> (unsigned 8bit integer=w423:u8)
                    n305 = call-poly <vilib>:"Append Digital Samples.vi"("digital data B"=w430, "digital data A"=w430) -> ("digital data out"=→"Mixed Signal Graph":digitaldata)  [unwired: 8 in, 1 out]
                    n306 = Join Numbers(hi=w423, lo=w423) -> ((hi.lo)=w422:u16)
                    n307 = Join Numbers(hi=w422, lo=w422) -> ((hi.lo)=→"INV_REG":u32)
                    n308 = case shown="True" "OK Button 4" {
                      tunnel: "CLOCK DISABLE" -> [_ w506]
                      frame False {
                      }
                      frame True {
                        n309 = stacked-sequence {
                          frame #0 {
                            n310 = local read "READ_WID"() -> (w543:dbl)
                            n311 = local read "IDL_WID2"() -> (w535:dbl)
                            n312 = local read "RST_WID"() -> (w556:dbl)
                            n313 = local read "READ_OFF"() -> (w542:dbl)
                            n314 = local read "IDXM_WID"() -> (w545:dbl)
                            n315 = local read "IDL_OFF2"() -> (w536:dbl)
                            n316 = local read "IDL_WID1"() -> (w537:dbl)
                            n317 = local read "IDXM_OFF"() -> (w544:dbl)
                            n318 = local read "IDL_OFF1"() -> (w538:dbl)
                            n319 = local read "CLOCK 2"() -> (w534:dbl)
                            n320 = local read "RST_OFF"() -> (w557:dbl)
                            n321 = local read "IDXL_OFF"() -> (w546:dbl)
                            n322 = local read "IDXL_WID"() -> (w547:dbl)
                            n323 = Divide(x=w557, y=w534) -> (x/y=w548:dbl)
                            n324 = Divide(x=w556, y=w534) -> (x/y=w549:dbl)
                            n325 = Divide(x=w542, y=w534) -> (x/y=w550:dbl)
                            n326 = Divide(x=w544, y=w534) -> (x/y=w555:dbl)
                            n327 = Divide(x=w546, y=w534) -> (x/y=w553:dbl)
                            n328 = Divide(x=w543, y=w534) -> (x/y=w551:dbl)
                            n329 = Divide(x=w545, y=w534) -> (x/y=w552:dbl)
                            n330 = Divide(x=w547, y=w534) -> (x/y=w554:dbl)
                            n331 = Divide(x=w538, y=w534) -> (x/y=w540:dbl)
                            n332 = Divide(x=w537, y=w534) -> (x/y=w541:dbl)
                            n333 = Divide(x=w536, y=w534) -> (x/y=w539:dbl)
                            n334 = Divide(x=w535, y=w534) -> (x/y=w533:dbl)
                            n335 = To Unsigned Word Integer(number=w548) -> (unsigned 16bit integer=w531:u16)
                            n336 = To Unsigned Word Integer(number=w550) -> (unsigned 16bit integer=w530:u16)
                            n337 = To Unsigned Word Integer(number=w552) -> (unsigned 16bit integer=w527:u16)
                            n338 = To Unsigned Word Integer(number=w549) -> (unsigned 16bit integer=w532:u16)
                            n339 = To Unsigned Word Integer(number=w553) -> (unsigned 16bit integer=w526:u16)
                            n340 = To Unsigned Word Integer(number=w551) -> (unsigned 16bit integer=w529:u16)
                            n341 = To Unsigned Word Integer(number=w554) -> (unsigned 16bit integer=w525:u16)
                            n342 = To Unsigned Word Integer(number=w555) -> (unsigned 16bit integer=w528:u16)
                            n343 = To Unsigned Word Integer(number=w540) -> (unsigned 16bit integer=w524:u16)
                            n344 = To Unsigned Word Integer(number=w541) -> (unsigned 16bit integer=w523:u16)
                            n345 = To Unsigned Word Integer(number=w533) -> (unsigned 16bit integer=w521:u16)
                            n346 = To Unsigned Word Integer(number=w539) -> (unsigned 16bit integer=w522:u16)
                            n347 = Join Numbers(hi=w532, lo=w531) -> ((hi.lo)=w520:u32)
                            n348 = Join Numbers(hi=w525, lo=w526) -> ()  [unwired: 1 out]
                            n349 = Join Numbers(hi=w529, lo=w530) -> ((hi.lo)=w510:u32)
                            n350 = Join Numbers(hi=w523, lo=w524) -> ((hi.lo)=w514:u32)
                            n351 = Join Numbers(hi=w527, lo=w528) -> ((hi.lo)=w511:u32)
                            n352 = Join Numbers(hi=w521, lo=w522) -> ((hi.lo)=w512:u32)
                            n353 = call "UDP_WR.vi"("DATA"=w520, "ADDRESS"=u16 11 ("address")) -> ()  [unwired: 1 out]
                            n354 = call "UDP_WR.vi"("ADDRESS"=u16 14 ("address")) -> ()  [unwired: 1 in, 1 out]
                            n355 = call "UDP_WR.vi"("DATA"=w514, "ADDRESS"=u16 15 ("address")) -> ()  [unwired: 1 out]
                            n356 = call "UDP_WR.vi"("DATA"=w512, "ADDRESS"=u16 16 ("address")) -> ()  [unwired: 1 out]
                            n357 = call "UDP_WR.vi"("DATA"=w510, "ADDRESS"=u16 12 ("address")) -> ()  [unwired: 1 out]
                            n358 = call "UDP_WR.vi"("DATA"=w511, "ADDRESS"=u16 13 ("address")) -> ()  [unwired: 1 out]
                          }
                          frame #1 {
                            n359 = local read "READ_WID"() -> (w591:dbl)
                            n360 = local read "IDL_WID2"() -> (w583:dbl)
                            n361 = local read "RST_WID"() -> (w604:dbl)
                            n362 = local read "READ_OFF"() -> (w590:dbl)
                            n363 = local read "IDXM_WID"() -> (w593:dbl)
                            n364 = local read "IDL_OFF2"() -> (w584:dbl)
                            n365 = local read "IDL_WID1"() -> (w585:dbl)
                            n366 = local read "IDXM_OFF"() -> (w592:dbl)
                            n367 = local read "IDL_OFF1"() -> (w586:dbl)
                            n368 = local read "CLOCK 2"() -> (w582:dbl)
                            n369 = local read "RST_OFF"() -> (w605:dbl)
                            n370 = local read "IDXL_OFF"() -> (w594:dbl)
                            n371 = local read "IDXL_WID"() -> (w595:dbl)
                            n372 = Divide(x=w605, y=w582) -> (x/y=w596:dbl)
                            n373 = Divide(x=w604, y=w582) -> (x/y=w597:dbl)
                            n374 = Divide(x=w590, y=w582) -> (x/y=w598:dbl)
                            n375 = Divide(x=w592, y=w582) -> (x/y=w603:dbl)
                            n376 = Divide(x=w594, y=w582) -> (x/y=w601:dbl)
                            n377 = Divide(x=w591, y=w582) -> (x/y=w599:dbl)
                            n378 = Divide(x=w593, y=w582) -> (x/y=w600:dbl)
                            n379 = Divide(x=w595, y=w582) -> (x/y=w602:dbl)
                            n380 = Divide(x=w586, y=w582) -> (x/y=w588:dbl)
                            n381 = Divide(x=w585, y=w582) -> (x/y=w589:dbl)
                            n382 = Divide(x=w584, y=w582) -> (x/y=w587:dbl)
                            n383 = Divide(x=w583, y=w582) -> (x/y=w581:dbl)
                            n384 = To Unsigned Word Integer(number=w596) -> (unsigned 16bit integer=w579:u16)
                            n385 = To Unsigned Word Integer(number=w598) -> (unsigned 16bit integer=w578:u16)
                            n386 = To Unsigned Word Integer(number=w600) -> (unsigned 16bit integer=w575:u16)
                            n387 = To Unsigned Word Integer(number=w597) -> (unsigned 16bit integer=w580:u16)
                            n388 = To Unsigned Word Integer(number=w601) -> (unsigned 16bit integer=w574:u16)
                            n389 = To Unsigned Word Integer(number=w599) -> (unsigned 16bit integer=w577:u16)
                            n390 = To Unsigned Word Integer(number=w602) -> (unsigned 16bit integer=w573:u16)
                            n391 = To Unsigned Word Integer(number=w603) -> (unsigned 16bit integer=w576:u16)
                            n392 = To Unsigned Word Integer(number=w588) -> (unsigned 16bit integer=w572:u16)
                            n393 = To Unsigned Word Integer(number=w589) -> (unsigned 16bit integer=w571:u16)
                            n394 = To Unsigned Word Integer(number=w581) -> (unsigned 16bit integer=w569:u16)
                            n395 = To Unsigned Word Integer(number=w587) -> (unsigned 16bit integer=w570:u16)
                            n396 = Join Numbers(hi=w580, lo=w579) -> ((hi.lo)=w568:u32)
                            n397 = Join Numbers(hi=w573, lo=w574) -> ()  [unwired: 1 out]
                            n398 = Join Numbers(hi=w577, lo=w578) -> ((hi.lo)=w558:u32)
                            n399 = Join Numbers(hi=w571, lo=w572) -> ((hi.lo)=w562:u32)
                            n400 = Join Numbers(hi=w575, lo=w576) -> ((hi.lo)=w559:u32)
                            n401 = Join Numbers(hi=w569, lo=w570) -> ((hi.lo)=w560:u32)
                            n402 = call "UDP_WR.vi"("DATA"=w568, "ADDRESS"=u16 20 ("address")) -> ()  [unwired: 1 out]
                            n403 = call "UDP_WR.vi"("ADDRESS"=u16 23 ("address")) -> ()  [unwired: 1 in, 1 out]
                            n404 = call "UDP_WR.vi"("DATA"=w562, "ADDRESS"=u16 24 ("address")) -> ()  [unwired: 1 out]
                            n405 = call "UDP_WR.vi"("DATA"=w560, "ADDRESS"=u16 25 ("address")) -> ()  [unwired: 1 out]
                            n406 = call "UDP_WR.vi"("DATA"=w558, "ADDRESS"=u16 21 ("address")) -> ()  [unwired: 1 out]
                            n407 = call "UDP_WR.vi"("DATA"=w559, "ADDRESS"=u16 22 ("address")) -> ()  [unwired: 1 out]
                          }
                          frame #2 {
                            n408 = local read "READ_WID"() -> (w639:dbl)
                            n409 = local read "IDL_WID2"() -> (w631:dbl)
                            n410 = local read "RST_WID"() -> (w652:dbl)
                            n411 = local read "READ_OFF"() -> (w638:dbl)
                            n412 = local read "IDXM_WID"() -> (w641:dbl)
                            n413 = local read "IDL_OFF2"() -> (w632:dbl)
                            n414 = local read "IDL_WID1"() -> (w633:dbl)
                            n415 = local read "IDXM_OFF"() -> (w640:dbl)
                            n416 = local read "IDL_OFF1"() -> (w634:dbl)
                            n417 = local read "CLOCK 2"() -> (w630:dbl)
                            n418 = local read "RST_OFF"() -> (w653:dbl)
                            n419 = local read "IDXL_OFF"() -> (w642:dbl)
                            n420 = local read "IDXL_WID"() -> (w643:dbl)
                            n421 = Divide(x=w653, y=w630) -> (x/y=w644:dbl)
                            n422 = Divide(x=w652, y=w630) -> (x/y=w645:dbl)
                            n423 = Divide(x=w638, y=w630) -> (x/y=w646:dbl)
                            n424 = Divide(x=w640, y=w630) -> (x/y=w651:dbl)
                            n425 = Divide(x=w642, y=w630) -> (x/y=w649:dbl)
                            n426 = Divide(x=w639, y=w630) -> (x/y=w647:dbl)
                            n427 = Divide(x=w641, y=w630) -> (x/y=w648:dbl)
                            n428 = Divide(x=w643, y=w630) -> (x/y=w650:dbl)
                            n429 = Divide(x=w634, y=w630) -> (x/y=w636:dbl)
                            n430 = Divide(x=w633, y=w630) -> (x/y=w637:dbl)
                            n431 = Divide(x=w632, y=w630) -> (x/y=w635:dbl)
                            n432 = Divide(x=w631, y=w630) -> (x/y=w629:dbl)
                            n433 = To Unsigned Word Integer(number=w644) -> (unsigned 16bit integer=w627:u16)
                            n434 = To Unsigned Word Integer(number=w646) -> (unsigned 16bit integer=w626:u16)
                            n435 = To Unsigned Word Integer(number=w648) -> (unsigned 16bit integer=w623:u16)
                            n436 = To Unsigned Word Integer(number=w645) -> (unsigned 16bit integer=w628:u16)
                            n437 = To Unsigned Word Integer(number=w649) -> (unsigned 16bit integer=w622:u16)
                            n438 = To Unsigned Word Integer(number=w647) -> (unsigned 16bit integer=w625:u16)
                            n439 = To Unsigned Word Integer(number=w650) -> (unsigned 16bit integer=w621:u16)
                            n440 = To Unsigned Word Integer(number=w651) -> (unsigned 16bit integer=w624:u16)
                            n441 = To Unsigned Word Integer(number=w636) -> (unsigned 16bit integer=w620:u16)
                            n442 = To Unsigned Word Integer(number=w637) -> (unsigned 16bit integer=w619:u16)
                            n443 = To Unsigned Word Integer(number=w629) -> (unsigned 16bit integer=w617:u16)
                            n444 = To Unsigned Word Integer(number=w635) -> (unsigned 16bit integer=w618:u16)
                            n445 = Join Numbers(hi=w628, lo=w627) -> ((hi.lo)=w616:u32)
                            n446 = Join Numbers(hi=w621, lo=w622) -> ()  [unwired: 1 out]
                            n447 = Join Numbers(hi=w625, lo=w626) -> ((hi.lo)=w606:u32)
                            n448 = Join Numbers(hi=w619, lo=w620) -> ((hi.lo)=w610:u32)
                            n449 = Join Numbers(hi=w623, lo=w624) -> ((hi.lo)=w607:u32)
                            n450 = Join Numbers(hi=w617, lo=w618) -> ((hi.lo)=w608:u32)
                            n451 = call "UDP_WR.vi"("DATA"=w616, "ADDRESS"=u16 29 ("address")) -> ()  [unwired: 1 out]
                            n452 = call "UDP_WR.vi"("ADDRESS"=u16 32 ("address")) -> ()  [unwired: 1 in, 1 out]
                            n453 = call "UDP_WR.vi"("DATA"=w610, "ADDRESS"=u16 33 ("address")) -> ()  [unwired: 1 out]
                            n454 = call "UDP_WR.vi"("DATA"=w608, "ADDRESS"=u16 34 ("address")) -> ()  [unwired: 1 out]
                            n455 = call "UDP_WR.vi"("DATA"=w606, "ADDRESS"=u16 30 ("address")) -> ()  [unwired: 1 out]
                            n456 = call "UDP_WR.vi"("DATA"=w607, "ADDRESS"=u16 31 ("address")) -> ()  [unwired: 1 out]
                          }
                          frame #3 {
                            n457 = local read "READ_WID"() -> (w687:dbl)
                            n458 = local read "IDL_WID2"() -> (w679:dbl)
                            n459 = local read "RST_WID"() -> (w700:dbl)
                            n460 = local read "READ_OFF"() -> (w686:dbl)
                            n461 = local read "IDXM_WID"() -> (w689:dbl)
                            n462 = local read "IDL_OFF2"() -> (w680:dbl)
                            n463 = local read "IDL_WID1"() -> (w681:dbl)
                            n464 = local read "IDXM_OFF"() -> (w688:dbl)
                            n465 = local read "IDL_OFF1"() -> (w682:dbl)
                            n466 = local read "CLOCK 2"() -> (w678:dbl)
                            n467 = local read "RST_OFF"() -> (w701:dbl)
                            n468 = local read "IDXL_OFF"() -> (w690:dbl)
                            n469 = local read "IDXL_WID"() -> (w691:dbl)
                            n470 = Divide(x=w701, y=w678) -> (x/y=w692:dbl)
                            n471 = Divide(x=w700, y=w678) -> (x/y=w693:dbl)
                            n472 = Divide(x=w686, y=w678) -> (x/y=w694:dbl)
                            n473 = Divide(x=w688, y=w678) -> (x/y=w699:dbl)
                            n474 = Divide(x=w690, y=w678) -> (x/y=w697:dbl)
                            n475 = Divide(x=w687, y=w678) -> (x/y=w695:dbl)
                            n476 = Divide(x=w689, y=w678) -> (x/y=w696:dbl)
                            n477 = Divide(x=w691, y=w678) -> (x/y=w698:dbl)
                            n478 = Divide(x=w682, y=w678) -> (x/y=w684:dbl)
                            n479 = Divide(x=w681, y=w678) -> (x/y=w685:dbl)
                            n480 = Divide(x=w680, y=w678) -> (x/y=w683:dbl)
                            n481 = Divide(x=w679, y=w678) -> (x/y=w677:dbl)
                            n482 = To Unsigned Word Integer(number=w692) -> (unsigned 16bit integer=w675:u16)
                            n483 = To Unsigned Word Integer(number=w694) -> (unsigned 16bit integer=w674:u16)
                            n484 = To Unsigned Word Integer(number=w696) -> (unsigned 16bit integer=w671:u16)
                            n485 = To Unsigned Word Integer(number=w693) -> (unsigned 16bit integer=w676:u16)
                            n486 = To Unsigned Word Integer(number=w697) -> (unsigned 16bit integer=w670:u16)
                            n487 = To Unsigned Word Integer(number=w695) -> (unsigned 16bit integer=w673:u16)
                            n488 = To Unsigned Word Integer(number=w698) -> (unsigned 16bit integer=w669:u16)
                            n489 = To Unsigned Word Integer(number=w699) -> (unsigned 16bit integer=w672:u16)
                            n490 = To Unsigned Word Integer(number=w684) -> (unsigned 16bit integer=w668:u16)
                            n491 = To Unsigned Word Integer(number=w685) -> (unsigned 16bit integer=w667:u16)
                            n492 = To Unsigned Word Integer(number=w677) -> (unsigned 16bit integer=w665:u16)
                            n493 = To Unsigned Word Integer(number=w683) -> (unsigned 16bit integer=w666:u16)
                            n494 = Join Numbers(hi=w676, lo=w675) -> ((hi.lo)=w664:u32)
                            n495 = Join Numbers(hi=w669, lo=w670) -> ()  [unwired: 1 out]
                            n496 = Join Numbers(hi=w673, lo=w674) -> ((hi.lo)=w654:u32)
                            n497 = Join Numbers(hi=w667, lo=w668) -> ((hi.lo)=w658:u32)
                            n498 = Join Numbers(hi=w671, lo=w672) -> ((hi.lo)=w655:u32)
                            n499 = Join Numbers(hi=w665, lo=w666) -> ((hi.lo)=w656:u32)
                            n500 = call "UDP_WR.vi"("DATA"=w664, "ADDRESS"=u16 38 ("address")) -> ()  [unwired: 1 out]
                            n501 = call "UDP_WR.vi"("ADDRESS"=u16 41 ("address")) -> ()  [unwired: 1 in, 1 out]
                            n502 = call "UDP_WR.vi"("DATA"=w658, "ADDRESS"=u16 42 ("address")) -> ()  [unwired: 1 out]
                            n503 = call "UDP_WR.vi"("DATA"=w656, "ADDRESS"=u16 43 ("address")) -> ()  [unwired: 1 out]
                            n504 = call "UDP_WR.vi"("DATA"=w654, "ADDRESS"=u16 39 ("address")) -> ()  [unwired: 1 out]
                            n505 = call "UDP_WR.vi"("DATA"=w655, "ADDRESS"=u16 40 ("address")) -> ()  [unwired: 1 out]
                          }
                        }
                        n506 = local read "INV_REG"() -> (w505:u32)
                        n507 = call "UDP_WR.vi"("DATA"=w505, "ADDRESS"=u16 10) -> ()  [unwired: 1 out]
                        n508 = Select(t=T10."Disabled and Grayed Out" ("Disabled"), s=w506, f=T10."Enabled" ("Disabled")) -> (s? t:f=w509:T10)
                        n509 = property on="Mixed Signal Graph" class="MixedGraph (strict)"("DisabledEnum"=w509) -> ()  [unwired: 2 in, 2 out]
                      }
                    }
                  }
                }
              }
            }
            n510 = Wait Until Next ms Multiple(millisecond multiple=u32 10) -> ()  [unwired: 1 out]
            n511 = case shown="True" "SAVE TO \nFILE" {
              frame False {
              }
              frame True {
                n512 = local read "Store_Data"() -> (w702:bool)
                n513 = case shown="False" w702 {
                  frame False {
                    n514 = stacked-sequence {
                      seq-local: [w704 _] -> [_ w716]
                      seq-local: [w703 _] -> [_ w715]
                      frame #0 {
                        n515 = Concatenate Strings("FILE NAME 2", ".txt" ("string")) -> (w706:string)
                        n516 = Build Path(base path="FILE PATH", name or relative path=w706) -> (appended path=w704:path)
                        n517 = call <vilib>:"Check if File or Folder Exists.vi"("path"=w704) -> ("file or folder exists?"=w707:bool)  [unwired: 8 in, 2 out]
                        n518 = case shown="False" w707 {
                          tunnel: [TRUE ("T button?") w713] -> w703
                          frame False {
                          }
                          frame True {
                            n519 = Two Button Dialog(message="FILE EXISTS DO YOU \nWANT TO OVERWRITE", 1:"NO" ("F button name (\"Cancel\")"), 2:"YES" ("T button name (\"OK\")")) -> (T button?=w713:bool)
                          }
                        }
                      }
                      frame #1 {
                        n520 = Path To String(path=w716) -> (string=w717:string)
                        n521 = case shown="True" w715 {
                          tunnel: w717 -> [_ w719]
                          frame False {
                          }
                          frame True {
                            n522 = global read "WIB_Global.vi" "WIB_DLL_REF"() -> (w718:refnum<k24>)
                            n523 = invoke class="WIB_COMM" method="open_file"(reference=w718, "File_name"=w719) -> ()  [unwired: 2 in, 4 out]
                          }
                        }
                      }
                    }
                  }
                  frame True {
                    n524 = global read "WIB_Global.vi" "WIB_DLL_REF"() -> (w720:refnum<k24>)
                    n525 = invoke class="WIB_COMM" method="open_file"(reference=w720, "File_name"="") -> ()  [unwired: 2 in, 4 out]
                  }
                }
              }
            }
            n526 = global read "WIB_Global.vi" "WIB_DLL_REF"() -> (w66:refnum<k24>)
            n527 = property class="WIB_COMM"(reference=w66) -> ("Store_Data"=→"Store_Data":bool)  [unwired: 1 in, 2 out]
          }
          frame "ADC POWER" {
            n528 = case shown="True" "Boolean" {
              selector: "Boolean" -> [w723 w735]
              tunnel: [w723 w735] -> _
              frame False {
              }
              frame True {
                n529 = for {
                  N: 6 -> [_]
                  tunnel: [w749] -> w737 mode=indexing
                  tunnel: [w746] -> w724 mode=indexing
                  i -> [w751]
                  n530 = for {
                    N: 2 -> [_]
                    tunnel: [w758] -> w748 mode=indexing
                    tunnel: w751 -> [w761]
                    tunnel: [w753] -> w747 mode=indexing
                    i -> [w759]
                    n531 = Add(x=w761, y=u16 64 ("DEVICE_ADDR 4")) -> (x+y=w757:i32)
                    n532 = Add(x=u8 1 ("ADDRESS 6"), y=w759) -> (x+y=w755:i32)
                    n533 = call "RD_I2C_CT_ADC_SKT2-3.vi"("READ address"=w755, "NUM_BYTES"=u8 2 ("BYTES 3"), "DEV address 2"=w757) -> ("DATA 7"=w754:u32, "DATA 8"=w752:u32)
                    n534 = Swap Bytes(anything=w752) -> (byte swapped=w758:u32)
                    n535 = Swap Bytes(anything=w754) -> (byte swapped=w753:u32)
                  }
                  n536 = To Word Integer(number=w747) -> (16bit integer=w746:i16[])
                  n537 = To Word Integer(number=w748) -> (16bit integer=w749:i16[])
                }
                n538 = Transpose 2D Array(2D array=w737) -> (transposed array=w742:i16[][])
                n539 = Transpose 2D Array(2D array=w724) -> (transposed array=w727:i16[][])
                n540 = Index Array(array=w742, index (row)=1) -> (element=w741:i16[])  [unwired: 1 in]
                n541 = Index Array(array=w742, index (row)=0) -> (element=w738:i16[])  [unwired: 1 in]
                n542 = Multiply(x=w741, y=0.00125) -> (x*y=→"BUS VOL":dbl[])
                n543 = Multiply(x=w738, y=2.5e-06) -> (x*y=→"SHUNT VOL":dbl[])
                n544 = Index Array(array=w727, index (row)=1) -> (element=w728:i16[])  [unwired: 1 in]
                n545 = Index Array(array=w727, index (row)=0) -> (element=w731:i16[])  [unwired: 1 in]
                n546 = Multiply(x=w728, y=0.00125) -> (x*y=→"BUS VOL 2":dbl[])
                n547 = Multiply(x=w731, y=2.5e-06) -> (x*y=→"SHUNT VOL 2":dbl[])
              }
            }
          }
          frame "ASIC SPI" {
            n548 = Wait Until Next ms Multiple(millisecond multiple=u32 10) -> ()  [unwired: 1 out]
            n549 = stacked-sequence {
              frame #0 {
                n550 = for {
                  N: 4 ("NUMBER OF ASICS") -> [_]
                  shift-right: [w807] -> w766
                  shift-left: bool[] [] -> [w806]
                  i -> [w771]
                  n551 = Index Array(array="CHANNEL 3", index (col)=w771) -> (element=w804:T11)  [unwired: 1 in]
                  n552 = Reverse 1D Array(array=w804) -> (reversed array=w808:T11)
                  n553 = for {
                    tunnel: w808 -> [w822] mode=indexing
                    shift-right: [w818] -> w770
                    shift-left: bool[] [] -> [w812]
                    n554 = Unbundle By Name(w822) -> ("tst"=w810:bool, "slp"=w811:bool, "PDSR"=w817:bool, "PCSR"=w816:bool, "D_offset"=w815:u16)
                    n555 = Number To Boolean Array(number=w815) -> (Boolean array=w821:bool[])
                    n556 = Array Subset(array=w821, index=0, length=4) -> (w814:bool[])
                    n557 = Reverse 1D Array(array=w814) -> (reversed array=w813:bool[])
                    n558 = Build Array (concatenate)(w812, w810, w811, w817, w816, w813) -> (w818:bool[])
                  }
                  n559 = Select(t=0, s="GLOBAL \nALL SAME", f=w771) -> (s? t:f=w774:i32)
                  n560 = Index Array(array="Array 4", index=w774) -> (element=w799:T12)
                  n561 = Unbundle By Name(w799) -> ("sLSB"=w777:u16, "F5  TEST DATA"=w790:u16, "F4 pipeline select"=w791:u16, "F3"=w792:u16, "F2"=w793:u16, "F1"=w794:u16, "F0"=w795:u16, "EN_GR"=w796:u16, "FRQC"=w797:u16, "CLKG"=w798:u16)
                  n562 = Number To Boolean Array(number=w798) -> (Boolean array=w801:bool[])
                  n563 = Not Equal To 0?(x=w792) -> (x != 0?=w782:bool)
                  n564 = Not Equal To 0?(x=w793) -> (x != 0?=w783:bool)
                  n565 = Not Equal To 0?(x=w790) -> (x != 0?=w780:bool)
                  n566 = Not Equal To 0?(x=w791) -> (x != 0?=w781:bool)
                  n567 = Not Equal To 0?(x=w794) -> (x != 0?=w784:bool)
                  n568 = Not Equal To 0?(x=w795) -> (x != 0?=w785:bool)
                  n569 = Not Equal To 0?(x=w796) -> (x != 0?=w786:bool)
                  n570 = Not Equal To 0?(x=w797) -> (x != 0?=w787:bool)
                  n571 = Not Equal To 0?(x=w777) -> (x != 0?=w776:bool)
                  n572 = Index Array(array=w801, index=1) -> (element=w788:bool)
                  n573 = Index Array(array=w801, index=0) -> (element=w789:bool)
                  n574 = Initialize Array(FALSE ("x != 0?"), 5 ("dimension size")) -> (w775:bool[])
                  n575 = Build Array (concatenate)(w775, w776, w780, w781, w782, w783, w784, w785, w786, w787, w788, w789) -> (w769:bool[])
                  n576 = Build Array (concatenate)(w806, w770, w769) -> (w807:bool[])
                }
                "ADC ARRAY" <- w766
                n577 = Array Size(array=w766) -> (size(s)=→"size(s)":i32)
              }
              frame #1 {
                n578 = for {
                  N: 1 -> [_]
                  shift-right: [w846] -> w824
                  shift-left: bool[] [] -> [w844]
                  w842 = FALSE ("SLK 2")
                  n579 = Index Array(array="Array 3", index (col)=0 ("disabled index (col)")) -> (element=w847:T13)  [unwired: 1 in]
                  n580 = for {
                    tunnel: w847 -> [w873] mode=indexing
                    shift-right: [w869] -> w853
                    shift-left: bool[] [] -> [w870]
                    n581 = Unbundle By Name(w873) -> ("sts"=w872:bool, "snc"=w871:bool, "SG"=w862:u16, "ST"=w861:u16, "SDC"=w858:bool, "SDF"=w857:bool)
                    n582 = Number To Boolean Array(number=w862) -> (Boolean array=w868:bool[])
                    n583 = Number To Boolean Array(number=w861) -> (Boolean array=w863:bool[])
                    n584 = Array Subset(array=w868, index=0, length=2) -> (w860:bool[])
                    n585 = Array Subset(array=w863, index=0, length=2) -> (w859:bool[])
                    n586 = Build Array (concatenate)(w870, w872, w871, w860, w859, w858, w857) -> (w869:bool[])
                  }
                  n587 = Number To Boolean Array(number="STB") -> (Boolean array=w849:bool[])
                  n588 = Number To Boolean Array(number="DAC  0x00-0x3f") -> (Boolean array=w836:bool[])
                  n589 = Array Subset(array=w849, index=0, length=2) -> (w855:bool[])
                  n590 = Array Subset(array=w836, index=0, length=6) -> (w833:bool[])
                  n591 = Number To Boolean Array(number="DAC") -> (Boolean array=w832:bool[])
                  n592 = Reverse 1D Array(array=w853) -> (reversed array=w841:bool[])
                  n593 = Reverse 1D Array(array=w855) -> (reversed array=w856:bool[])
                  n594 = Reverse 1D Array(array=w833) -> (reversed array=w828:bool[])
                  n595 = Array Subset(array=w832, index=0, length=2) -> (w829:bool[])
                  n596 = Build Array (concatenate)(w829, w828) -> (w840:bool[])
                  n597 = Build Array (concatenate)(w841, "SLK", w856, w842, "SLK 2", w842, w842, w842, w840) -> (w845:bool[])
                  n598 = Build Array (concatenate)(w844, w845) -> (w846:bool[])
                }
                "FE ARRAY" <- w824
                n599 = Array Size(array=w824) -> (size(s)=→"size(s) 2":i32)
              }
              frame #2 {
                n600 = for {
                  N: 4 -> [_]
                  tunnel: [w885] -> w879 mode=indexing
                  tunnel: [w882] -> w874
                  i -> [w894]
                  n601 = local read "FE ARRAY"() -> (w887:bool[])
                  n602 = Select(t=0, s="ALL SAME", f=144 ("length")) -> (s? t:f=w892:i32)
                  n603 = local read "ADC ARRAY"() -> (w888:bool[])
                  n604 = Multiply(x=w892, y=w894) -> (x*y=w893:i32)
                  n605 = Array Subset(array=w887, index=0, length=144) -> (w883:bool[])
                  n606 = Array Subset(array=w888, index=w893, length=144) -> (w886:bool[])
                  n607 = for {
                    N: 5 -> [_]
                    tunnel: w886 -> [w909]
                    tunnel: [w904] -> w885 mode=indexing
                    i -> [w908]
                    w907 = 32 ("length")
                    n608 = Multiply(x=w907, y=w908) -> (x*y=w906:i32)
                    n609 = Array Subset(array=w909, index=w906, length=w907) -> (w905:bool[])
                    n610 = Boolean Array To Number(Boolean array=w905) -> (number=w904:u32)
                  }
                  n611 = for {
                    N: 5 -> [_]
                    tunnel: w883 -> [w903]
                    tunnel: [w898] -> w882 mode=indexing
                    i -> [w902]
                    w901 = 32 ("length")
                    n612 = Multiply(x=w901, y=w902) -> (x*y=w900:i32)
                    n613 = Array Subset(array=w903, index=w900, length=w901) -> (w899:bool[])
                    n614 = Boolean Array To Number(Boolean array=w899) -> (number=w898:u32)
                  }
                }
                "FE SPI" <- w874
                n615 = Index Array(array=w879) -> (element #1=→"ADC SPI 1":u32[], element #2=→"ADC SPI 2":u32[], element #3=→"ADC SPI 3":u32[], element #4=→"ADC SPI 4":u32[])  [unwired: 8 in]
              }
              frame #3 {
                n616 = case shown="True" "write_string" {
                  frame False {
                  }
                  frame True {
                    n617 = stacked-sequence {
                      frame #0 {
                        n618 = local read "ADC SPI 4"() -> (w914:u32[])
                        n619 = local read "ADC SPI 2"() -> (w916:u32[])
                        n620 = local read "FE SPI"() -> (w913:u32[])
                        n621 = local read "ADC SPI 1"() -> (w917:u32[])
                        n622 = local read "ADC SPI 3"() -> (w915:u32[])
                        n623 = for {
                          tunnel: w917 -> [w933] mode=indexing
                          tunnel: w916 -> [w929] mode=indexing
                          tunnel: w915 -> [w930] mode=indexing
                          tunnel: w914 -> [w931] mode=indexing
                          tunnel: w913 -> [w932] mode=indexing
                          i -> [w918]
                          n624 = Add(x=u16 64 ("ADDRESS"), y=w918) -> (x+y=w927:i32)
                          n625 = Add(x=u16 69 ("ADDRESS"), y=w918) -> (x+y=w925:i32)
                          n626 = Add(x=u16 74 ("ADDRESS"), y=w918) -> (x+y=w923:i32)
                          n627 = Add(x=u16 79 ("ADDRESS"), y=w918) -> (x+y=w921:i32)
                          n628 = Add(x=u16 84 ("ADDRESS"), y=w918) -> (x+y=w919:i32)
                          n629 = call "UDP_WR.vi"("DATA"=w931, "ADDRESS"=w921) -> ()  [unwired: 1 out]
                          n630 = call "UDP_WR.vi"("DATA"=w932, "ADDRESS"=w919) -> ()  [unwired: 1 out]
                          n631 = call "UDP_WR.vi"("DATA"=w929, "ADDRESS"=w925) -> ()  [unwired: 1 out]
                          n632 = call "UDP_WR.vi"("DATA"=w930, "ADDRESS"=w923) -> ()  [unwired: 1 out]
                          n633 = call "UDP_WR.vi"("DATA"=w933, "ADDRESS"=w927) -> ()  [unwired: 1 out]
                        }
                        n634 = call "UDP_WR.vi"("DATA"=u32 0, "ADDRESS"=u16 2) -> ()  [unwired: 1 out]
                      }
                      frame #1 {
                        n635 = flat-sequence {
                          frame #0 {
                            n636 = call "UDP_WR.vi"("DATA"=u32 3, "ADDRESS"=u16 2) -> ()  [unwired: 1 out]
                          }
                          frame #1 {
                            n637 = Wait Until Next ms Multiple(millisecond multiple=u32 100) -> ()  [unwired: 1 out]
                          }
                          frame #2 {
                            n638 = call "UDP_WR.vi"("DATA"=u32 2, "ADDRESS"=u16 2) -> ()  [unwired: 1 out]
                          }
                          frame #3 {
                            n639 = Wait Until Next ms Multiple(millisecond multiple=u32 100) -> ()  [unwired: 1 out]
                          }
                          frame #4 {
                            n640 = call "UDP_WR.vi"("DATA"=u32 0, "ADDRESS"=u16 2) -> ()  [unwired: 1 out]
                          }
                        }
                      }
                      frame #2 {
                        n641 = call "UDP_RD.vi"("ADDRESS 2"=i16 2) -> ("DATA 2"=w944:u32)
                        n642 = Split Number(x=w944) -> (hi(x)=w943:u16)  [unwired: 1 out]
                        n643 = Number To Boolean Array(number=w944) -> (Boolean array=w954:bool[])
                        n644 = Split Number(x=w943) -> (hi(x)=→"SYNC":u8)  [unwired: 1 out]
                        n645 = Index Array(array=w954, index #1=16 ("index")) -> (element #1=→"ADC 1":bool, element #2=→"FE 1":bool, element #3=→"ADC 2":bool, element #4=→"FE 2":bool, element #5=→"ADC 3":bool, element #6=→"FE 3":bool, element #7=→"ADC 4":bool, element #8=→"FE 4":bool)  [unwired: 7 in]
                      }
                    }
                  }
                }
              }
              frame #4 {
                n646 = case shown="True" "OK Button 2" {
                  frame False {
                  }
                  frame True {
                    n647 = flat-sequence {
                      frame #0 {
                        n648 = call "UDP_WR.vi"("DATA"=u32 48, "ADDRESS"=u16 2) -> ()  [unwired: 1 out]
                      }
                      frame #1 {
                        n649 = call "UDP_WR.vi"("DATA"=u32 0, "ADDRESS"=u16 2) -> ()  [unwired: 1 out]
                      }
                    }
                  }
                }
                n650 = case shown="True" "OK Button 5" {
                  frame False {
                  }
                  frame True {
                    n651 = flat-sequence {
                      frame #0 {
                        n652 = call "UDP_WR.vi"("DATA"=u32 64, "ADDRESS"=u16 2) -> ()  [unwired: 1 out]
                      }
                      frame #1 {
                        n653 = call "UDP_WR.vi"("DATA"=u32 0, "ADDRESS"=u16 2) -> ()  [unwired: 1 out]
                      }
                    }
                  }
                }
              }
            }
            n654 = event shown="[3] \"PWR SCK 1\", \"PWR SCK 2\", \"PWR SCK 3\", \"PWR SCK 4\": Value Change" {
              selector: _ -> [_ _ _ _]
              dyn-events: _ -> [_ _ _ _]
              timeout: 100 -> [_ _ _ _]
              event Timeout {
                n655 = event-data() -> ()  [unwired: 1 in, 3 out]
              }
              event "Slide": Value Change {
                w966 = u8 0 ("element")
                n656 = event-data() -> ()  [unwired: 1 in, 4 out]
                n657 = Build Array(w966, "Slide") -> (w968:u8[])
                n658 = Build Array(w966, w966) -> (w967:u8[])
                n659 = Build Array("Slide") -> (w969:u8[])
                n660 = property on="Array 3" class="Arr"("Index Values"=w967) -> ()  [unwired: 2 in, 2 out]
                n661 = property on="Array 4" class="Arr (strict)"("Index Values"=w969) -> ()  [unwired: 2 in, 2 out]
                n662 = property on="CHANNEL 3" class="Arr (strict)"("Index Values"=w968) -> ()  [unwired: 2 in, 2 out]
              }
              event "QUICK SET": Value Change {
                n663 = event-data() -> ()  [unwired: 1 in, 6 out]
                n664 = local read "Array 3"() -> (w976:T7)
                n665 = local read "CHANNEL 3"() -> (w986:T5)
                n666 = local read "Slide"() -> (w981:u8)
                n667 = Index Array(array=w986, index (col)=w981) -> (element=w982:T11)  [unwired: 1 in]
                n668 = Index Array(array=w976, index (col)=0 ("disabled index (col)")) -> (element=w979:T13)  [unwired: 1 in]
                n669 = for {
                  tunnel: w982 -> [w1036] mode=indexing
                  tunnel: "CHANNEL 4" -> [w1038]
                  tunnel: [w1037] -> w984 mode=indexing
                  tunnel: w982 -> [w1035] mode=indexing
                  tunnel: "channel" -> [w1019]
                  tunnel: w979 -> [w1018] mode=indexing
                  tunnel: w979 -> [w1017] mode=indexing
                  tunnel: [w992] -> w978 mode=indexing
                  n670 = Unbundle By Name(w1038) -> ("D_offset"=w1028:u16, "PDSR"=w1027:bool, "PCSR"=w1025:bool, "slp"=w1024:bool, "tst"=w988:bool)
                  n671 = Unbundle By Name(w1035) -> ("D_offset"=w1031:u16, "PDSR"=w1030:bool, "PCSR"=w1026:bool, "slp"=w1029:bool, "tst"=w989:bool)
                  n672 = Unbundle By Name(w1019) -> ("sts"=w1004:bool, "snc"=w1003:bool, "SG"=w1002:u16, "ST"=w1001:u16, "SDC"=w1000:bool, "SDF"=w999:bool)
                  n673 = Unbundle By Name(w1018) -> ("sts"=w1016:bool, "snc"=w1015:bool, "SG"=w1014:u16, "ST"=w1013:u16, "SDC"=w1012:bool, "SDF"=w1011:bool)
                  n674 = Select(t=w1028, s="s", f=w1031) -> (s? t:f=w1034:u16)
                  n675 = Select(t=w1027, s="s 2", f=w1030) -> (s? t:f=w1033:bool)
                  n676 = Select(t=w1025, s="s 3", f=w1026) -> (s? t:f=w1032:bool)
                  n677 = Select(t=w1024, s="s 4", f=w1029) -> (s? t:f=w991:bool)
                  n678 = Select(t=w988, s="s 11", f=w989) -> (s? t:f=w990:bool)
                  n679 = Select(t=w1004, s="s 5", f=w1016) -> (s? t:f=w993:bool)
                  n680 = Select(t=w1003, s="s 6", f=w1015) -> (s? t:f=w994:bool)
                  n681 = Select(t=w1002, s="s 7", f=w1014) -> (s? t:f=w995:u16)
                  n682 = Select(t=w1001, s="s 8", f=w1013) -> (s? t:f=w996:u16)
                  n683 = Select(t=w1000, s="s 9", f=w1012) -> (s? t:f=w997:bool)
                  n684 = Select(t=w999, s="s 10", f=w1011) -> (s? t:f=w998:bool)
                  n685 = Bundle By Name(cluster=w1036, "D_offset"=w1034, "PDSR"=w1033, "PCSR"=w1032, "slp"=w991, "tst"=w990) -> (w1037:T4)
                  n686 = Bundle By Name(cluster=w1017, "sts"=w993, "snc"=w994, "SG"=w995, "ST"=w996, "SDC"=w997, "SDF"=w998) -> (w992:T3)
                }
                n687 = local read "Array 3"() -> (w975:T7)
                n688 = local read "CHANNEL 3"() -> (w985:T5)
                n689 = local read "Slide"() -> (w977:u8)
                n690 = Replace Array Subset(array=w985, new element=w984, index (col)=w977) -> (w983:T5)  [unwired: 1 in]
                n691 = Replace Array Subset(array=w975, new element=w978, index (col)=0 ("disabled index (col)")) -> (w974:T7)  [unwired: 1 in]
                n692 = local write "CHANNEL 3"(w983) -> ()
                n693 = local write "Array 3"(w974) -> ()
              }
              event "PWR SCK 1", "PWR SCK 2", "PWR SCK 3", "PWR SCK 4": Value Change {
                n694 = event-data() -> ()  [unwired: 1 in, 6 out]
                n695 = Build Array("PWR SCK 1", "PWR SCK 2", "PWR SCK 3", "PWR SCK 4") -> (w1040:bool[])
                n696 = Boolean Array To Number(Boolean array=w1040) -> (number=w1039:u32)
                "PWR_CNTRL_\nREG 1" <- w1039
                n697 = call "UDP_WR.vi"("DATA"=w1039, "ADDRESS"=u16 1) -> ()  [unwired: 1 out]
              }
            }
          }
        }
      }
    }
    frame #2 {
      n698 = flat-sequence {
        frame #0 {
        }
        frame #1 {
          n699 = Wait Until Next ms Multiple(millisecond multiple=u32 1000) -> ()  [unwired: 1 out]
        }
        frame #2 {
          n700 = global read "WIB_Global.vi" "WIB_DLL_REF"() -> (w1048:refnum<k24>)
          n701 = invoke class="WIB_COMM" method="UDP_CLEANUP"(reference=w1048) -> ("UDP_CLEANUP"=→"UDP_CLEANUP":string)  [unwired: 2 in, 2 out]
        }
        frame #3 {
          n702 = Wait Until Next ms Multiple(millisecond multiple=u32 2000) -> ()  [unwired: 1 out]
        }
        frame #4 {
          n703 = Request Deallocation(TRUE ("flag")) -> ()
        }
      }
    }
  }
